vi "GetAdjacentFips.vi"(11 "FipsIn":i32[](array[numeric])) -> (3 "FipsOut":i32[](array[numeric]))   [LabVIEW 2017]
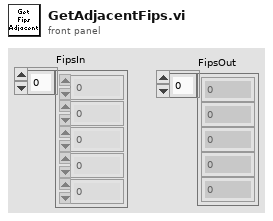
[diagram p1: front panel]
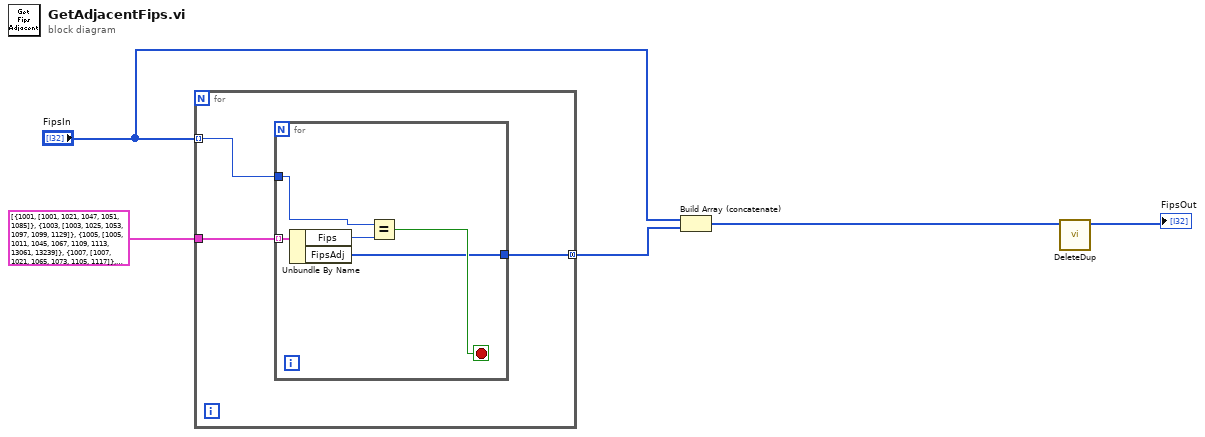
[diagram p0: block diagram]
diagram:
  n1 = for {
    tunnel: cluster{"Fips":i32, "FipsAdj":i32[]}[] [{"Fips"=1001, "FipsAdj"=[1001, 1021, 1047, 1051, 1085]}, {"Fips"=1003, "FipsAdj"=[1003, 1025, 1053, 1097, 1099, 1129]}, {"Fips"=1005, "FipsAdj"=[1005, 1011, 1045, 1067, 1109, 1113, 13061, 13239]}, {"Fips"=1007, "FipsAdj"=[1007, 1021, 1065, 1073, 1105, 1117]}, {"Fips"=1009, "FipsAdj"=[1009, 1043, 1055, 1073, 1095, 1115]}, {"Fips"=1011, "FipsAdj"=[1005, 1011, 1087, 1101, 1109]}, {"Fips"=1013, "FipsAdj"=[1013, 1035, 1039, 1041, 1085, 1099]}, {"Fips"=1015, "FipsAdj"=[1015, 1019, 1029, 1055, 1115]}, {"Fips"=1017, "FipsAdj"=[1017, 1081, 1111, 1123, 13145]}, {"Fips"=1019, "FipsAdj"=[1015, 1019, 1029, 1049, 1055, 13055, 13115]}, {"Fips"=1021, "FipsAdj"=[1001, 1007, 1021, 1037, 1047, 1051, 1105]}, {"Fips"=1023, "FipsAdj"=[1023, 1025, 1091, 1119, 1129, 28023, 28075]}, {"Fips"=1025, "FipsAdj"=[1003, 1023, 1025, 1091, 1099, 1129]}, {"Fips"=1027, "FipsAdj"=[1027, 1029, 1037, 1111, 1121]}, {"Fips"=1029, "FipsAdj"=[1015, 1019, 1027, 1029, 1111, 1121, 13045, 13143]}, {"Fips"=1031, "FipsAdj"=[1031, 1039, 1041, 1045, 1061]}, {"Fips"=1033, "FipsAdj"=[1033, 1059, 1077, 1079]}, {"Fips"=1035, "FipsAdj"=[1013, 1035, 1039, 1053]}, {"Fips"=1037, "FipsAdj"=[1021, 1027, 1037, 1051, 1117, 1121]}, {"Fips"=1039, "FipsAdj"=[1013, 1031, 1035, 1039, 1041, 1053, 1061, 12091]}, {"Fips"=1041, "FipsAdj"=[1013, 1031, 1039, 1041, 1085, 1101]}, {"Fips"=1043, "FipsAdj"=[1009, 1043, 1079, 1095, 1103, 1127]}, {"Fips"=1045, "FipsAdj"=[1005, 1031, 1045, 1061, 1067, 1069]}, {"Fips"=1047, "FipsAdj"=[1001, 1021, 1047, 1085, 1091, 1105]}, {"Fips"=1049, "FipsAdj"=[1019, 1049, 1055, 1071, 1095, 13055, 13083]}, {"Fips"=1051, "FipsAdj"=[1001, 1021, 1037, 1051, 1087, 1101]}, {"Fips"=1053, "FipsAdj"=[1003, 1035, 1039, 1053, 1099, 12033, 12091]}, {"Fips"=1055, "FipsAdj"=[1009, 1015, 1019, 1049, 1055, 1095]}, {"Fips"=1057, "FipsAdj"=[1057, 1075, 1093, 1107, 1125]}, {"Fips"=1059, "FipsAdj"=[1033, 1059, 1079, 1093, 1133, 28057]}, {"Fips"=1061, "FipsAdj"=[1031, 1039, 1045, 1061, 1069, 12059, 12063]}, {"Fips"=1063, "FipsAdj"=[1063, 1065, 1091, 1107, 1119]}, {"Fips"=1065, "FipsAdj"=[1007, 1063, 1065, 1091, 1105]}, {"Fips"=1067, "FipsAdj"=[1005, 1045, 1067, 1069, 13061]}, {"Fips"=1069, "FipsAdj"=[1045, 1061, 1067, 1069, 12063, 13099]}, {"Fips"=1071, "FipsAdj"=[1049, 1071, 1089, 1095, 13083, 47051]}, {"Fips"=1073, "FipsAdj"=[1007, 1009, 1073, 1115, 1117, 1125]}, {"Fips"=1075, "FipsAdj"=[1057, 1075, 1093, 1107, 28087]}, {"Fips"=1077, "FipsAdj"=[1033, 1077, 1079, 1083, 28141, 47055, 47071, 47099]}, {"Fips"=1079, "FipsAdj"=[1033, 1043, 1059, 1077, 1079, 1083, 1103]}, {"Fips"=1081, "FipsAdj"=[1017, 1081, 1087, 1113, 1123, 13145]}, {"Fips"=1083, "FipsAdj"=[1077, 1079, 1083, 1089, 1103, 47055]}, {"Fips"=1085, "FipsAdj"=[1001, 1013, 1041, 1047, 1085, 1101]}, {"Fips"=1087, "FipsAdj"=[1011, 1051, 1081, 1087, 1101, 1113]}, {"Fips"=1089, "FipsAdj"=[1071, 1083, 1089, 1095, 1103, 47051]}, {"Fips"=1091, "FipsAdj"=[1023, 1025, 1047, 1063, 1065, 1091, 1105, 1119]}, {"Fips"=1093, "FipsAdj"=[1057, 1059, 1075, 1093, 1127, 1133, 28057]}, {"Fips"=1095, "FipsAdj"=[1009, 1043, 1049, 1055, 1071, 1089, 1095]}, {"Fips"=1097, "FipsAdj"=[1003, 1097, 1129, 28039, 28041]}, {"Fips"=1099, "FipsAdj"=[1003, 1013, 1025, 1035, 1053, 1099]}, {"Fips"=1101, "FipsAdj"=[1001, 1011, 1041, 1051, 1085, 1087, 1101]}, {"Fips"=1103, "FipsAdj"=[1043, 1079, 1083, 1089, 1095]}, {"Fips"=1105, "FipsAdj"=[1007, 1021, 1047, 1065, 1091]}, {"Fips"=1107, "FipsAdj"=[1057, 1063, 1075, 1107, 1119, 1125, 28087]}, {"Fips"=1109, "FipsAdj"=[1005, 1011, 1031, 1041, 1045, 1101]}, {"Fips"=1111, "FipsAdj"=[1017, 1027, 1029, 1111, 1123, 13045, 13149]}, {"Fips"=1113, "FipsAdj"=[1005, 1011, 1081, 1087, 1113, 13053, 13215]}, {"Fips"=1115, "FipsAdj"=[1009, 1015, 1055, 1073, 1115, 1117]}, {"Fips"=1117, "FipsAdj"=[1007, 1021, 1037, 1073, 1115, 1117]}, {"Fips"=1119, "FipsAdj"=[1023, 1063, 1091, 1107, 1119, 28069, 28075]}, {"Fips"=1121, "FipsAdj"=[1015, 1027, 1029, 1037, 1115, 1117]}, {"Fips"=1123, "FipsAdj"=[1017, 1027, 1037, 1051, 1081, 1087, 1111]}, {"Fips"=1125, "FipsAdj"=[1007, 1057, 1063, 1065, 1073, 1107, 1125]}, {"Fips"=1127, "FipsAdj"=[1009, 1043, 1057, 1073, 1093, 1125, 1127]}, {"Fips"=1129, "FipsAdj"=[1003, 1023, 1025, 1097, 1129, 28041]}, {"Fips"=1131, "FipsAdj"=[1013, 1025, 1047, 1085, 1091, 1099]}, {"Fips"=1133, "FipsAdj"=[1043, 1059, 1079, 1093, 1127]}, {"Fips"=2013, "FipsAdj"=[2013, 2016]}, {"Fips"=2016, "FipsAdj"=[2013]}, {"Fips"=2020, "FipsAdj"=[2020, 2122, 2170]}, {"Fips"=2050, "FipsAdj"=[2050, 2070, 2122, 2164, 2170, 2270]}, {"Fips"=2060, "FipsAdj"=[2060, 2070]}, {"Fips"=2068, "FipsAdj"=[2068, 2090, 2170, 2240]}, {"Fips"=2070, "FipsAdj"=[2050, 2060, 2070]}, {"Fips"=2090, "FipsAdj"=[2068, 2090, 2240]}, {"Fips"=2100, "FipsAdj"=[2100, 2105, 2110]}, {"Fips"=2105, "FipsAdj"=[2100, 2105, 2110, 2195, 2220]}, {"Fips"=2110, "FipsAdj"=[2100, 2105]}, {"Fips"=2122, "FipsAdj"=[2020, 2050, 2122, 2150, 2164, 2170]}, {"Fips"=2130, "FipsAdj"=[2130, 2198]}, {"Fips"=2150, "FipsAdj"=[2122, 2150]}, {"Fips"=2164, "FipsAdj"=[2013, 2050, 2060, 2070, 2122, 2150]}, {"Fips"=2170, "FipsAdj"=[2020, 2050, 2068, 2122, 2170, 2240, 2261]}, {"Fips"=2180, "FipsAdj"=[2180, 2188, 2270]}, {"Fips"=2185, "FipsAdj"=[2185, 2188]}, {"Fips"=2188, "FipsAdj"=[2180, 2185, 2188]}, {"Fips"=2195, "FipsAdj"=[2105, 2195, 2198, 2220]}, {"Fips"=2198, "FipsAdj"=[2130, 2195, 2198]}, {"Fips"=2220, "FipsAdj"=[2105, 2195]}, {"Fips"=2230, "FipsAdj"=[2100]}, {"Fips"=2240, "FipsAdj"=[2068, 2090, 2170, 2240, 2261]}, {"Fips"=2261, "FipsAdj"=[2020, 2122, 2170, 2240, 2261]}, {"Fips"=2270, "FipsAdj"=[2050, 2180, 2270]}, {"Fips"=2275, "FipsAdj"=[2130, 2195, 2198]}, {"Fips"=2282, "FipsAdj"=[2105, 2261]}, {"Fips"=2290, "FipsAdj"=[2050, 2068, 2090, 2170, 2180, 2185, 2188, 2240, 2270]}, {"Fips"=4001, "FipsAdj"=[4001, 4009, 4011, 4017, 8083, 35003, 35006, 35031, 35045]}, {"Fips"=4003, "FipsAdj"=[4003, 4009, 4011, 4019, 4023]}, {"Fips"=4005, "FipsAdj"=[4005, 4007, 4015, 4017, 4025, 49025]}, {"Fips"=4007, "FipsAdj"=[4005, 4007, 4009, 4013, 4017, 4021]}, {"Fips"=4009, "FipsAdj"=[4001, 4003, 4007, 4009, 4011, 4017, 4019]}, {"Fips"=4011, "FipsAdj"=[4001, 4003, 4009, 4011, 35003, 35017]}, {"Fips"=4012, "FipsAdj"=[4012, 4013, 4015, 4025, 4027, 6025, 6065]}, {"Fips"=4013, "FipsAdj"=[4007, 4012, 4013, 4019, 4021, 4025]}, {"Fips"=4015, "FipsAdj"=[4005, 4012, 4015, 4025, 6071, 32003, 32017, 49025]}, {"Fips"=4017, "FipsAdj"=[4001, 4005, 4007, 4009, 4017]}, {"Fips"=4019, "FipsAdj"=[4003, 4009, 4013, 4019, 4021, 4023]}, {"Fips"=4021, "FipsAdj"=[4007, 4009, 4013, 4019]}, {"Fips"=4023, "FipsAdj"=[4003, 4019]}, {"Fips"=4025, "FipsAdj"=[4005, 4007, 4012, 4013, 4015]}, {"Fips"=4027, "FipsAdj"=[4012, 4013, 4019, 4027]}, {"Fips"=5001, "FipsAdj"=[5001, 5041, 5069, 5079, 5085, 5095, 5107]}, {"Fips"=5003, "FipsAdj"=[5003, 5011, 5017, 5043, 5139, 22067]}, {"Fips"=5005, "FipsAdj"=[5005, 5049, 5065, 5089, 5129, 5137]}, {"Fips"=5007, "FipsAdj"=[5007, 5015, 5087, 5143, 29009, 29119, 40001]}, {"Fips"=5009, "FipsAdj"=[5009, 5015, 5089, 5101, 5129]}, {"Fips"=5011, "FipsAdj"=[5003, 5011, 5013, 5025, 5043]}, {"Fips"=5013, "FipsAdj"=[5011, 5013, 5025, 5039, 5103]}, {"Fips"=5015, "FipsAdj"=[5007, 5009, 5015, 5087, 5101, 29009, 29209]}, {"Fips"=5017, "FipsAdj"=[5003, 5017, 5041, 5043, 22035, 22067, 22123, 28011, 28055]}, {"Fips"=5019, "FipsAdj"=[5019, 5039, 5059, 5097, 5099, 5103]}, {"Fips"=5021, "FipsAdj"=[5021, 5055, 5121, 29023, 29069]}, {"Fips"=5023, "FipsAdj"=[5023, 5045, 5063, 5137, 5141]}, {"Fips"=5025, "FipsAdj"=[5011, 5013, 5025, 5039, 5043, 5053, 5069]}, {"Fips"=5027, "FipsAdj"=[5027, 5073, 5099, 5103, 5139, 22027]}, {"Fips"=5029, "FipsAdj"=[5029, 5045, 5105, 5115, 5141]}, {"Fips"=5031, "FipsAdj"=[5031, 5055, 5067, 5075, 5093, 5111]}, {"Fips"=5033, "FipsAdj"=[5033, 5047, 5087, 5131, 5143, 40001]}, {"Fips"=5035, "FipsAdj"=[5035, 5037, 5077, 5093, 5111, 5123, 28033, 28143, 47157]}, {"Fips"=5037, "FipsAdj"=[5035, 5037, 5067, 5111, 5123]}, {"Fips"=5039, "FipsAdj"=[5013, 5019, 5025, 5039, 5053, 5059]}, {"Fips"=5041, "FipsAdj"=[5001, 5017, 5041, 5043, 5079, 5107]}, {"Fips"=5043, "FipsAdj"=[5003, 5011, 5017, 5025, 5041, 5043]}, {"Fips"=5045, "FipsAdj"=[5023, 5029, 5045, 5085, 5105, 5119, 5141]}, {"Fips"=5047, "FipsAdj"=[5033, 5047, 5071, 5083, 5087]}, {"Fips"=5049, "FipsAdj"=[5005, 5049, 5065, 5135, 29091, 29149]}, {"Fips"=5051, "FipsAdj"=[5051, 5059, 5097, 5105, 5125]}, {"Fips"=5053, "FipsAdj"=[5025, 5039, 5053, 5059, 5069, 5119]}, {"Fips"=5055, "FipsAdj"=[5021, 5031, 5055, 5075, 5121]}, {"Fips"=5057, "FipsAdj"=[5057, 5061, 5073, 5081, 5091, 5099]}, {"Fips"=5059, "FipsAdj"=[5019, 5039, 5051, 5053, 5059, 5097]}, {"Fips"=5061, "FipsAdj"=[5057, 5061, 5081, 5097, 5109, 5113]}, {"Fips"=5063, "FipsAdj"=[5023, 5063, 5065, 5067, 5075, 5135, 5137]}, {"Fips"=5065, "FipsAdj"=[5005, 5049, 5063, 5065, 5135]}, {"Fips"=5067, "FipsAdj"=[5031, 5037, 5063, 5067, 5075, 5111, 5145]}, {"Fips"=5069, "FipsAdj"=[5001, 5025, 5053, 5069, 5079, 5085]}, {"Fips"=5071, "FipsAdj"=[5047, 5071, 5083, 5087, 5101]}, {"Fips"=5073, "FipsAdj"=[5027, 5057, 5073, 5091, 5099, 22015]}, {"Fips"=5075, "FipsAdj"=[5031, 5055, 5063, 5067, 5075, 5121]}, {"Fips"=5077, "FipsAdj"=[5035, 5077, 5095, 5107, 5123]}, {"Fips"=5079, "FipsAdj"=[5001, 5025, 5041, 5043, 5069]}, {"Fips"=5081, "FipsAdj"=[5057, 5061, 5081, 5091, 5133, 40089]}, {"Fips"=5083, "FipsAdj"=[5047, 5071, 5083, 5115, 5127, 5131]}, {"Fips"=5085, "FipsAdj"=[5001, 5045, 5069, 5085, 5117, 5119]}, {"Fips"=5087, "FipsAdj"=[5007, 5015, 5033, 5047, 5071, 5087, 5101]}, {"Fips"=5089, "FipsAdj"=[5005, 5009, 5089, 5129, 29153]}, {"Fips"=5091, "FipsAdj"=[5057, 5073, 5081, 5091, 22015, 22017, 48037]}, {"Fips"=5093, "FipsAdj"=[5031, 5035, 5093, 5111, 29069, 29155, 47045, 47097, 47157]}, {"Fips"=5095, "FipsAdj"=[5001, 5077, 5095, 5107, 5117, 5123]}, {"Fips"=5097, "FipsAdj"=[5019, 5051, 5059, 5061, 5097, 5109, 5113, 5127]}, {"Fips"=5099, "FipsAdj"=[5019, 5027, 5057, 5073, 5099, 5103]}, {"Fips"=5101, "FipsAdj"=[5009, 5015, 5071, 5087, 5101, 5115]}, {"Fips"=5103, "FipsAdj"=[5013, 5019, 5027, 5039, 5099, 5103]}, {"Fips"=5105, "FipsAdj"=[5029, 5045, 5051, 5105, 5119, 5125]}, {"Fips"=5107, "FipsAdj"=[5001, 5041, 5077, 5095, 5107, 28011, 28027]}, {"Fips"=5109, "FipsAdj"=[5019, 5057, 5061, 5097, 5099, 5109]}, {"Fips"=5111, "FipsAdj"=[5031, 5035, 5037, 5067, 5093]}, {"Fips"=5113, "FipsAdj"=[5061, 5097, 5109, 5113, 5127, 5133, 40079]}, {"Fips"=5115, "FipsAdj"=[5029, 5071, 5083, 5101, 5115, 5129, 5141]}, {"Fips"=5117, "FipsAdj"=[5001, 5085, 5095, 5117, 5145]}, {"Fips"=5119, "FipsAdj"=[5045, 5053, 5069, 5085, 5105, 5119]}, {"Fips"=5121, "FipsAdj"=[5021, 5055, 5075, 5121, 5135, 29149]}, {"Fips"=5123, "FipsAdj"=[5035, 5037, 5077, 5095, 5123]}, {"Fips"=5125, "FipsAdj"=[5051, 5053, 5059, 5105, 5119]}, {"Fips"=5127, "FipsAdj"=[5083, 5097, 5113, 5127, 5131, 5149]}, {"Fips"=5129, "FipsAdj"=[5005, 5009, 5089, 5101, 5115, 5129, 5137]}, {"Fips"=5131, "FipsAdj"=[5033, 5047, 5083, 5127, 5131, 40079]}, {"Fips"=5133, "FipsAdj"=[5061, 5081, 5113, 5133]}, {"Fips"=5135, "FipsAdj"=[5049, 5063, 5065, 5075, 5121, 5135]}, {"Fips"=5137, "FipsAdj"=[5005, 5023, 5063, 5065, 5129, 5137]}, {"Fips"=5139, "FipsAdj"=[5003, 5011, 5013, 5027, 5103, 5139, 22027, 22067]}, {"Fips"=5141, "FipsAdj"=[5023, 5029, 5045, 5115, 5129, 5137]}, {"Fips"=5143, "FipsAdj"=[5007, 5033, 5087, 5143]}, {"Fips"=5145, "FipsAdj"=[5023, 5045, 5063, 5067, 5085, 5117, 5145]}, {"Fips"=5147, "FipsAdj"=[5037, 5067, 5095, 5117, 5123, 5145]}, {"Fips"=5149, "FipsAdj"=[5029, 5051, 5083, 5097, 5105, 5115, 5127]}, {"Fips"=6001, "FipsAdj"=[6001, 6013, 6075, 6077, 6081, 6085]}, {"Fips"=6003, "FipsAdj"=[6003, 6005, 6009, 6017, 6051, 6109]}, {"Fips"=6005, "FipsAdj"=[6003, 6005, 6009, 6017, 6067]}, {"Fips"=6007, "FipsAdj"=[6007, 6011, 6021, 6063, 6101, 6103]}, {"Fips"=6009, "FipsAdj"=[6003, 6005, 6009, 6077, 6099]}, {"Fips"=6011, "FipsAdj"=[6007, 6011, 6021, 6033, 6101]}, {"Fips"=6013, "FipsAdj"=[6001, 6013, 6041, 6067, 6075, 6077, 6095]}, {"Fips"=6015, "FipsAdj"=[6015, 6023, 6093, 41015]}, {"Fips"=6017, "FipsAdj"=[6003, 6005, 6017, 6061, 6067]}, {"Fips"=6019, "FipsAdj"=[6019, 6027, 6031, 6039, 6047, 6051, 6053, 6069]}, {"Fips"=6021, "FipsAdj"=[6007, 6011, 6021, 6033, 6045]}, {"Fips"=6023, "FipsAdj"=[6015, 6023, 6045, 6093]}, {"Fips"=6025, "FipsAdj"=[4012, 4027, 6025, 6065]}, {"Fips"=6027, "FipsAdj"=[6019, 6027, 6029, 6051, 6071, 6107, 32003, 32009]}, {"Fips"=6029, "FipsAdj"=[6027, 6029, 6031, 6037, 6071, 6079, 6083, 6107]}, {"Fips"=6031, "FipsAdj"=[6019, 6029, 6031, 6053, 6079]}, {"Fips"=6033, "FipsAdj"=[6011, 6021, 6033, 6045, 6055, 6097]}, {"Fips"=6035, "FipsAdj"=[6035, 6049, 6063, 6089, 6091]}, {"Fips"=6037, "FipsAdj"=[6029, 6037, 6059, 6071]}, {"Fips"=6039, "FipsAdj"=[6019, 6039, 6043, 6047, 6051]}, {"Fips"=6041, "FipsAdj"=[6013, 6041, 6075, 6095]}, {"Fips"=6043, "FipsAdj"=[6039, 6043, 6047, 6099]}, {"Fips"=6045, "FipsAdj"=[6021, 6023, 6033, 6045, 6097, 6103]}, {"Fips"=6047, "FipsAdj"=[6019, 6039, 6043, 6047, 6069, 6085]}, {"Fips"=6049, "FipsAdj"=[6035, 6049, 6089, 6093, 32031, 41035]}, {"Fips"=6051, "FipsAdj"=[6003, 6019, 6027, 6039, 6051, 6109, 32005, 32009, 32019]}, {"Fips"=6053, "FipsAdj"=[6019, 6031, 6053, 6069, 6079]}, {"Fips"=6055, "FipsAdj"=[6033, 6055, 6095, 6097]}, {"Fips"=6057, "FipsAdj"=[6057, 6061, 6091, 6115]}, {"Fips"=6059, "FipsAdj"=[6037, 6059, 6065, 6071]}, {"Fips"=6061, "FipsAdj"=[6017, 6057, 6061, 6067, 6101, 6115, 32005, 32031]}, {"Fips"=6063, "FipsAdj"=[6007, 6035, 6063, 6089, 6091, 6103]}, {"Fips"=6065, "FipsAdj"=[4012, 6025, 6059, 6065, 6071]}, {"Fips"=6067, "FipsAdj"=[6005, 6013, 6017, 6061, 6067, 6077, 6095, 6101]}, {"Fips"=6069, "FipsAdj"=[6019, 6047, 6053, 6069, 6085]}, {"Fips"=6071, "FipsAdj"=[4012, 4015, 6027, 6029, 6037, 6059, 6065, 6071]}, {"Fips"=6073, "FipsAdj"=[6025, 6059, 6065]}, {"Fips"=6075, "FipsAdj"=[6001, 6013, 6041, 6075]}, {"Fips"=6077, "FipsAdj"=[6001, 6005, 6009, 6013, 6067, 6077]}, {"Fips"=6079, "FipsAdj"=[6029, 6031, 6053, 6079]}, {"Fips"=6081, "FipsAdj"=[6001, 6075, 6081, 6085]}, {"Fips"=6083, "FipsAdj"=[6029, 6079, 6083]}, {"Fips"=6085, "FipsAdj"=[6001, 6047, 6069, 6081, 6085, 6087]}, {"Fips"=6087, "FipsAdj"=[6053, 6069, 6081, 6085]}, {"Fips"=6089, "FipsAdj"=[6035, 6049, 6063, 6089, 6093, 6103]}, {"Fips"=6091, "FipsAdj"=[6035, 6057, 6063, 6091, 6115]}, {"Fips"=6093, "FipsAdj"=[6015, 6023, 6049, 6089, 6093, 6105, 41029, 41033]}, {"Fips"=6095, "FipsAdj"=[6013, 6041, 6055, 6067, 6095, 6097]}, {"Fips"=6097, "FipsAdj"=[6013, 6033, 6041, 6045, 6055, 6095]}, {"Fips"=6099, "FipsAdj"=[6001, 6009, 6043, 6047, 6077, 6085, 6099]}, {"Fips"=6101, "FipsAdj"=[6007, 6011, 6061, 6067, 6101, 6113]}, {"Fips"=6103, "FipsAdj"=[6007, 6021, 6045, 6063, 6089, 6103]}, {"Fips"=6105, "FipsAdj"=[6023, 6045, 6089, 6093, 6103]}, {"Fips"=6107, "FipsAdj"=[6019, 6027, 6029, 6031]}, {"Fips"=6109, "FipsAdj"=[6003, 6009, 6039, 6043, 6051, 6099]}, {"Fips"=6111, "FipsAdj"=[6029, 6037, 6083]}, {"Fips"=6113, "FipsAdj"=[6011, 6033, 6055, 6067, 6095, 6101]}, {"Fips"=6115, "FipsAdj"=[6007, 6057, 6061, 6063, 6091, 6101]}, {"Fips"=8001, "FipsAdj"=[8001, 8005, 8014, 8031, 8059, 8087, 8121]}, {"Fips"=8003, "FipsAdj"=[8003, 8021, 8023, 8055, 8105]}, {"Fips"=8005, "FipsAdj"=[8001, 8005, 8031, 8035, 8039, 8059, 8073]}, {"Fips"=8007, "FipsAdj"=[8007, 8021, 8053, 8067, 8079, 8105, 35039]}, {"Fips"=8009, "FipsAdj"=[8009, 8011, 8071, 8099, 20129, 20187, 35059]}, {"Fips"=8011, "FipsAdj"=[8009, 8011, 8061, 8071, 8089]}, {"Fips"=8013, "FipsAdj"=[8013, 8014, 8047, 8049, 8059, 8069]}, {"Fips"=8014, "FipsAdj"=[8001, 8013, 8014, 8059]}, {"Fips"=8015, "FipsAdj"=[8015, 8043, 8051, 8065, 8093, 8097]}, {"Fips"=8017, "FipsAdj"=[8017, 8061, 8063, 8073, 20071]}, {"Fips"=8019, "FipsAdj"=[8019, 8047, 8049, 8059, 8093]}, {"Fips"=8021, "FipsAdj"=[8003, 8007, 8021, 8023, 8105, 35039]}, {"Fips"=8023, "FipsAdj"=[8003, 8021, 8023, 8055, 8071, 35007]}, {"Fips"=8025, "FipsAdj"=[8025, 8041, 8061, 8073, 8089]}, {"Fips"=8027, "FipsAdj"=[8027, 8043, 8055, 8101]}, {"Fips"=8029, "FipsAdj"=[8029, 8051, 8077]}, {"Fips"=8031, "FipsAdj"=[8001, 8005, 8031]}, {"Fips"=8033, "FipsAdj"=[8033, 8067, 8083, 8111, 8113]}, {"Fips"=8035, "FipsAdj"=[8005, 8035, 8039, 8041, 8059]}, {"Fips"=8037, "FipsAdj"=[8037, 8045, 8049, 8065, 8097, 8107]}, {"Fips"=8039, "FipsAdj"=[8005, 8035, 8039, 8041]}, {"Fips"=8041, "FipsAdj"=[8025, 8035, 8039, 8041, 8043, 8073, 8101]}, {"Fips"=8043, "FipsAdj"=[8015, 8027, 8041, 8043, 8093, 8101, 8109]}, {"Fips"=8045, "FipsAdj"=[8037, 8045, 8077, 8097, 8103, 8107, 49019]}, {"Fips"=8047, "FipsAdj"=[8013, 8019, 8047, 8049]}, {"Fips"=8049, "FipsAdj"=[8013, 8019, 8037, 8047, 8049, 8057, 8069, 8107]}, {"Fips"=8051, "FipsAdj"=[8015, 8029, 8051, 8053, 8077, 8085, 8091, 8097]}, {"Fips"=8053, "FipsAdj"=[8007, 8051, 8053, 8067, 8079, 8091, 8109]}, {"Fips"=8055, "FipsAdj"=[8003, 8023, 8027, 8055, 8071, 8101]}, {"Fips"=8057, "FipsAdj"=[8049, 8057, 8069, 8107, 56001]}, {"Fips"=8059, "FipsAdj"=[8001, 8005, 8013, 8014, 8019, 8031, 8035, 8047, 8059, 8093]}, {"Fips"=8061, "FipsAdj"=[8011, 8017, 8025, 8061, 8073, 8089, 8099]}, {"Fips"=8063, "FipsAdj"=[8017, 8063, 8073, 8121, 8125, 20023, 20181]}, {"Fips"=8065, "FipsAdj"=[8015, 8037, 8065, 8093, 8097]}, {"Fips"=8067, "FipsAdj"=[8007, 8033, 8053, 8067, 8083, 8111]}, {"Fips"=8069, "FipsAdj"=[8013, 8049, 8057, 8069, 8123, 56001]}, {"Fips"=8071, "FipsAdj"=[8009, 8011, 8023, 8055, 8071, 8089, 8101, 35007]}, {"Fips"=8073, "FipsAdj"=[8005, 8017, 8025, 8039, 8041, 8061, 8063, 8073, 8101]}, {"Fips"=8075, "FipsAdj"=[8075, 8087, 8095, 8115, 8121, 8123, 8125, 31033]}, {"Fips"=8077, "FipsAdj"=[8029, 8045, 8051, 8077, 8085, 8097, 49019]}, {"Fips"=8079, "FipsAdj"=[8007, 8053, 8079, 8105]}, {"Fips"=8081, "FipsAdj"=[8081, 8103, 8107, 49009, 49047, 56007]}, {"Fips"=8083, "FipsAdj"=[4001, 8033, 8067, 8083, 8111, 35045]}, {"Fips"=8085, "FipsAdj"=[8029, 8051, 8077, 8085, 8091, 8113, 49019]}, {"Fips"=8087, "FipsAdj"=[8001, 8075, 8087, 8121]}, {"Fips"=8089, "FipsAdj"=[8011, 8025, 8061, 8071, 8089]}, {"Fips"=8091, "FipsAdj"=[8051, 8053, 8085, 8091, 8111]}, {"Fips"=8093, "FipsAdj"=[8015, 8019, 8043, 8059, 8065, 8093, 8117]}, {"Fips"=8095, "FipsAdj"=[8075, 8095, 8115, 8125, 31029]}, {"Fips"=8097, "FipsAdj"=[8015, 8037, 8045, 8051, 8065, 8077]}, {"Fips"=8099, "FipsAdj"=[8009, 8011, 8061, 8099, 20071, 20075]}, {"Fips"=8101, "FipsAdj"=[8025, 8027, 8041, 8043, 8055, 8071, 8073, 8089]}, {"Fips"=8103, "FipsAdj"=[8045, 8081, 8103, 8107]}, {"Fips"=8105, "FipsAdj"=[8003, 8007, 8021, 8079, 8105]}, {"Fips"=8107, "FipsAdj"=[8037, 8045, 8049, 8057, 8081, 8103, 8107]}, {"Fips"=8109, "FipsAdj"=[8003, 8015, 8027, 8043, 8051, 8053, 8055, 8079, 8105]}, {"Fips"=8111, "FipsAdj"=[8033, 8053, 8067, 8083, 8091, 8111]}, {"Fips"=8113, "FipsAdj"=[8033, 8085, 8091, 8111, 8113]}, {"Fips"=8115, "FipsAdj"=[8075, 8095, 8115, 31033, 31049]}, {"Fips"=8117, "FipsAdj"=[8019, 8037, 8049, 8065, 8093]}, {"Fips"=8119, "FipsAdj"=[8035, 8041, 8043, 8059, 8093]}, {"Fips"=8121, "FipsAdj"=[8001, 8005, 8063, 8073, 8075, 8087, 8121]}, {"Fips"=8123, "FipsAdj"=[8001, 8013, 8014, 8069, 8075, 8087, 8123, 31105]}, {"Fips"=8125, "FipsAdj"=[8063, 8075, 8095, 8121, 8125, 20023, 31029]}, {"Fips"=9001, "FipsAdj"=[9001, 9005, 9009, 36027, 36059, 36079, 36103]}, {"Fips"=9003, "FipsAdj"=[9003, 9005, 9007, 9009, 9011, 9013]}, {"Fips"=9005, "FipsAdj"=[9001, 9003, 9005, 9009, 25003, 25013]}, {"Fips"=9007, "FipsAdj"=[9003, 9007, 9009, 9011]}, {"Fips"=9009, "FipsAdj"=[9001, 9003, 9005, 9007, 9009]}, {"Fips"=9011, "FipsAdj"=[9003, 9007, 9011, 9013, 9015, 36103, 44003]}, {"Fips"=9013, "FipsAdj"=[9003, 9011, 9013, 9015, 25013]}, {"Fips"=9015, "FipsAdj"=[9011, 9013, 9015, 25027, 44003]}, {"Fips"=10001, "FipsAdj"=[10001, 10003, 10005, 24011, 24029, 24035, 34009, 34011]}, {"Fips"=10003, "FipsAdj"=[10001, 10003, 24015, 24029, 34015, 34033, 42029]}, {"Fips"=10005, "FipsAdj"=[10001, 10005, 24011, 24019, 24045, 24047]}, {"Fips"=11001, "FipsAdj"=[11001, 24031, 24033, 51013, 51059]}, {"Fips"=12001, "FipsAdj"=[12001, 12007, 12023, 12041, 12075, 12083, 12107]}, {"Fips"=12003, "FipsAdj"=[12003, 12007, 12019, 12023, 12031, 12089, 12125, 13049, 13065]}, {"Fips"=12005, "FipsAdj"=[12005, 12013, 12045, 12063, 12131]}, {"Fips"=12007, "FipsAdj"=[12001, 12003, 12007, 12019, 12107]}, {"Fips"=12009, "FipsAdj"=[12009, 12061, 12095, 12097, 12117]}, {"Fips"=12011, "FipsAdj"=[12011, 12021, 12051, 12086]}, {"Fips"=12013, "FipsAdj"=[12005, 12013, 12039, 12045, 12063]}, {"Fips"=12015, "FipsAdj"=[12015, 12027, 12043, 12051, 12055, 12071]}, {"Fips"=12017, "FipsAdj"=[12017, 12053, 12075, 12083]}, {"Fips"=12019, "FipsAdj"=[12003, 12007, 12019, 12031, 12107]}, {"Fips"=12021, "FipsAdj"=[12011, 12021, 12051, 12071, 12086]}, {"Fips"=12023, "FipsAdj"=[12001, 12003, 12023, 12041, 12047, 12121, 12125, 13065]}, {"Fips"=12027, "FipsAdj"=[12015, 12027, 12043, 12049, 12055, 12081]}, {"Fips"=12029, "FipsAdj"=[12029, 12041, 12067, 12075]}, {"Fips"=12031, "FipsAdj"=[12003, 12019, 12031, 12089]}, {"Fips"=12033, "FipsAdj"=[1003, 1053, 12033]}, {"Fips"=12035, "FipsAdj"=[12035, 12107, 12109]}, {"Fips"=12037, "FipsAdj"=[12037, 12045, 12077]}, {"Fips"=12039, "FipsAdj"=[12013, 12039, 12063, 12073, 12077, 13087, 13131]}, {"Fips"=12041, "FipsAdj"=[12001, 12023, 12029, 12041, 12067, 12075]}, {"Fips"=12043, "FipsAdj"=[12015, 12027, 12043, 12051, 12055, 12071, 12085, 12093]}, {"Fips"=12045, "FipsAdj"=[12005, 12013, 12037, 12045]}, {"Fips"=12047, "FipsAdj"=[12023, 12047, 12079, 12121, 13027, 13101]}, {"Fips"=12049, "FipsAdj"=[12027, 12049, 12055, 12057, 12081]}, {"Fips"=12051, "FipsAdj"=[12011, 12015, 12021, 12043, 12051, 12071, 12085, 12093]}, {"Fips"=12053, "FipsAdj"=[12017, 12053, 12101]}, {"Fips"=12055, "FipsAdj"=[12015, 12027, 12043, 12049, 12055, 12093, 12097]}, {"Fips"=12057, "FipsAdj"=[12049, 12057, 12081, 12101, 12103]}, {"Fips"=12059, "FipsAdj"=[1061, 12059, 12063, 12131]}, {"Fips"=12061, "FipsAdj"=[12009, 12061, 12093, 12097]}, {"Fips"=12063, "FipsAdj"=[1061, 1069, 12005, 12013, 12039, 12059, 12063, 12077, 12133]}, {"Fips"=12065, "FipsAdj"=[12065, 12073, 12079, 12123, 12129, 13027]}, {"Fips"=12067, "FipsAdj"=[12029, 12041, 12067, 12079, 12121]}, {"Fips"=12069, "FipsAdj"=[12069, 12083, 12095, 12097, 12105, 12117, 12119]}, {"Fips"=12071, "FipsAdj"=[12015, 12021, 12043, 12051]}, {"Fips"=12073, "FipsAdj"=[12039, 12065, 12073, 12077, 12129, 13131]}, {"Fips"=12075, "FipsAdj"=[12001, 12017, 12029, 12041, 12075]}, {"Fips"=12077, "FipsAdj"=[12013, 12037, 12039, 12045, 12063, 12073, 12077]}, {"Fips"=12079, "FipsAdj"=[12047, 12065, 12067, 12079, 12121, 12123, 13027]}, {"Fips"=12081, "FipsAdj"=[12027, 12049, 12057, 12081, 12105]}, {"Fips"=12083, "FipsAdj"=[12001, 12017, 12069, 12075, 12083, 12107, 12119]}, {"Fips"=12085, "FipsAdj"=[12043, 12051, 12085, 12093, 12099]}, {"Fips"=12086, "FipsAdj"=[12011, 12021, 12086]}, {"Fips"=12087, "FipsAdj"=[12021, 12086]}, {"Fips"=12089, "FipsAdj"=[12003, 12031, 12089, 13039]}, {"Fips"=12091, "FipsAdj"=[1039, 1053, 12091, 12113]}, {"Fips"=12093, "FipsAdj"=[12043, 12051, 12055, 12061, 12085, 12093, 12097, 12099, 12105]}, {"Fips"=12095, "FipsAdj"=[12009, 12069, 12095, 12097, 12105, 12117]}, {"Fips"=12097, "FipsAdj"=[12009, 12055, 12061, 12069, 12093, 12095, 12097]}, {"Fips"=12099, "FipsAdj"=[12011, 12043, 12051, 12085, 12093]}, {"Fips"=12101, "FipsAdj"=[12053, 12057, 12101, 12103, 12105]}, {"Fips"=12103, "FipsAdj"=[12057, 12101]}, {"Fips"=12105, "FipsAdj"=[12049, 12055, 12057, 12069, 12081, 12093, 12095, 12097, 12101, 12105]}, {"Fips"=12107, "FipsAdj"=[12001, 12007, 12019, 12035, 12083, 12107, 12109]}, {"Fips"=12109, "FipsAdj"=[12019, 12031, 12035, 12107]}, {"Fips"=12111, "FipsAdj"=[12061, 12085, 12093]}, {"Fips"=12113, "FipsAdj"=[1053, 12033, 12091]}, {"Fips"=12115, "FipsAdj"=[12015, 12027, 12081]}, {"Fips"=12117, "FipsAdj"=[12009, 12069, 12095, 12117]}, {"Fips"=12119, "FipsAdj"=[12017, 12053, 12069, 12083, 12101, 12105]}, {"Fips"=12121, "FipsAdj"=[12023, 12041, 12047, 12067, 12079]}, {"Fips"=12123, "FipsAdj"=[12029, 12065, 12067, 12079]}, {"Fips"=12125, "FipsAdj"=[12001, 12003, 12007, 12023]}, {"Fips"=12127, "FipsAdj"=[12009, 12035, 12069, 12083, 12095, 12107, 12117]}, {"Fips"=12129, "FipsAdj"=[12037, 12065, 12073, 12077]}, {"Fips"=12131, "FipsAdj"=[1039, 1061, 12005, 12059, 12091, 12131]}, {"Fips"=12133, "FipsAdj"=[12005, 12059, 12063, 12131]}, {"Fips"=13001, "FipsAdj"=[13001, 13005, 13161, 13229, 13267, 13279]}, {"Fips"=13003, "FipsAdj"=[13003, 13019, 13065, 13069, 13173]}, {"Fips"=13005, "FipsAdj"=[13001, 13005, 13069, 13161, 13229]}, {"Fips"=13007, "FipsAdj"=[13007, 13037, 13087, 13095, 13099, 13201]}, {"Fips"=13009, "FipsAdj"=[13009, 13141, 13169, 13237, 13303]}, {"Fips"=13011, "FipsAdj"=[13011, 13119, 13137, 13139, 13157, 13195]}, {"Fips"=13013, "FipsAdj"=[13013, 13059, 13135, 13139, 13157, 13219]}, {"Fips"=13015, "FipsAdj"=[13015, 13057, 13067, 13115, 13129, 13223, 13227]}, {"Fips"=13017, "FipsAdj"=[13017, 13069, 13155, 13271, 13287]}, {"Fips"=13019, "FipsAdj"=[13003, 13019, 13069, 13075, 13155, 13173, 13185]}, {"Fips"=13021, "FipsAdj"=[13021, 13079, 13153, 13169, 13207]}, {"Fips"=13023, "FipsAdj"=[13023, 13091, 13153, 13175, 13235, 13289]}, {"Fips"=13025, "FipsAdj"=[13025, 13039, 13049, 13127, 13229, 13299]}, {"Fips"=13027, "FipsAdj"=[12047, 12065, 12079, 13027, 13071, 13075, 13185]}, {"Fips"=13029, "FipsAdj"=[13029, 13031, 13051, 13103, 13109]}, {"Fips"=13031, "FipsAdj"=[13029, 13031, 13043, 13103, 13107, 13109, 13165]}, {"Fips"=13033, "FipsAdj"=[13033, 13107, 13163, 13165, 13245, 13251, 45003, 45005]}, {"Fips"=13035, "FipsAdj"=[13035, 13151, 13159, 13171, 13207, 13217]}, {"Fips"=13037, "FipsAdj"=[13007, 13037, 13061, 13095, 13099, 13243]}, {"Fips"=13039, "FipsAdj"=[12089, 13025, 13039, 13049]}, {"Fips"=13043, "FipsAdj"=[13031, 13043, 13107, 13109, 13267]}, {"Fips"=13045, "FipsAdj"=[1029, 1111, 13045, 13077, 13097, 13121, 13143, 13149]}, {"Fips"=13047, "FipsAdj"=[13047, 13295, 13313]}, {"Fips"=13049, "FipsAdj"=[12003, 12089, 13025, 13039, 13049]}, {"Fips"=13051, "FipsAdj"=[13029, 13051, 13103, 13179]}, {"Fips"=13053, "FipsAdj"=[1113, 13053, 13197, 13215, 13259]}, {"Fips"=13055, "FipsAdj"=[1019, 1049, 13055, 13115]}, {"Fips"=13057, "FipsAdj"=[13015, 13057, 13067, 13085, 13117, 13121, 13129]}, {"Fips"=13059, "FipsAdj"=[13013, 13059, 13157, 13195, 13219]}, {"Fips"=13061, "FipsAdj"=[1005, 1067, 13037, 13061, 13099, 13239]}, {"Fips"=13063, "FipsAdj"=[13063, 13089, 13113, 13121, 13151]}, {"Fips"=13065, "FipsAdj"=[12003, 12023, 13003, 13065, 13101, 13173]}, {"Fips"=13067, "FipsAdj"=[13015, 13057, 13067, 13097, 13121]}, {"Fips"=13069, "FipsAdj"=[13003, 13005, 13017, 13019, 13069, 13155, 13161, 13271]}, {"Fips"=13071, "FipsAdj"=[13027, 13071, 13075, 13205, 13275, 13277]}, {"Fips"=13073, "FipsAdj"=[13073, 13181, 13189, 13245, 45037]}, {"Fips"=13075, "FipsAdj"=[13019, 13027, 13071, 13075, 13185]}, {"Fips"=13077, "FipsAdj"=[13045, 13077, 13113, 13121, 13149, 13199, 13255]}, {"Fips"=13079, "FipsAdj"=[13021, 13079, 13153, 13193, 13207, 13225, 13269]}, {"Fips"=13081, "FipsAdj"=[13081, 13093, 13177, 13261, 13287, 13315]}, {"Fips"=13083, "FipsAdj"=[1049, 1071, 13083, 13295, 47065]}, {"Fips"=13085, "FipsAdj"=[13057, 13085, 13111, 13117, 13123, 13139, 13187]}, {"Fips"=13087, "FipsAdj"=[12039, 13007, 13087, 13131, 13201, 13205]}, {"Fips"=13089, "FipsAdj"=[13063, 13089, 13121, 13135, 13151]}, {"Fips"=13091, "FipsAdj"=[13023, 13091, 13175, 13235, 13271, 13309]}, {"Fips"=13093, "FipsAdj"=[13081, 13093, 13153, 13193, 13235, 13261]}, {"Fips"=13095, "FipsAdj"=[13007, 13037, 13095, 13177, 13205, 13273]}, {"Fips"=13097, "FipsAdj"=[13045, 13067, 13097, 13121]}, {"Fips"=13099, "FipsAdj"=[1067, 1069, 13007, 13037, 13061, 13099, 13201]}, {"Fips"=13101, "FipsAdj"=[12023, 12047, 13065, 13101, 13173]}, {"Fips"=13103, "FipsAdj"=[13029, 13031, 13051, 13103, 13251, 45049]}, {"Fips"=13105, "FipsAdj"=[13105, 13147, 13181, 13195, 13221, 13317, 45001, 45007]}, {"Fips"=13107, "FipsAdj"=[13031, 13033, 13043, 13107, 13163, 13165, 13167, 13175, 13267, 13279]}, {"Fips"=13109, "FipsAdj"=[13029, 13031, 13043, 13109, 13179]}, {"Fips"=13111, "FipsAdj"=[13085, 13111, 13123, 13187, 13213, 13291, 37039]}, {"Fips"=13113, "FipsAdj"=[13063, 13077, 13113, 13121]}, {"Fips"=13115, "FipsAdj"=[1019, 13015, 13055, 13115, 13129, 13233]}, {"Fips"=13117, "FipsAdj"=[13057, 13085, 13117, 13121, 13135]}, {"Fips"=13119, "FipsAdj"=[13011, 13119, 13147, 13195, 13257]}, {"Fips"=13121, "FipsAdj"=[13045, 13057, 13063, 13067, 13077, 13089, 13097, 13113, 13117, 13121]}, {"Fips"=13123, "FipsAdj"=[13085, 13111, 13123, 13129, 13213]}, {"Fips"=13125, "FipsAdj"=[13125, 13141, 13163, 13301]}, {"Fips"=13127, "FipsAdj"=[13025, 13039, 13127, 13191]}, {"Fips"=13129, "FipsAdj"=[13015, 13057, 13115, 13123, 13129, 13213, 13227, 13295]}, {"Fips"=13131, "FipsAdj"=[12039, 12073, 13087, 13131, 13205]}, {"Fips"=13133, "FipsAdj"=[13133, 13141, 13211, 13219, 13221, 13237]}, {"Fips"=13135, "FipsAdj"=[13013, 13089, 13117, 13121, 13135, 13139, 13157, 13247]}, {"Fips"=13137, "FipsAdj"=[13011, 13137, 13139, 13241, 13257, 13281, 13311]}, {"Fips"=13139, "FipsAdj"=[13011, 13013, 13085, 13117, 13135, 13137, 13139, 13157, 13187]}, {"Fips"=13141, "FipsAdj"=[13009, 13125, 13133, 13141, 13237, 13265, 13301]}, {"Fips"=13143, "FipsAdj"=[1029, 13045, 13143, 13223]}, {"Fips"=13145, "FipsAdj"=[1017, 1081, 13145, 13199, 13215, 13263]}, {"Fips"=13147, "FipsAdj"=[13105, 13119, 13147, 13195, 45007]}, {"Fips"=13149, "FipsAdj"=[1111, 13045, 13077, 13149]}, {"Fips"=13151, "FipsAdj"=[13035, 13063, 13089, 13151, 13217, 13247]}, {"Fips"=13153, "FipsAdj"=[13021, 13023, 13079, 13093, 13153, 13193, 13225, 13235]}, {"Fips"=13155, "FipsAdj"=[13017, 13019, 13069, 13155, 13277]}, {"Fips"=13157, "FipsAdj"=[13011, 13013, 13059, 13135, 13139, 13157, 13195]}, {"Fips"=13159, "FipsAdj"=[13035, 13159, 13169, 13207, 13211, 13217]}, {"Fips"=13161, "FipsAdj"=[13001, 13005, 13069, 13161, 13209, 13271, 13279]}, {"Fips"=13163, "FipsAdj"=[13033, 13107, 13125, 13163, 13167, 13189, 13245, 13301]}, {"Fips"=13165, "FipsAdj"=[13031, 13033, 13107, 13165]}, {"Fips"=13167, "FipsAdj"=[13107, 13163, 13167, 13175, 13283, 13303]}, {"Fips"=13169, "FipsAdj"=[13009, 13021, 13159, 13169, 13207, 13237, 13289]}, {"Fips"=13171, "FipsAdj"=[13035, 13171, 13207, 13231, 13255]}, {"Fips"=13173, "FipsAdj"=[13003, 13019, 13065, 13101, 13173]}, {"Fips"=13175, "FipsAdj"=[13023, 13091, 13107, 13167, 13175, 13283, 13289, 13309]}, {"Fips"=13177, "FipsAdj"=[13081, 13095, 13177, 13261, 13273]}, {"Fips"=13179, "FipsAdj"=[13029, 13051, 13109, 13179, 13183, 13191]}, {"Fips"=13181, "FipsAdj"=[13073, 13105, 13181, 13189, 13317]}, {"Fips"=13183, "FipsAdj"=[13179, 13183, 13191, 13267]}, {"Fips"=13185, "FipsAdj"=[12047, 12079, 13019, 13027, 13075, 13101, 13173]}, {"Fips"=13187, "FipsAdj"=[13085, 13111, 13139, 13187, 13291]}, {"Fips"=13189, "FipsAdj"=[13073, 13163, 13181, 13189, 13245, 13301]}, {"Fips"=13191, "FipsAdj"=[13127, 13179, 13183, 13191]}, {"Fips"=13193, "FipsAdj"=[13079, 13093, 13153, 13193, 13225, 13249, 13261]}, {"Fips"=13195, "FipsAdj"=[13011, 13059, 13105, 13119, 13147, 13157, 13195]}, {"Fips"=13197, "FipsAdj"=[13053, 13197, 13249, 13259, 13261, 13263, 13269]}, {"Fips"=13199, "FipsAdj"=[13077, 13145, 13199, 13231, 13255, 13263, 13285]}, {"Fips"=13201, "FipsAdj"=[13007, 13087, 13099, 13201]}, {"Fips"=13205, "FipsAdj"=[13007, 13071, 13087, 13095, 13131, 13205, 13275]}, {"Fips"=13207, "FipsAdj"=[13021, 13035, 13079, 13159, 13169, 13171, 13207]}, {"Fips"=13209, "FipsAdj"=[13161, 13209, 13279, 13283]}, {"Fips"=13211, "FipsAdj"=[13133, 13159, 13211, 13217, 13219, 13237]}, {"Fips"=13213, "FipsAdj"=[13111, 13123, 13129, 13213, 13313, 47011]}, {"Fips"=13215, "FipsAdj"=[1081, 1113, 13053, 13145, 13215]}, {"Fips"=13217, "FipsAdj"=[13035, 13151, 13159, 13211, 13217, 13247]}, {"Fips"=13219, "FipsAdj"=[13013, 13059, 13133, 13157, 13211, 13219, 13221]}, {"Fips"=13221, "FipsAdj"=[13059, 13105, 13133, 13195, 13219, 13221, 13265]}, {"Fips"=13223, "FipsAdj"=[13015, 13045, 13067, 13097, 13143, 13223]}, {"Fips"=13225, "FipsAdj"=[13079, 13153, 13193, 13225]}, {"Fips"=13227, "FipsAdj"=[13015, 13057, 13085, 13123, 13129]}, {"Fips"=13229, "FipsAdj"=[13001, 13005, 13025, 13229, 13299]}, {"Fips"=13231, "FipsAdj"=[13171, 13199, 13231, 13255]}, {"Fips"=13233, "FipsAdj"=[1019, 1029, 13015, 13115, 13143, 13223]}, {"Fips"=13235, "FipsAdj"=[13023, 13091, 13093, 13153, 13235]}, {"Fips"=13237, "FipsAdj"=[13009, 13133, 13141, 13159, 13169, 13211]}, {"Fips"=13239, "FipsAdj"=[1005, 13061, 13239, 13243]}, {"Fips"=13241, "FipsAdj"=[13137, 13241, 13281, 37043, 37099, 37113]}, {"Fips"=13243, "FipsAdj"=[13037, 13061, 13239, 13243, 13259, 13273]}, {"Fips"=13245, "FipsAdj"=[13033, 13073, 13163, 13189, 13245, 45003]}, {"Fips"=13247, "FipsAdj"=[13089, 13135, 13151, 13217, 13247]}, {"Fips"=13249, "FipsAdj"=[13193, 13197, 13249, 13261]}, {"Fips"=13251, "FipsAdj"=[13031, 13033, 13103, 13165, 13251, 45005]}, {"Fips"=13253, "FipsAdj"=[1069, 12039, 12063, 13087, 13099, 13201]}, {"Fips"=13255, "FipsAdj"=[13035, 13063, 13077, 13113, 13151, 13171, 13199, 13231]}, {"Fips"=13257, "FipsAdj"=[13011, 13119, 13137, 13257]}, {"Fips"=13259, "FipsAdj"=[1005, 1113, 13053, 13197, 13239, 13243, 13259]}, {"Fips"=13261, "FipsAdj"=[13081, 13093, 13177, 13193, 13197, 13249, 13261, 13273]}, {"Fips"=13263, "FipsAdj"=[13053, 13145, 13197, 13199, 13215, 13263, 13269]}, {"Fips"=13265, "FipsAdj"=[13133, 13141, 13221, 13265, 13301]}, {"Fips"=13267, "FipsAdj"=[13001, 13043, 13107, 13109, 13179, 13183, 13267, 13279]}, {"Fips"=13269, "FipsAdj"=[13079, 13193, 13197, 13225, 13249, 13263, 13269]}, {"Fips"=13271, "FipsAdj"=[13017, 13069, 13091, 13161, 13271, 13309]}, {"Fips"=13273, "FipsAdj"=[13037, 13095, 13177, 13243, 13261, 13273]}, {"Fips"=13275, "FipsAdj"=[12065, 12073, 13027, 13071, 13131, 13205]}, {"Fips"=13277, "FipsAdj"=[13019, 13071, 13075, 13155, 13277, 13287]}, {"Fips"=13279, "FipsAdj"=[13001, 13043, 13107, 13161, 13209, 13267, 13279]}, {"Fips"=13281, "FipsAdj"=[13137, 13241, 13281, 13291, 13311]}, {"Fips"=13283, "FipsAdj"=[13107, 13167, 13175, 13209, 13279, 13283]}, {"Fips"=13285, "FipsAdj"=[1017, 1111, 13077, 13145, 13149, 13199]}, {"Fips"=13287, "FipsAdj"=[13017, 13081, 13155, 13277, 13287, 13315]}, {"Fips"=13289, "FipsAdj"=[13021, 13023, 13153, 13169, 13175, 13289]}, {"Fips"=13291, "FipsAdj"=[13111, 13187, 13281, 13291, 13311, 37039]}, {"Fips"=13293, "FipsAdj"=[13079, 13171, 13199, 13207, 13231, 13263, 13269]}, {"Fips"=13295, "FipsAdj"=[1049, 13047, 13055, 13083, 13115, 13129, 13295, 13313]}, {"Fips"=13297, "FipsAdj"=[13013, 13135, 13211, 13217, 13219, 13247]}, {"Fips"=13299, "FipsAdj"=[12003, 13003, 13005, 13025, 13049, 13065, 13069, 13229]}, {"Fips"=13301, "FipsAdj"=[13125, 13141, 13163, 13189, 13265, 13301]}, {"Fips"=13303, "FipsAdj"=[13009, 13125, 13141, 13163, 13167, 13303]}, {"Fips"=13305, "FipsAdj"=[13001, 13025, 13127, 13183, 13191, 13229, 13267]}, {"Fips"=13307, "FipsAdj"=[13197, 13243, 13259, 13261, 13273]}, {"Fips"=13309, "FipsAdj"=[13091, 13161, 13175, 13209, 13271, 13283]}, {"Fips"=13311, "FipsAdj"=[13137, 13139, 13187, 13281, 13291]}, {"Fips"=13313, "FipsAdj"=[13047, 13129, 13213, 13295, 13313, 47011]}, {"Fips"=13315, "FipsAdj"=[13017, 13081, 13091, 13093, 13235, 13271, 13287]}, {"Fips"=13317, "FipsAdj"=[13105, 13181, 13189, 13221, 13265, 13301]}, {"Fips"=13319, "FipsAdj"=[13009, 13023, 13167, 13169, 13175, 13289, 13303]}, {"Fips"=13321, "FipsAdj"=[13071, 13081, 13095, 13177, 13205, 13277, 13287]}, {"Fips"=15001, "FipsAdj"=[]}, {"Fips"=15003, "FipsAdj"=[]}, {"Fips"=15005, "FipsAdj"=[15005]}, {"Fips"=15007, "FipsAdj"=[]}, {"Fips"=15009, "FipsAdj"=[15005]}, {"Fips"=16001, "FipsAdj"=[16001, 16015, 16027, 16039, 16045]}, {"Fips"=16003, "FipsAdj"=[16003, 16045, 16049, 16085, 16087, 41001]}, {"Fips"=16005, "FipsAdj"=[16005, 16011, 16029, 16041, 16071]}, {"Fips"=16007, "FipsAdj"=[16007, 16029, 16041, 49005, 49033]}, {"Fips"=16009, "FipsAdj"=[16009, 16055, 16057, 16079, 53063]}, {"Fips"=16011, "FipsAdj"=[16005, 16011, 16013, 16019, 16023, 16029, 16051]}, {"Fips"=16013, "FipsAdj"=[16011, 16013, 16023, 16025, 16031, 16037, 16039, 16063, 16067]}, {"Fips"=16015, "FipsAdj"=[16001, 16015, 16037, 16039, 16045]}, {"Fips"=16017, "FipsAdj"=[16017, 16021, 16055, 16079, 30053, 30089, 53051]}, {"Fips"=16019, "FipsAdj"=[16011, 16019, 16029, 16051, 16065, 16081, 56023]}, {"Fips"=16021, "FipsAdj"=[16017, 16021, 30053]}, {"Fips"=16023, "FipsAdj"=[16011, 16013, 16023, 16033, 16037, 16051]}, {"Fips"=16025, "FipsAdj"=[16013, 16025, 16039, 16047]}, {"Fips"=16027, "FipsAdj"=[16001, 16027, 16045, 16073, 16075]}, {"Fips"=16029, "FipsAdj"=[16005, 16007, 16011, 16019, 16029, 16041]}, {"Fips"=16031, "FipsAdj"=[16013, 16031, 16053, 16067, 16071, 16077, 16083, 32007]}, {"Fips"=16033, "FipsAdj"=[16023, 16033, 16043, 16051, 16059]}, {"Fips"=16035, "FipsAdj"=[16035, 16049, 16057, 16061, 16069, 16079, 30061]}, {"Fips"=16037, "FipsAdj"=[16013, 16015, 16023, 16037, 16039, 16059]}, {"Fips"=16039, "FipsAdj"=[16001, 16013, 16015, 16025, 16037, 16039, 16047, 16073]}, {"Fips"=16041, "FipsAdj"=[16005, 16007, 16029, 16041, 16071, 49005]}, {"Fips"=16043, "FipsAdj"=[16033, 16043, 16051, 16065, 16081, 30001, 30031, 30057]}, {"Fips"=16045, "FipsAdj"=[16001, 16003, 16015, 16027, 16045, 16075, 16085]}, {"Fips"=16047, "FipsAdj"=[16025, 16039, 16047, 16053, 16063]}, {"Fips"=16049, "FipsAdj"=[16003, 16035, 16049, 16059, 16061, 16069, 16085, 30063, 30081]}, {"Fips"=16051, "FipsAdj"=[16011, 16019, 16023, 16033, 16043, 16051]}, {"Fips"=16053, "FipsAdj"=[16031, 16047, 16053, 16063, 16067]}, {"Fips"=16055, "FipsAdj"=[16009, 16017, 16055, 16079]}, {"Fips"=16057, "FipsAdj"=[16009, 16035, 16057, 16069, 16079]}, {"Fips"=16059, "FipsAdj"=[16023, 16033, 16037, 16049, 16059, 16085, 30001]}, {"Fips"=16061, "FipsAdj"=[16035, 16049, 16061]}, {"Fips"=16063, "FipsAdj"=[16013, 16025, 16047, 16053, 16063]}, {"Fips"=16065, "FipsAdj"=[16019, 16043, 16051, 16065]}, {"Fips"=16067, "FipsAdj"=[16013, 16031, 16053, 16063]}, {"Fips"=16069, "FipsAdj"=[16035, 16049, 16057, 16061, 16069, 41063, 53003]}, {"Fips"=16071, "FipsAdj"=[16005, 16031, 16041, 16071, 16077, 49003]}, {"Fips"=16073, "FipsAdj"=[16001, 16027, 16039, 16073, 16083, 32007, 32013]}, {"Fips"=16075, "FipsAdj"=[16027, 16045, 16075, 16087]}, {"Fips"=16077, "FipsAdj"=[16005, 16011, 16013, 16031, 16071]}, {"Fips"=16079, "FipsAdj"=[16009, 16017, 16035, 16055, 16057, 16079, 30061]}, {"Fips"=16081, "FipsAdj"=[16019, 16043, 16065, 16081]}, {"Fips"=16083, "FipsAdj"=[16031, 16039, 16047, 16053, 16073, 16083]}, {"Fips"=16085, "FipsAdj"=[16003, 16015, 16037, 16045, 16049, 16059]}, {"Fips"=16087, "FipsAdj"=[16003, 16045, 16075, 16087, 41001]}, {"Fips"=17001, "FipsAdj"=[17001, 17009, 17067, 17149, 17169, 29111]}, {"Fips"=17003, "FipsAdj"=[17003, 17153, 17181, 21007, 29031, 29133]}, {"Fips"=17005, "FipsAdj"=[17005, 17027, 17051, 17119]}, {"Fips"=17007, "FipsAdj"=[17007, 17037, 17111, 17141, 17201, 55105]}, {"Fips"=17009, "FipsAdj"=[17001, 17009, 17017, 17137, 17149]}, {"Fips"=17011, "FipsAdj"=[17011, 17073, 17099, 17103, 17123, 17155, 17175]}, {"Fips"=17013, "FipsAdj"=[17013, 17061, 17083, 17149, 29113, 29163]}, {"Fips"=17015, "FipsAdj"=[17015, 17085, 17141, 17177, 17195, 19045]}, {"Fips"=17017, "FipsAdj"=[17009, 17017, 17125, 17129, 17137, 17167]}, {"Fips"=17019, "FipsAdj"=[17019, 17041, 17045, 17053, 17113, 17147]}, {"Fips"=17021, "FipsAdj"=[17021, 17115, 17135, 17167]}, {"Fips"=17023, "FipsAdj"=[17023, 17029, 17033, 17035, 17045, 17079, 18153]}, {"Fips"=17025, "FipsAdj"=[17025, 17049, 17051, 17079, 17121, 17159]}, {"Fips"=17027, "FipsAdj"=[17005, 17027, 17051, 17119, 17121, 17163]}, {"Fips"=17029, "FipsAdj"=[17023, 17029, 17035, 17041, 17045, 17139]}, {"Fips"=17031, "FipsAdj"=[17031, 17043, 17089, 17097, 17111, 17197, 18089, 18127]}, {"Fips"=17033, "FipsAdj"=[17023, 17033, 17079, 17101, 17159, 18083]}, {"Fips"=17035, "FipsAdj"=[17023, 17029, 17035, 17049, 17079]}, {"Fips"=17037, "FipsAdj"=[17007, 17037, 17089, 17093, 17099, 17103, 17111, 17141]}, {"Fips"=17039, "FipsAdj"=[17039, 17107, 17113, 17115]}, {"Fips"=17041, "FipsAdj"=[17019, 17029, 17041, 17045, 17139, 17147]}, {"Fips"=17043, "FipsAdj"=[17031, 17043, 17089, 17093]}, {"Fips"=17045, "FipsAdj"=[17019, 17023, 17029, 17041, 17045, 17183, 18165]}, {"Fips"=17047, "FipsAdj"=[17047, 17159, 17185, 17191]}, {"Fips"=17049, "FipsAdj"=[17025, 17035, 17049, 17051, 17079]}, {"Fips"=17051, "FipsAdj"=[17005, 17025, 17027, 17049, 17051, 17121, 17135]}, {"Fips"=17053, "FipsAdj"=[17019, 17053, 17075, 17091, 17105, 17113]}, {"Fips"=17055, "FipsAdj"=[17055, 17065, 17077, 17081, 17145, 17165]}, {"Fips"=17057, "FipsAdj"=[17057, 17095, 17109, 17125, 17143, 17169, 17179]}, {"Fips"=17059, "FipsAdj"=[17059, 17065, 17069, 17165, 17193, 18129]}, {"Fips"=17061, "FipsAdj"=[17013, 17061, 17083, 17117, 17137, 17149]}, {"Fips"=17063, "FipsAdj"=[17063, 17091, 17093, 17099, 17105]}, {"Fips"=17065, "FipsAdj"=[17055, 17059, 17065, 17081, 17165, 17191]}, {"Fips"=17067, "FipsAdj"=[17001, 17067, 17071, 17109, 17169, 19111, 29045]}, {"Fips"=17069, "FipsAdj"=[17059, 17069, 17151, 17165, 21055, 21139]}, {"Fips"=17071, "FipsAdj"=[17067, 17071, 17109, 17131, 17187, 19057]}, {"Fips"=17073, "FipsAdj"=[17011, 17073, 17095, 17131, 17161, 17175]}, {"Fips"=17075, "FipsAdj"=[17053, 17075, 17091, 17183, 18007]}, {"Fips"=17077, "FipsAdj"=[17055, 17077, 17145, 17157, 17181, 17199]}, {"Fips"=17079, "FipsAdj"=[17023, 17025, 17033, 17035, 17049, 17079]}, {"Fips"=17081, "FipsAdj"=[17055, 17065, 17081, 17121, 17145, 17189]}, {"Fips"=17083, "FipsAdj"=[17013, 17061, 17083, 17117, 17119]}, {"Fips"=17085, "FipsAdj"=[17015, 17085, 17177, 19061, 19097, 55043]}, {"Fips"=17087, "FipsAdj"=[17087, 17127, 17151, 17153, 17165, 17181]}, {"Fips"=17089, "FipsAdj"=[17031, 17037, 17043, 17089, 17093]}, {"Fips"=17091, "FipsAdj"=[17053, 17063, 17075, 17091, 17105, 17197, 18089]}, {"Fips"=17093, "FipsAdj"=[17037, 17043, 17063, 17089, 17093, 17099]}, {"Fips"=17095, "FipsAdj"=[17057, 17073, 17095, 17131, 17143, 17175]}, {"Fips"=17097, "FipsAdj"=[17031, 17097, 17111, 26005, 26021, 26159]}, {"Fips"=17099, "FipsAdj"=[17011, 17037, 17063, 17093, 17099, 17103, 17105, 17123, 17155]}, {"Fips"=17101, "FipsAdj"=[17033, 17101, 17159, 17185]}, {"Fips"=17103, "FipsAdj"=[17011, 17037, 17099, 17103, 17141]}, {"Fips"=17105, "FipsAdj"=[17053, 17063, 17091, 17099, 17105, 17113]}, {"Fips"=17107, "FipsAdj"=[17039, 17107, 17113, 17115, 17125, 17129, 17167]}, {"Fips"=17109, "FipsAdj"=[17057, 17067, 17071, 17109, 17169]}, {"Fips"=17111, "FipsAdj"=[17007, 17031, 17037, 17089, 17097, 17111, 55059]}, {"Fips"=17113, "FipsAdj"=[17019, 17039, 17053, 17105, 17107, 17113, 17147, 17179]}, {"Fips"=17115, "FipsAdj"=[17021, 17039, 17107, 17115, 17139, 17147, 17167]}, {"Fips"=17117, "FipsAdj"=[17061, 17083, 17117, 17119, 17135, 17137]}, {"Fips"=17119, "FipsAdj"=[17005, 17027, 17083, 17117, 17119, 17135, 17163, 29183, 29189]}, {"Fips"=17121, "FipsAdj"=[17025, 17027, 17051, 17081, 17121, 17189]}, {"Fips"=17123, "FipsAdj"=[17011, 17099, 17123, 17143, 17155, 17175]}, {"Fips"=17125, "FipsAdj"=[17017, 17057, 17107, 17125, 17129, 17169]}, {"Fips"=17127, "FipsAdj"=[17087, 17127, 17151, 17153, 21139]}, {"Fips"=17129, "FipsAdj"=[17017, 17107, 17125, 17129]}, {"Fips"=17131, "FipsAdj"=[17071, 17073, 17095, 17131, 17161, 17187, 19057]}, {"Fips"=17133, "FipsAdj"=[17133, 17157, 17163, 29099, 29186]}, {"Fips"=17135, "FipsAdj"=[17005, 17021, 17051, 17117, 17119, 17135, 17167]}, {"Fips"=17137, "FipsAdj"=[17009, 17017, 17061, 17117, 17137, 17149, 17167]}, {"Fips"=17139, "FipsAdj"=[17029, 17041, 17115, 17139, 17147]}, {"Fips"=17141, "FipsAdj"=[17007, 17015, 17037, 17103, 17141, 17177, 17195]}, {"Fips"=17143, "FipsAdj"=[17057, 17095, 17123, 17143, 17175, 17179]}, {"Fips"=17145, "FipsAdj"=[17055, 17077, 17081, 17145, 17157]}, {"Fips"=17147, "FipsAdj"=[17019, 17039, 17041, 17113, 17115, 17139]}, {"Fips"=17149, "FipsAdj"=[17001, 17009, 17013, 17061, 17137, 17149, 17171, 29127, 29163]}, {"Fips"=17151, "FipsAdj"=[17069, 17087, 17127, 17151, 17165, 17199]}, {"Fips"=17153, "FipsAdj"=[17003, 17087, 17127, 17153, 17181, 21007]}, {"Fips"=17155, "FipsAdj"=[17011, 17099, 17123]}, {"Fips"=17157, "FipsAdj"=[17077, 17133, 17145, 17157, 17163, 17189, 29157]}, {"Fips"=17159, "FipsAdj"=[17025, 17033, 17047, 17079, 17101, 17159, 17185]}, {"Fips"=17161, "FipsAdj"=[17073, 17131, 17161, 17195, 19045, 19115, 19139]}, {"Fips"=17163, "FipsAdj"=[17027, 17119, 17133, 17157, 17163, 17189, 29189]}, {"Fips"=17165, "FipsAdj"=[17055, 17059, 17065, 17069, 17087, 17151, 17165]}, {"Fips"=17167, "FipsAdj"=[17017, 17021, 17107, 17115, 17117, 17129, 17135, 17137]}, {"Fips"=17169, "FipsAdj"=[17001, 17009, 17017, 17057, 17067, 17109, 17125]}, {"Fips"=17171, "FipsAdj"=[17061, 17137, 17149]}, {"Fips"=17173, "FipsAdj"=[17021, 17029, 17035, 17049, 17051, 17115, 17135, 17139]}, {"Fips"=17175, "FipsAdj"=[17011, 17073, 17095, 17123, 17143]}, {"Fips"=17177, "FipsAdj"=[17015, 17085, 17141, 17177, 17201, 55045]}, {"Fips"=17179, "FipsAdj"=[17057, 17107, 17113, 17125, 17143, 17179]}, {"Fips"=17181, "FipsAdj"=[17003, 17077, 17087, 17153, 17181, 17199, 29031]}, {"Fips"=17183, "FipsAdj"=[17019, 17041, 17045, 17053, 17075, 17183, 18007, 18165]}, {"Fips"=17185, "FipsAdj"=[17047, 17101, 17159, 17185, 17193, 18051]}, {"Fips"=17187, "FipsAdj"=[17057, 17071, 17095, 17109, 17131]}, {"Fips"=17189, "FipsAdj"=[17027, 17081, 17121, 17145, 17157, 17163]}, {"Fips"=17191, "FipsAdj"=[17025, 17047, 17065, 17081, 17121, 17159, 17191]}, {"Fips"=17193, "FipsAdj"=[17047, 17059, 17065, 17185, 17191, 17193, 18051]}, {"Fips"=17195, "FipsAdj"=[17011, 17015, 17073, 17103, 17141, 17161, 17195]}, {"Fips"=17197, "FipsAdj"=[17031, 17043, 17063, 17091, 17093, 17197]}, {"Fips"=17199, "FipsAdj"=[17055, 17077, 17087, 17151, 17165, 17181]}, {"Fips"=17201, "FipsAdj"=[17007, 17037, 17141, 17177, 17201, 55045]}, {"Fips"=17203, "FipsAdj"=[17099, 17105, 17113, 17123, 17143, 17179]}, {"Fips"=18001, "FipsAdj"=[18001, 18003, 18075, 18179, 39107]}, {"Fips"=18003, "FipsAdj"=[18001, 18003, 18033, 18069, 18113, 18179, 18183, 39039, 39125]}, {"Fips"=18005, "FipsAdj"=[18005, 18013, 18031, 18071, 18079, 18081]}, {"Fips"=18007, "FipsAdj"=[17075, 17183, 18007, 18073, 18111, 18157, 18171]}, {"Fips"=18009, "FipsAdj"=[18009, 18035, 18053, 18075]}, {"Fips"=18011, "FipsAdj"=[18011, 18023, 18057, 18063, 18097]}, {"Fips"=18013, "FipsAdj"=[18005, 18013, 18071, 18081, 18105]}, {"Fips"=18015, "FipsAdj"=[18015, 18017, 18023, 18067, 18157]}, {"Fips"=18017, "FipsAdj"=[18015, 18017, 18049, 18067, 18103, 18131]}, {"Fips"=18019, "FipsAdj"=[18019, 18043, 18077, 18143, 18175, 21111, 21185]}, {"Fips"=18021, "FipsAdj"=[18021, 18055, 18119, 18121, 18133, 18153]}, {"Fips"=18023, "FipsAdj"=[18011, 18015, 18023, 18057, 18067, 18107, 18157]}, {"Fips"=18025, "FipsAdj"=[18025, 18037, 18061, 18117, 18123, 18175]}, {"Fips"=18027, "FipsAdj"=[18027, 18037, 18055, 18083, 18101]}, {"Fips"=18029, "FipsAdj"=[18029, 18047, 18115, 18137, 21015, 39017]}, {"Fips"=18031, "FipsAdj"=[18005, 18031, 18047, 18079, 18137, 18139]}, {"Fips"=18033, "FipsAdj"=[18003, 18033, 18087, 18113, 18151, 39039]}, {"Fips"=18035, "FipsAdj"=[18009, 18035, 18053, 18065, 18075, 18095]}, {"Fips"=18037, "FipsAdj"=[18025, 18027, 18037, 18101, 18117, 18123, 18125, 18147]}, {"Fips"=18039, "FipsAdj"=[18039, 18085, 18087, 18099, 18113, 18141, 26027]}, {"Fips"=18041, "FipsAdj"=[18041, 18047, 18065, 18139, 18161]}, {"Fips"=18043, "FipsAdj"=[18019, 18043, 18061, 18175]}, {"Fips"=18045, "FipsAdj"=[18045, 18107, 18121, 18157, 18165]}, {"Fips"=18047, "FipsAdj"=[18029, 18031, 18041, 18047, 18137, 18139, 18161, 39017]}, {"Fips"=18049, "FipsAdj"=[18017, 18049, 18085, 18099, 18103, 18131, 18149]}, {"Fips"=18051, "FipsAdj"=[17185, 17193, 18051, 18083, 18125, 18129, 18163]}, {"Fips"=18053, "FipsAdj"=[18009, 18035, 18053, 18067, 18069, 18095, 18103, 18159, 18169]}, {"Fips"=18055, "FipsAdj"=[18021, 18027, 18055, 18083, 18093, 18101, 18105, 18119]}, {"Fips"=18057, "FipsAdj"=[18011, 18023, 18057, 18059, 18095, 18097]}, {"Fips"=18059, "FipsAdj"=[18057, 18059, 18065, 18095, 18097, 18139]}, {"Fips"=18061, "FipsAdj"=[18025, 18043, 18061, 18175, 21093, 21111]}, {"Fips"=18063, "FipsAdj"=[18011, 18063, 18097, 18107, 18109]}, {"Fips"=18065, "FipsAdj"=[18035, 18041, 18059, 18065, 18095, 18135, 18139]}, {"Fips"=18067, "FipsAdj"=[18015, 18017, 18023, 18053, 18067, 18103]}, {"Fips"=18069, "FipsAdj"=[18003, 18053, 18069, 18169, 18179]}, {"Fips"=18071, "FipsAdj"=[18005, 18013, 18071, 18079, 18093, 18105, 18143]}, {"Fips"=18073, "FipsAdj"=[18007, 18073, 18089, 18091, 18111, 18127, 18131, 18149]}, {"Fips"=18075, "FipsAdj"=[18001, 18009, 18035, 18075, 18135, 18179, 39037]}, {"Fips"=18077, "FipsAdj"=[18019, 18077, 18079, 18137, 18143, 18155, 21041]}, {"Fips"=18079, "FipsAdj"=[18005, 18031, 18071, 18077, 18079, 18137]}, {"Fips"=18081, "FipsAdj"=[18005, 18013, 18081, 18097, 18109]}, {"Fips"=18083, "FipsAdj"=[17033, 17101, 17185, 18027, 18051, 18055, 18083, 18125]}, {"Fips"=18085, "FipsAdj"=[18039, 18049, 18085, 18099, 18113, 18169]}, {"Fips"=18087, "FipsAdj"=[18033, 18039, 18087, 18113, 18151, 26023]}, {"Fips"=18089, "FipsAdj"=[17031, 17091, 17197, 18073, 18089, 18111]}, {"Fips"=18091, "FipsAdj"=[18073, 18091, 18127, 18141, 18149]}, {"Fips"=18093, "FipsAdj"=[18055, 18071, 18093, 18101, 18105, 18117]}, {"Fips"=18095, "FipsAdj"=[18035, 18053, 18057, 18059, 18065, 18095]}, {"Fips"=18097, "FipsAdj"=[18011, 18057, 18059, 18063, 18081, 18097, 18109]}, {"Fips"=18099, "FipsAdj"=[18039, 18049, 18085, 18099, 18131, 18141]}, {"Fips"=18101, "FipsAdj"=[18027, 18037, 18055, 18093, 18101]}, {"Fips"=18103, "FipsAdj"=[18017, 18049, 18053, 18067, 18103]}, {"Fips"=18105, "FipsAdj"=[18013, 18055, 18071, 18093, 18105, 18109]}, {"Fips"=18107, "FipsAdj"=[18011, 18023, 18045, 18063, 18107, 18121, 18133]}, {"Fips"=18109, "FipsAdj"=[18013, 18063, 18081, 18097, 18105, 18109, 18119]}, {"Fips"=18111, "FipsAdj"=[17075, 17091, 18007, 18073, 18089]}, {"Fips"=18113, "FipsAdj"=[18003, 18033, 18039, 18085, 18087, 18113, 18151]}, {"Fips"=18115, "FipsAdj"=[18029, 18115, 18137, 18155]}, {"Fips"=18117, "FipsAdj"=[18025, 18037, 18093, 18101, 18117]}, {"Fips"=18119, "FipsAdj"=[18021, 18055, 18105, 18109, 18119]}, {"Fips"=18121, "FipsAdj"=[18021, 18045, 18107, 18121, 18133, 18165]}, {"Fips"=18123, "FipsAdj"=[18025, 18037, 18123, 18147, 21027, 21091]}, {"Fips"=18125, "FipsAdj"=[18027, 18037, 18051, 18083, 18125]}, {"Fips"=18127, "FipsAdj"=[17031, 18073, 18089, 18091, 18127, 18149]}, {"Fips"=18129, "FipsAdj"=[17059, 17193, 18051, 18129, 18163, 21101]}, {"Fips"=18131, "FipsAdj"=[18017, 18049, 18073, 18099, 18131, 18149]}, {"Fips"=18133, "FipsAdj"=[18021, 18063, 18107, 18109, 18119, 18121]}, {"Fips"=18135, "FipsAdj"=[18035, 18065, 18075, 18135, 18177]}, {"Fips"=18137, "FipsAdj"=[18029, 18031, 18047, 18077, 18079, 18115, 18137]}, {"Fips"=18139, "FipsAdj"=[18031, 18041, 18047, 18059, 18065, 18139]}, {"Fips"=18141, "FipsAdj"=[18039, 18091, 18099, 18141, 18149, 26021]}, {"Fips"=18143, "FipsAdj"=[18019, 18071, 18077, 18079, 18143]}, {"Fips"=18145, "FipsAdj"=[18005, 18031, 18059, 18081, 18097, 18139]}, {"Fips"=18147, "FipsAdj"=[18037, 18123, 18147, 18173, 21059]}, {"Fips"=18149, "FipsAdj"=[18049, 18073, 18091, 18099, 18127, 18131, 18141]}, {"Fips"=18151, "FipsAdj"=[18033, 18087, 18113, 18151, 26023, 26059]}, {"Fips"=18153, "FipsAdj"=[17023, 17033, 18021, 18055, 18083, 18153]}, {"Fips"=18155, "FipsAdj"=[18077, 18115, 18137, 18155, 21015, 21041]}, {"Fips"=18157, "FipsAdj"=[18007, 18015, 18023, 18045, 18107, 18157, 18171]}, {"Fips"=18159, "FipsAdj"=[18023, 18053, 18057, 18067, 18095]}, {"Fips"=18161, "FipsAdj"=[18041, 18047, 18161, 18177, 39017]}, {"Fips"=18163, "FipsAdj"=[18051, 18129, 18163, 18173]}, {"Fips"=18165, "FipsAdj"=[17045, 17183, 18045, 18121, 18165, 18167]}, {"Fips"=18167, "FipsAdj"=[17023, 17045, 18021, 18121, 18153, 18165]}, {"Fips"=18169, "FipsAdj"=[18049, 18053, 18069, 18085, 18103, 18169]}, {"Fips"=18171, "FipsAdj"=[17183, 18007, 18045, 18157, 18165]}, {"Fips"=18173, "FipsAdj"=[18037, 18051, 18125, 18147, 18163, 18173, 21059]}, {"Fips"=18175, "FipsAdj"=[18019, 18025, 18043, 18061, 18071, 18093, 18117, 18143]}, {"Fips"=18177, "FipsAdj"=[18041, 18065, 18135, 18161, 18177, 39037]}, {"Fips"=18179, "FipsAdj"=[18001, 18003, 18009, 18053, 18069, 18075]}, {"Fips"=18181, "FipsAdj"=[18007, 18015, 18017, 18073, 18131, 18157]}, {"Fips"=18183, "FipsAdj"=[18003, 18069, 18085, 18113, 18169]}, {"Fips"=19001, "FipsAdj"=[19001, 19003, 19009, 19029, 19049, 19077, 19121]}, {"Fips"=19003, "FipsAdj"=[19001, 19003, 19029, 19137, 19145, 19159, 19173]}, {"Fips"=19005, "FipsAdj"=[19005, 19043, 19065, 19191, 27055, 55023]}, {"Fips"=19007, "FipsAdj"=[19007, 19051, 19117, 19135, 19179, 19185, 29171]}, {"Fips"=19009, "FipsAdj"=[19001, 19009, 19027, 19029, 19047, 19077]}, {"Fips"=19011, "FipsAdj"=[19011, 19013, 19019, 19095, 19103, 19113, 19157]}, {"Fips"=19013, "FipsAdj"=[19011, 19013, 19017, 19019, 19023, 19065, 19075]}, {"Fips"=19015, "FipsAdj"=[19015, 19049, 19073, 19079, 19153, 19169]}, {"Fips"=19017, "FipsAdj"=[19013, 19017, 19019, 19023, 19037, 19065]}, {"Fips"=19019, "FipsAdj"=[19011, 19013, 19017, 19019, 19043, 19055, 19065]}, {"Fips"=19021, "FipsAdj"=[19021, 19025, 19035, 19041, 19093, 19141, 19147, 19151]}, {"Fips"=19023, "FipsAdj"=[19013, 19017, 19023, 19033, 19037, 19067, 19069, 19075]}, {"Fips"=19025, "FipsAdj"=[19021, 19025, 19027, 19073, 19151, 19161]}, {"Fips"=19027, "FipsAdj"=[19009, 19025, 19027, 19047, 19073, 19077, 19161]}, {"Fips"=19029, "FipsAdj"=[19001, 19003, 19009, 19029, 19077, 19137, 19155]}, {"Fips"=19031, "FipsAdj"=[19031, 19045, 19103, 19105, 19113, 19139]}, {"Fips"=19033, "FipsAdj"=[19023, 19033, 19067, 19069, 19081, 19131, 19189, 19195]}, {"Fips"=19035, "FipsAdj"=[19021, 19035, 19041, 19093, 19141, 19149, 19161, 19167]}, {"Fips"=19037, "FipsAdj"=[19017, 19023, 19037, 19065, 19067, 19089, 19131]}, {"Fips"=19039, "FipsAdj"=[19039, 19053, 19117, 19121, 19159, 19175, 19181]}, {"Fips"=19041, "FipsAdj"=[19021, 19035, 19041, 19059, 19063, 19141, 19143, 19147]}, {"Fips"=19043, "FipsAdj"=[19005, 19019, 19043, 19055, 19061, 19065, 19191, 55023]}, {"Fips"=19045, "FipsAdj"=[17015, 17161, 17195, 19031, 19045, 19097, 19105]}, {"Fips"=19047, "FipsAdj"=[19009, 19027, 19047, 19085, 19093, 19133, 19161, 19165]}, {"Fips"=19049, "FipsAdj"=[19001, 19015, 19049, 19073, 19077, 19121, 19153]}, {"Fips"=19051, "FipsAdj"=[19007, 19051, 19101, 19135, 19177, 19179, 29197]}, {"Fips"=19053, "FipsAdj"=[19039, 19053, 19117, 19159, 19175, 19185, 29081]}, {"Fips"=19055, "FipsAdj"=[19019, 19043, 19055, 19061, 19065, 19105]}, {"Fips"=19057, "FipsAdj"=[17071, 17131, 19057, 19087, 19111]}, {"Fips"=19059, "FipsAdj"=[19041, 19059, 19063, 19141, 19143, 19147]}, {"Fips"=19061, "FipsAdj"=[17085, 19043, 19055, 19061, 19097, 19105]}, {"Fips"=19063, "FipsAdj"=[19041, 19059, 19063, 19109, 19147, 27063]}, {"Fips"=19065, "FipsAdj"=[19005, 19013, 19017, 19019, 19037, 19043, 19055, 19065]}, {"Fips"=19067, "FipsAdj"=[19017, 19023, 19033, 19037, 19067, 19069, 19089]}, {"Fips"=19069, "FipsAdj"=[19023, 19033, 19067, 19069, 19075, 19079, 19081, 19083]}, {"Fips"=19071, "FipsAdj"=[19071, 19129, 19137, 19145, 29005, 31025]}, {"Fips"=19073, "FipsAdj"=[19015, 19025, 19027, 19049, 19073, 19077]}, {"Fips"=19075, "FipsAdj"=[19013, 19023, 19069, 19075, 19083, 19127]}, {"Fips"=19077, "FipsAdj"=[19001, 19009, 19027, 19029, 19049, 19073, 19077]}, {"Fips"=19079, "FipsAdj"=[19015, 19069, 19079, 19083, 19169, 19187]}, {"Fips"=19081, "FipsAdj"=[19033, 19069, 19081, 19091, 19109, 19189, 19195]}, {"Fips"=19083, "FipsAdj"=[19023, 19069, 19075, 19079, 19083, 19127, 19169]}, {"Fips"=19085, "FipsAdj"=[19047, 19085, 19133, 19155, 19165, 31021]}, {"Fips"=19087, "FipsAdj"=[19057, 19087, 19101, 19111, 19115, 19177]}, {"Fips"=19089, "FipsAdj"=[19037, 19067, 19089, 19131, 19191, 27045]}, {"Fips"=19091, "FipsAdj"=[19081, 19091, 19109, 19147, 19151, 19187]}, {"Fips"=19093, "FipsAdj"=[19021, 19035, 19047, 19093, 19133, 19161]}, {"Fips"=19095, "FipsAdj"=[19011, 19095, 19103, 19107, 19113, 19157, 19171]}, {"Fips"=19097, "FipsAdj"=[17015, 17085, 19045, 19061, 19097]}, {"Fips"=19099, "FipsAdj"=[19099, 19123, 19125, 19127, 19153, 19157, 19169]}, {"Fips"=19101, "FipsAdj"=[19051, 19087, 19101, 19107, 19177, 19179]}, {"Fips"=19103, "FipsAdj"=[19011, 19031, 19095, 19103, 19113, 19115, 19139]}, {"Fips"=19105, "FipsAdj"=[19031, 19045, 19055, 19061, 19097, 19105]}, {"Fips"=19107, "FipsAdj"=[19095, 19101, 19107, 19123, 19157, 19179]}, {"Fips"=19109, "FipsAdj"=[19063, 19081, 19091, 19109, 19147, 19151, 19189, 19197, 27043]}, {"Fips"=19111, "FipsAdj"=[17067, 17071, 19057, 19087, 19111, 19177]}, {"Fips"=19113, "FipsAdj"=[19011, 19019, 19031, 19055, 19095, 19103, 19105]}, {"Fips"=19115, "FipsAdj"=[17131, 17161, 19057, 19087, 19103, 19115, 19139]}, {"Fips"=19117, "FipsAdj"=[19007, 19039, 19053, 19117, 19125, 19135, 19181]}, {"Fips"=19119, "FipsAdj"=[19119, 19141, 19143, 19167, 27105, 27133, 46083]}, {"Fips"=19121, "FipsAdj"=[19001, 19039, 19049, 19077, 19121, 19153, 19175]}, {"Fips"=19123, "FipsAdj"=[19099, 19107, 19123, 19125, 19135, 19157]}, {"Fips"=19125, "FipsAdj"=[19099, 19117, 19123, 19125, 19135, 19153]}, {"Fips"=19127, "FipsAdj"=[19075, 19083, 19099, 19127, 19157, 19169]}, {"Fips"=19129, "FipsAdj"=[19071, 19129, 19137, 19145, 19155, 31025]}, {"Fips"=19131, "FipsAdj"=[19033, 19037, 19067, 19089, 19131, 19195]}, {"Fips"=19133, "FipsAdj"=[19047, 19085, 19093, 19133, 19193, 31021]}, {"Fips"=19135, "FipsAdj"=[19007, 19051, 19117, 19123, 19125, 19135, 19179]}, {"Fips"=19137, "FipsAdj"=[19003, 19029, 19071, 19129, 19137, 19145, 19155]}, {"Fips"=19139, "FipsAdj"=[17161, 19031, 19103, 19115, 19139]}, {"Fips"=19141, "FipsAdj"=[19021, 19035, 19041, 19059, 19119, 19141, 19143, 19149]}, {"Fips"=19143, "FipsAdj"=[19041, 19059, 19119, 19141, 19143, 19167, 27063]}, {"Fips"=19145, "FipsAdj"=[19003, 19071, 19129, 19137, 19145, 19173, 29005]}, {"Fips"=19147, "FipsAdj"=[19021, 19041, 19059, 19063, 19091, 19109, 19147]}, {"Fips"=19149, "FipsAdj"=[19035, 19141, 19149, 19167, 19193]}, {"Fips"=19151, "FipsAdj"=[19021, 19025, 19041, 19091, 19109, 19147, 19151, 19161]}, {"Fips"=19153, "FipsAdj"=[19015, 19049, 19099, 19121, 19125, 19153, 19169]}, {"Fips"=19155, "FipsAdj"=[19029, 19085, 19129, 19137, 19155, 19165, 31055, 31153]}, {"Fips"=19157, "FipsAdj"=[19011, 19095, 19099, 19107, 19123, 19127, 19157]}, {"Fips"=19159, "FipsAdj"=[19003, 19039, 19053, 19159, 19173, 19175, 29081]}, {"Fips"=19161, "FipsAdj"=[19021, 19025, 19027, 19035, 19047, 19093, 19151]}, {"Fips"=19163, "FipsAdj"=[17161, 19031, 19045, 19139]}, {"Fips"=19165, "FipsAdj"=[19009, 19027, 19029, 19047, 19085, 19155]}, {"Fips"=19167, "FipsAdj"=[19035, 19119, 19141, 19143, 19149, 19167, 46083]}, {"Fips"=19169, "FipsAdj"=[19015, 19079, 19083, 19099, 19127, 19153]}, {"Fips"=19171, "FipsAdj"=[19011, 19013, 19075, 19095, 19099, 19127, 19157]}, {"Fips"=19173, "FipsAdj"=[19003, 19137, 19145, 19159, 19173, 19175, 29147]}, {"Fips"=19175, "FipsAdj"=[19001, 19003, 19039, 19053, 19121, 19159, 19173]}, {"Fips"=19177, "FipsAdj"=[19051, 19087, 19101, 19111, 19177, 19179, 29045]}, {"Fips"=19179, "FipsAdj"=[19007, 19051, 19101, 19107, 19123, 19135, 19177]}, {"Fips"=19181, "FipsAdj"=[19039, 19049, 19117, 19121, 19125, 19153]}, {"Fips"=19183, "FipsAdj"=[19087, 19095, 19101, 19103, 19107, 19115]}, {"Fips"=19185, "FipsAdj"=[19007, 19039, 19053, 19117, 19135, 19185, 29129]}, {"Fips"=19187, "FipsAdj"=[19015, 19025, 19073, 19079, 19091, 19151, 19187]}, {"Fips"=19189, "FipsAdj"=[19033, 19081, 19109, 19189, 19195, 27043]}, {"Fips"=19191, "FipsAdj"=[19005, 19037, 19043, 19065, 19089, 19191, 27045]}, {"Fips"=19193, "FipsAdj"=[19035, 19047, 19093, 19133, 19149, 19193, 31043, 31173]}, {"Fips"=19195, "FipsAdj"=[19033, 19081, 19131, 19189, 19195, 27047]}, {"Fips"=19197, "FipsAdj"=[19033, 19069, 19079, 19081, 19083, 19091, 19109, 19187]}, {"Fips"=20001, "FipsAdj"=[20001, 20003, 20011, 20031, 20107, 20133, 20205]}, {"Fips"=20003, "FipsAdj"=[20001, 20003, 20011, 20031, 20059, 20107, 20121]}, {"Fips"=20005, "FipsAdj"=[20005, 20013, 20043, 20085, 20087, 20103, 29021]}, {"Fips"=20007, "FipsAdj"=[20007, 20033, 20077, 20095, 20097, 20151, 40003]}, {"Fips"=20009, "FipsAdj"=[20009, 20053, 20145, 20159, 20165, 20167]}, {"Fips"=20011, "FipsAdj"=[20001, 20003, 20011, 20037, 20107, 20133]}, {"Fips"=20013, "FipsAdj"=[20005, 20013, 20043, 20085, 20131]}, {"Fips"=20015, "FipsAdj"=[20015, 20017, 20035, 20049, 20073, 20079, 20115, 20173]}, {"Fips"=20017, "FipsAdj"=[20015, 20017, 20073, 20111, 20115]}, {"Fips"=20019, "FipsAdj"=[20019, 20035, 20049, 20125, 40113]}, {"Fips"=20021, "FipsAdj"=[20021, 20037, 20099, 29097, 29145, 40035]}, {"Fips"=20023, "FipsAdj"=[8063, 8125, 20023, 20153, 20181]}, {"Fips"=20025, "FipsAdj"=[20025, 20033, 20057, 20097, 20119, 40007]}, {"Fips"=20027, "FipsAdj"=[20027, 20029, 20041, 20061, 20143, 20161]}, {"Fips"=20029, "FipsAdj"=[20027, 20029, 20089, 20123, 20143, 20157]}, {"Fips"=20031, "FipsAdj"=[20001, 20003, 20031, 20059, 20073, 20111, 20139]}, {"Fips"=20033, "FipsAdj"=[20007, 20025, 20033, 20097, 40059]}, {"Fips"=20035, "FipsAdj"=[20015, 20019, 20035, 20049, 20173, 20191, 40071]}, {"Fips"=20037, "FipsAdj"=[20011, 20021, 20037, 20099, 20133, 29011, 29097]}, {"Fips"=20039, "FipsAdj"=[20039, 20137, 20153, 20179, 20193, 31065]}, {"Fips"=20041, "FipsAdj"=[20027, 20041, 20061, 20113, 20115, 20127, 20143]}, {"Fips"=20043, "FipsAdj"=[20005, 20013, 20043, 29003, 29021, 29087]}, {"Fips"=20045, "FipsAdj"=[20045, 20059, 20087, 20091, 20103, 20121, 20139]}, {"Fips"=20047, "FipsAdj"=[20047, 20057, 20083, 20097, 20145, 20151]}, {"Fips"=20049, "FipsAdj"=[20015, 20019, 20035, 20049, 20073, 20125]}, {"Fips"=20051, "FipsAdj"=[20051, 20135, 20141, 20163, 20165, 20167]}, {"Fips"=20053, "FipsAdj"=[20009, 20053, 20105, 20113, 20159, 20167]}, {"Fips"=20055, "FipsAdj"=[20055, 20067, 20069, 20081, 20083, 20093, 20101, 20135]}, {"Fips"=20057, "FipsAdj"=[20025, 20047, 20057, 20069, 20083, 20097]}, {"Fips"=20059, "FipsAdj"=[20003, 20031, 20045, 20059, 20091, 20107, 20121]}, {"Fips"=20061, "FipsAdj"=[20027, 20041, 20061, 20127, 20161]}, {"Fips"=20063, "FipsAdj"=[20063, 20065, 20101, 20109, 20135, 20171, 20179, 20193]}, {"Fips"=20065, "FipsAdj"=[20063, 20065, 20137, 20147, 20163, 20179]}, {"Fips"=20067, "FipsAdj"=[20055, 20067, 20075, 20081, 20093, 20187]}, {"Fips"=20069, "FipsAdj"=[20055, 20057, 20069, 20081, 20083]}, {"Fips"=20071, "FipsAdj"=[8017, 8061, 8099, 20071, 20075, 20199]}, {"Fips"=20073, "FipsAdj"=[20015, 20017, 20031, 20049, 20073, 20111, 20205]}, {"Fips"=20075, "FipsAdj"=[8099, 20067, 20071, 20075, 20093, 20187]}, {"Fips"=20077, "FipsAdj"=[20007, 20077, 20095, 20191, 40003]}, {"Fips"=20079, "FipsAdj"=[20015, 20079, 20113, 20115, 20155]}, {"Fips"=20081, "FipsAdj"=[20055, 20067, 20069, 20081, 20093, 20119, 20175]}, {"Fips"=20083, "FipsAdj"=[20047, 20055, 20057, 20069, 20083, 20135]}, {"Fips"=20085, "FipsAdj"=[20005, 20013, 20085, 20087, 20131, 20149]}, {"Fips"=20087, "FipsAdj"=[20005, 20045, 20085, 20087, 20103]}, {"Fips"=20089, "FipsAdj"=[20029, 20089, 20123, 20141, 20157, 20183, 31129]}, {"Fips"=20091, "FipsAdj"=[20045, 20059, 20091, 20103, 20121, 20209, 29037]}, {"Fips"=20093, "FipsAdj"=[20055, 20067, 20075, 20081, 20093, 20171, 20187]}, {"Fips"=20095, "FipsAdj"=[20007, 20077, 20095, 20151, 20155, 20173]}, {"Fips"=20097, "FipsAdj"=[20007, 20025, 20033, 20047, 20057, 20097]}, {"Fips"=20099, "FipsAdj"=[20021, 20037, 20099, 20125, 20133, 40035]}, {"Fips"=20101, "FipsAdj"=[20055, 20063, 20101, 20135]}, {"Fips"=20103, "FipsAdj"=[20005, 20045, 20087, 20091, 20103, 20209]}, {"Fips"=20105, "FipsAdj"=[20053, 20105, 20123, 20141, 20143, 20167]}, {"Fips"=20107, "FipsAdj"=[20001, 20003, 20011, 20059, 20107, 20121, 29013]}, {"Fips"=20109, "FipsAdj"=[20063, 20109, 20171, 20181, 20193, 20199]}, {"Fips"=20111, "FipsAdj"=[20017, 20031, 20073, 20111, 20127, 20139]}, {"Fips"=20113, "FipsAdj"=[20041, 20053, 20079, 20113, 20115, 20155, 20159]}, {"Fips"=20115, "FipsAdj"=[20015, 20017, 20041, 20079, 20113, 20115, 20127]}, {"Fips"=20117, "FipsAdj"=[20117, 20131, 20149, 20161, 20201, 31067]}, {"Fips"=20119, "FipsAdj"=[20025, 20057, 20069, 20081, 20119, 20175]}, {"Fips"=20121, "FipsAdj"=[20003, 20045, 20059, 20091, 20107, 20121, 29013]}, {"Fips"=20123, "FipsAdj"=[20029, 20089, 20105, 20123, 20141]}, {"Fips"=20125, "FipsAdj"=[20019, 20049, 20099, 20125, 20133, 20205, 40105]}, {"Fips"=20127, "FipsAdj"=[20017, 20041, 20061, 20111, 20115, 20127]}, {"Fips"=20129, "FipsAdj"=[8009, 20129, 20187, 20189, 40025]}, {"Fips"=20131, "FipsAdj"=[20013, 20085, 20117, 20131, 20149, 31133]}, {"Fips"=20133, "FipsAdj"=[20001, 20011, 20037, 20099, 20125, 20133, 20205]}, {"Fips"=20135, "FipsAdj"=[20051, 20055, 20063, 20083, 20101, 20135, 20145, 20165]}, {"Fips"=20137, "FipsAdj"=[20039, 20065, 20137, 20147, 20179, 31065]}, {"Fips"=20139, "FipsAdj"=[20031, 20045, 20059, 20111, 20139, 20177]}, {"Fips"=20141, "FipsAdj"=[20051, 20089, 20105, 20123, 20141, 20163, 20167]}, {"Fips"=20143, "FipsAdj"=[20027, 20029, 20041, 20105, 20123, 20143]}, {"Fips"=20145, "FipsAdj"=[20009, 20047, 20083, 20135, 20145, 20165]}, {"Fips"=20147, "FipsAdj"=[20065, 20137, 20147, 20163, 20183, 31061]}, {"Fips"=20149, "FipsAdj"=[20085, 20117, 20131, 20149, 20161, 20177]}, {"Fips"=20151, "FipsAdj"=[20007, 20047, 20095, 20097, 20151, 20155]}, {"Fips"=20153, "FipsAdj"=[20023, 20039, 20153, 20181, 20193, 31057, 31087]}, {"Fips"=20155, "FipsAdj"=[20079, 20095, 20113, 20151, 20155, 20159, 20173]}, {"Fips"=20157, "FipsAdj"=[20029, 20089, 20157, 20201, 31095, 31129]}, {"Fips"=20159, "FipsAdj"=[20009, 20053, 20113, 20155, 20159]}, {"Fips"=20161, "FipsAdj"=[20027, 20061, 20117, 20149, 20161, 20197]}, {"Fips"=20163, "FipsAdj"=[20051, 20065, 20141, 20147, 20163, 20183]}, {"Fips"=20165, "FipsAdj"=[20009, 20051, 20135, 20145, 20165]}, {"Fips"=20167, "FipsAdj"=[20009, 20051, 20053, 20105, 20141, 20165]}, {"Fips"=20169, "FipsAdj"=[20041, 20053, 20105, 20113, 20115, 20143]}, {"Fips"=20171, "FipsAdj"=[20055, 20063, 20093, 20101, 20109, 20171]}, {"Fips"=20173, "FipsAdj"=[20015, 20035, 20079, 20095, 20155, 20173]}, {"Fips"=20175, "FipsAdj"=[20081, 20119, 20175, 20189, 40007]}, {"Fips"=20177, "FipsAdj"=[20045, 20085, 20087, 20139, 20149, 20177]}, {"Fips"=20179, "FipsAdj"=[20039, 20063, 20065, 20137, 20179]}, {"Fips"=20181, "FipsAdj"=[8063, 20023, 20109, 20153, 20181, 20193]}, {"Fips"=20183, "FipsAdj"=[20089, 20141, 20147, 20163, 20183, 31061]}, {"Fips"=20185, "FipsAdj"=[20009, 20047, 20145, 20151, 20155, 20159]}, {"Fips"=20187, "FipsAdj"=[8009, 8099, 20067, 20075, 20093, 20129, 20187]}, {"Fips"=20189, "FipsAdj"=[20067, 20081, 20129, 20175, 20187, 20189]}, {"Fips"=20191, "FipsAdj"=[20015, 20035, 20077, 20095, 20173, 20191, 40053]}, {"Fips"=20193, "FipsAdj"=[20039, 20063, 20109, 20153, 20179, 20181]}, {"Fips"=20195, "FipsAdj"=[20051, 20063, 20065, 20135, 20163]}, {"Fips"=20197, "FipsAdj"=[20061, 20111, 20127, 20139, 20149, 20161, 20177]}, {"Fips"=20199, "FipsAdj"=[8017, 8063, 20071, 20109, 20181, 20199]}, {"Fips"=20201, "FipsAdj"=[20027, 20029, 20117, 20157, 20161, 20201, 31067, 31095]}, {"Fips"=20203, "FipsAdj"=[20071, 20075, 20093, 20109, 20171, 20199]}, {"Fips"=20205, "FipsAdj"=[20001, 20049, 20073, 20125, 20133, 20205]}, {"Fips"=20207, "FipsAdj"=[20001, 20003, 20031, 20073, 20133, 20205]}, {"Fips"=20209, "FipsAdj"=[20091, 20103, 20209, 29047, 29095]}, {"Fips"=21001, "FipsAdj"=[21001, 21045, 21057, 21087, 21169, 21207]}, {"Fips"=21003, "FipsAdj"=[21003, 21009, 21171, 21213, 21227, 47111]}, {"Fips"=21005, "FipsAdj"=[21005, 21073, 21167, 21179, 21211, 21215, 21229]}, {"Fips"=21007, "FipsAdj"=[17003, 17153, 21007, 21039, 21145]}, {"Fips"=21009, "FipsAdj"=[21003, 21009, 21061, 21099, 21169, 21171]}, {"Fips"=21011, "FipsAdj"=[21011, 21017, 21069, 21165, 21173, 21181]}, {"Fips"=21013, "FipsAdj"=[21013, 21051, 21095, 21121, 21131, 21235, 47025]}, {"Fips"=21015, "FipsAdj"=[18029, 18115, 18155, 21015, 21077, 21081, 21117]}, {"Fips"=21017, "FipsAdj"=[21011, 21017, 21049, 21067, 21097, 21173, 21181]}, {"Fips"=21019, "FipsAdj"=[21019, 21043, 21089, 21127, 39087]}, {"Fips"=21021, "FipsAdj"=[21021, 21045, 21079, 21137, 21155, 21167]}, {"Fips"=21023, "FipsAdj"=[21023, 21097, 21161, 21191, 21201, 39015]}, {"Fips"=21025, "FipsAdj"=[21025, 21119, 21129, 21153, 21189, 21193]}, {"Fips"=21027, "FipsAdj"=[18123, 21027, 21085, 21091, 21093, 21163]}, {"Fips"=21029, "FipsAdj"=[21029, 21093, 21111, 21179]}, {"Fips"=21031, "FipsAdj"=[21031, 21061, 21085, 21141, 21177, 21183]}, {"Fips"=21033, "FipsAdj"=[21033, 21047, 21055, 21107, 21143, 21221]}, {"Fips"=21035, "FipsAdj"=[21035, 21083, 21157, 21221, 47079]}, {"Fips"=21037, "FipsAdj"=[21037, 21117, 21191, 39025]}, {"Fips"=21039, "FipsAdj"=[21007, 21039, 21083, 21105, 21145]}, {"Fips"=21041, "FipsAdj"=[18077, 18155, 21041, 21077, 21103, 21187]}, {"Fips"=21043, "FipsAdj"=[21019, 21043, 21063, 21089, 21127, 21135]}, {"Fips"=21045, "FipsAdj"=[21001, 21021, 21045, 21137, 21155, 21199, 21207]}, {"Fips"=21047, "FipsAdj"=[21033, 21047, 21107, 21177, 21219, 21221, 47125]}, {"Fips"=21049, "FipsAdj"=[21017, 21049, 21065, 21067, 21151, 21173]}, {"Fips"=21051, "FipsAdj"=[21013, 21051, 21109, 21121, 21125, 21131, 21189]}, {"Fips"=21053, "FipsAdj"=[21053, 21057, 21207, 21231, 47027]}, {"Fips"=21055, "FipsAdj"=[17069, 21033, 21055, 21139, 21143, 21225]}, {"Fips"=21057, "FipsAdj"=[21001, 21053, 21057, 21169, 21171, 21207]}, {"Fips"=21059, "FipsAdj"=[18147, 18173, 21059, 21091, 21101, 21149]}, {"Fips"=21061, "FipsAdj"=[21009, 21031, 21061, 21085, 21099]}, {"Fips"=21063, "FipsAdj"=[21043, 21063, 21127, 21175]}, {"Fips"=21065, "FipsAdj"=[21049, 21065, 21109, 21129, 21151]}, {"Fips"=21067, "FipsAdj"=[21017, 21049, 21067, 21113, 21151, 21209]}, {"Fips"=21069, "FipsAdj"=[21011, 21069, 21135, 21161, 21181, 21201]}, {"Fips"=21071, "FipsAdj"=[21071, 21115, 21119, 21153, 21159]}, {"Fips"=21073, "FipsAdj"=[21005, 21073, 21103, 21187, 21209, 21211]}, {"Fips"=21075, "FipsAdj"=[21075, 21105, 29133, 29143, 47095]}, {"Fips"=21077, "FipsAdj"=[18155, 21015, 21041, 21077, 21081]}, {"Fips"=21079, "FipsAdj"=[21021, 21079, 21113, 21137, 21151, 21167]}, {"Fips"=21081, "FipsAdj"=[21015, 21077, 21081, 21097, 21117, 21187, 21191]}, {"Fips"=21083, "FipsAdj"=[21035, 21039, 21083, 21105, 21145, 21157, 47079]}, {"Fips"=21085, "FipsAdj"=[21027, 21031, 21061, 21085, 21093, 21099]}, {"Fips"=21087, "FipsAdj"=[21001, 21087, 21099, 21123, 21169]}, {"Fips"=21089, "FipsAdj"=[21019, 21043, 21089, 21135, 39087]}, {"Fips"=21091, "FipsAdj"=[18123, 18147, 21027, 21059, 21091]}, {"Fips"=21093, "FipsAdj"=[18061, 21027, 21029, 21085, 21093, 21099, 21111, 21123, 21163]}, {"Fips"=21095, "FipsAdj"=[21013, 21095, 21131, 21133, 21193, 51105]}, {"Fips"=21097, "FipsAdj"=[21017, 21023, 21081, 21097, 21181, 21191, 21201]}, {"Fips"=21099, "FipsAdj"=[21009, 21061, 21085, 21087, 21093, 21099, 21123]}, {"Fips"=21101, "FipsAdj"=[18129, 18163, 18173, 21059, 21101, 21149, 21225]}, {"Fips"=21103, "FipsAdj"=[21041, 21073, 21103, 21185, 21187, 21211]}, {"Fips"=21105, "FipsAdj"=[21039, 21075, 21083, 21105, 29133, 47131]}, {"Fips"=21107, "FipsAdj"=[21033, 21047, 21107, 21149, 21177]}, {"Fips"=21109, "FipsAdj"=[21051, 21065, 21109, 21125, 21129, 21151, 21189]}, {"Fips"=21111, "FipsAdj"=[18019, 18043, 18061, 21029, 21093, 21111, 21185, 21211]}, {"Fips"=21113, "FipsAdj"=[21067, 21079, 21113, 21151, 21167]}, {"Fips"=21115, "FipsAdj"=[21071, 21115, 21127, 21153, 21159]}, {"Fips"=21117, "FipsAdj"=[21015, 21037, 21081, 21117, 21191]}, {"Fips"=21119, "FipsAdj"=[21025, 21071, 21119, 21133, 21153, 21193]}, {"Fips"=21121, "FipsAdj"=[21013, 21051, 21121, 21125]}, {"Fips"=21123, "FipsAdj"=[21087, 21093, 21099, 21123, 21155, 21179]}, {"Fips"=21125, "FipsAdj"=[21051, 21109, 21121, 21125, 21147, 21199, 21203]}, {"Fips"=21127, "FipsAdj"=[21019, 21043, 21063, 21115, 21127, 21159, 21175]}, {"Fips"=21129, "FipsAdj"=[21025, 21065, 21109, 21129, 21189, 21197]}, {"Fips"=21131, "FipsAdj"=[21013, 21051, 21095, 21131]}, {"Fips"=21133, "FipsAdj"=[21095, 21119, 21133, 21193, 21195]}, {"Fips"=21135, "FipsAdj"=[21043, 21069, 21089, 21135, 21161, 21205, 39001]}, {"Fips"=21137, "FipsAdj"=[21021, 21045, 21079, 21137, 21199]}, {"Fips"=21139, "FipsAdj"=[17069, 17127, 17151, 21055, 21139, 21143, 21145]}, {"Fips"=21141, "FipsAdj"=[21031, 21141, 21177, 21213, 21219, 21227]}, {"Fips"=21143, "FipsAdj"=[21033, 21055, 21139, 21143, 21157]}, {"Fips"=21145, "FipsAdj"=[17127, 17153, 21007, 21039, 21083, 21139, 21145]}, {"Fips"=21147, "FipsAdj"=[21125, 21147, 21199, 21231, 21235, 47013]}, {"Fips"=21149, "FipsAdj"=[21059, 21101, 21107, 21149, 21177, 21183]}, {"Fips"=21151, "FipsAdj"=[21049, 21065, 21067, 21079, 21109, 21113, 21151]}, {"Fips"=21153, "FipsAdj"=[21025, 21071, 21115, 21119, 21153, 21175]}, {"Fips"=21155, "FipsAdj"=[21021, 21045, 21123, 21155, 21179, 21217]}, {"Fips"=21157, "FipsAdj"=[21035, 21083, 21139, 21143, 21145, 21157]}, {"Fips"=21159, "FipsAdj"=[21071, 21115, 21127, 21159, 21195, 54059]}, {"Fips"=21161, "FipsAdj"=[21023, 21069, 21135, 21161, 21201, 39001]}, {"Fips"=21163, "FipsAdj"=[18025, 18061, 18123, 21027, 21093]}, {"Fips"=21165, "FipsAdj"=[21011, 21165, 21173, 21175, 21197, 21205]}, {"Fips"=21167, "FipsAdj"=[21005, 21021, 21079, 21113, 21167, 21229]}, {"Fips"=21169, "FipsAdj"=[21001, 21009, 21057, 21087, 21099, 21169]}, {"Fips"=21171, "FipsAdj"=[21003, 21009, 21057, 21169, 21171, 47027]}, {"Fips"=21173, "FipsAdj"=[21011, 21017, 21049, 21165, 21173, 21181]}, {"Fips"=21175, "FipsAdj"=[21063, 21115, 21127, 21153, 21165, 21175, 21205]}, {"Fips"=21177, "FipsAdj"=[21031, 21047, 21107, 21141, 21149, 21177, 21183]}, {"Fips"=21179, "FipsAdj"=[21005, 21029, 21093, 21123, 21155, 21179, 21215]}, {"Fips"=21181, "FipsAdj"=[21011, 21017, 21069, 21097, 21173, 21181]}, {"Fips"=21183, "FipsAdj"=[21027, 21031, 21059, 21085, 21091, 21149, 21177]}, {"Fips"=21185, "FipsAdj"=[18019, 21103, 21111, 21185, 21211]}, {"Fips"=21187, "FipsAdj"=[21041, 21073, 21077, 21081, 21103, 21187]}, {"Fips"=21189, "FipsAdj"=[21025, 21051, 21109, 21129, 21189]}, {"Fips"=21191, "FipsAdj"=[21023, 21037, 21081, 21097, 21117, 21191]}, {"Fips"=21193, "FipsAdj"=[21025, 21051, 21095, 21119, 21131, 21133, 21189]}, {"Fips"=21195, "FipsAdj"=[21071, 21119, 21133, 21159, 21195, 51027, 51051, 51195]}, {"Fips"=21197, "FipsAdj"=[21049, 21065, 21129, 21165, 21173, 21197]}, {"Fips"=21199, "FipsAdj"=[21045, 21125, 21137, 21147, 21199, 21203, 21207]}, {"Fips"=21201, "FipsAdj"=[21023, 21069, 21097, 21161, 21181]}, {"Fips"=21203, "FipsAdj"=[21079, 21109, 21125, 21137, 21151, 21199]}, {"Fips"=21205, "FipsAdj"=[21011, 21043, 21063, 21069, 21135, 21165, 21175]}, {"Fips"=21207, "FipsAdj"=[21001, 21045, 21053, 21057, 21199, 21207]}, {"Fips"=21209, "FipsAdj"=[21017, 21067, 21073, 21081, 21097, 21187, 21209]}, {"Fips"=21211, "FipsAdj"=[21005, 21073, 21103, 21111, 21185, 21211]}, {"Fips"=21213, "FipsAdj"=[21003, 21141, 21213, 21227, 47147]}, {"Fips"=21215, "FipsAdj"=[21005, 21029, 21111, 21179, 21211]}, {"Fips"=21217, "FipsAdj"=[21001, 21045, 21087, 21123, 21155]}, {"Fips"=21219, "FipsAdj"=[21047, 21141, 21177, 21219, 47125]}, {"Fips"=21221, "FipsAdj"=[21033, 21035, 21047, 21143, 21157, 21221]}, {"Fips"=21223, "FipsAdj"=[18019, 18077, 21041, 21103, 21185]}, {"Fips"=21225, "FipsAdj"=[17059, 17069, 18129, 21055, 21101, 21225]}, {"Fips"=21227, "FipsAdj"=[21003, 21009, 21031, 21061, 21141, 21213]}, {"Fips"=21229, "FipsAdj"=[21005, 21021, 21155, 21167, 21179]}, {"Fips"=21231, "FipsAdj"=[21053, 21147, 21199, 21207, 21231, 47137]}, {"Fips"=21233, "FipsAdj"=[21033, 21055, 21101, 21107, 21149, 21225]}, {"Fips"=21235, "FipsAdj"=[21013, 21121, 21125, 21147, 21235, 47013]}, {"Fips"=21237, "FipsAdj"=[21025, 21129, 21153, 21165, 21175, 21197]}, {"Fips"=21239, "FipsAdj"=[21005, 21067, 21073, 21113, 21167, 21209]}, {"Fips"=22001, "FipsAdj"=[22001, 22039, 22053, 22055, 22097]}, {"Fips"=22003, "FipsAdj"=[22003, 22011, 22039, 22053, 22079]}, {"Fips"=22005, "FipsAdj"=[22005, 22007, 22033, 22047, 22063, 22093]}, {"Fips"=22007, "FipsAdj"=[22005, 22007, 22045, 22047, 22057, 22093, 22099, 22101]}, {"Fips"=22009, "FipsAdj"=[22009, 22025, 22029, 22039, 22059, 22077, 22079, 22097]}, {"Fips"=22011, "FipsAdj"=[22003, 22011, 22019, 22053, 22115]}, {"Fips"=22013, "FipsAdj"=[22013, 22015, 22027, 22049, 22061, 22069, 22081, 22119]}, {"Fips"=22015, "FipsAdj"=[5073, 5091, 22013, 22015, 22017, 22081]}, {"Fips"=22017, "FipsAdj"=[5091, 22015, 22017, 22031, 22081, 48067, 48203, 48315]}, {"Fips"=22019, "FipsAdj"=[22011, 22019, 22023, 22053, 48351]}, {"Fips"=22021, "FipsAdj"=[22021, 22025, 22041, 22049, 22059, 22073, 22083]}, {"Fips"=22023, "FipsAdj"=[22019, 22023, 22053, 22113, 48245]}, {"Fips"=22025, "FipsAdj"=[22009, 22021, 22025, 22029, 22041, 22059]}, {"Fips"=22027, "FipsAdj"=[5027, 5139, 22013, 22027, 22061, 22111]}, {"Fips"=22029, "FipsAdj"=[22009, 22025, 22029, 22077, 22107, 22125, 28001]}, {"Fips"=22031, "FipsAdj"=[22017, 22031, 22069, 22081, 22085, 48365]}, {"Fips"=22033, "FipsAdj"=[22005, 22033, 22037, 22047, 22063, 22091]}, {"Fips"=22035, "FipsAdj"=[5017, 22035, 22065, 22083, 22123, 28055]}, {"Fips"=22037, "FipsAdj"=[22033, 22037, 22091, 22121, 22125, 28005]}, {"Fips"=22039, "FipsAdj"=[22001, 22003, 22009, 22039, 22053, 22079]}, {"Fips"=22041, "FipsAdj"=[22021, 22025, 22041, 22065, 22083]}, {"Fips"=22043, "FipsAdj"=[22043, 22059, 22069, 22079]}, {"Fips"=22045, "FipsAdj"=[22007, 22045, 22047, 22055, 22099, 22101]}, {"Fips"=22047, "FipsAdj"=[22005, 22007, 22033, 22045, 22047, 22077, 22099]}, {"Fips"=22049, "FipsAdj"=[22013, 22021, 22049, 22061, 22073]}, {"Fips"=22051, "FipsAdj"=[22051, 22057, 22071, 22075, 22089, 22095, 22103]}, {"Fips"=22053, "FipsAdj"=[22001, 22003, 22011, 22019, 22023, 22039, 22053]}, {"Fips"=22055, "FipsAdj"=[22001, 22045, 22055, 22097, 22099]}, {"Fips"=22057, "FipsAdj"=[22007, 22051, 22057, 22089, 22093, 22095]}, {"Fips"=22059, "FipsAdj"=[22009, 22021, 22025, 22043, 22059, 22079]}, {"Fips"=22061, "FipsAdj"=[22013, 22027, 22049, 22061, 22073]}, {"Fips"=22063, "FipsAdj"=[22005, 22033, 22063, 22091, 22095]}, {"Fips"=22065, "FipsAdj"=[22035, 22041, 22065, 22083, 22107]}, {"Fips"=22067, "FipsAdj"=[5003, 5017, 5139, 22067, 22073, 22083, 22111]}, {"Fips"=22069, "FipsAdj"=[22013, 22031, 22043, 22069, 22079, 22081, 22085, 22115]}, {"Fips"=22071, "FipsAdj"=[22051, 22071, 22075, 22087]}, {"Fips"=22073, "FipsAdj"=[22021, 22049, 22061, 22067, 22073, 22083]}, {"Fips"=22075, "FipsAdj"=[22051, 22071, 22075]}, {"Fips"=22077, "FipsAdj"=[22009, 22029, 22047, 22077, 22097, 22099, 22121]}, {"Fips"=22079, "FipsAdj"=[22003, 22009, 22039, 22043, 22059, 22069, 22079]}, {"Fips"=22081, "FipsAdj"=[22013, 22015, 22017, 22031, 22069]}, {"Fips"=22083, "FipsAdj"=[22021, 22035, 22041, 22065, 22067, 22073, 22083]}, {"Fips"=22085, "FipsAdj"=[22031, 22069, 22085, 22115, 48351, 48403]}, {"Fips"=22087, "FipsAdj"=[22071, 22075, 22087, 22103, 28045]}, {"Fips"=22089, "FipsAdj"=[22051, 22057, 22089, 22095]}, {"Fips"=22091, "FipsAdj"=[22033, 22037, 22063, 22091, 22105]}, {"Fips"=22093, "FipsAdj"=[22005, 22007, 22057, 22093]}, {"Fips"=22095, "FipsAdj"=[22005, 22051, 22057, 22063, 22089, 22093, 22095]}, {"Fips"=22097, "FipsAdj"=[22001, 22009, 22039, 22055, 22077, 22097]}, {"Fips"=22099, "FipsAdj"=[22007, 22045, 22047, 22055, 22077, 22097, 22099]}, {"Fips"=22101, "FipsAdj"=[22007, 22045, 22099, 22101]}, {"Fips"=22103, "FipsAdj"=[22051, 22071, 22087, 22103, 22105, 22117, 28045]}, {"Fips"=22105, "FipsAdj"=[22051, 22063, 22089, 22091, 22095, 22103, 22105, 22117, 28005]}, {"Fips"=22107, "FipsAdj"=[22025, 22029, 22041, 22065, 22107, 28001, 28021, 28063]}, {"Fips"=22109, "FipsAdj"=[22007, 22057, 22101]}, {"Fips"=22111, "FipsAdj"=[5003, 5139, 22027, 22061, 22067, 22073]}, {"Fips"=22113, "FipsAdj"=[22001, 22023, 22045, 22053, 22055]}, {"Fips"=22115, "FipsAdj"=[22003, 22011, 22069, 22079, 22085, 22115]}, {"Fips"=22117, "FipsAdj"=[22103, 22105, 22117, 28091, 28109, 28113]}, {"Fips"=22119, "FipsAdj"=[5027, 5073, 22013, 22015, 22027]}, {"Fips"=22121, "FipsAdj"=[22033, 22037, 22047, 22077, 22121]}, {"Fips"=22123, "FipsAdj"=[5017, 22035, 22067, 22083]}, {"Fips"=22125, "FipsAdj"=[22009, 22029, 22037, 22077, 22121, 22125]}, {"Fips"=22127, "FipsAdj"=[22013, 22021, 22043, 22049, 22059, 22069]}, {"Fips"=23001, "FipsAdj"=[23001, 23005, 23007, 23011, 23017]}, {"Fips"=23003, "FipsAdj"=[23003, 23019, 23021, 23025]}, {"Fips"=23005, "FipsAdj"=[23001, 23005, 23017, 23023]}, {"Fips"=23007, "FipsAdj"=[23001, 23007, 23011, 23017]}, {"Fips"=23009, "FipsAdj"=[23009, 23013, 23019, 23027]}, {"Fips"=23011, "FipsAdj"=[23001, 23007, 23011, 23015, 23023, 23025]}, {"Fips"=23013, "FipsAdj"=[23009, 23013, 23015]}, {"Fips"=23015, "FipsAdj"=[23011, 23013, 23015, 23023]}, {"Fips"=23017, "FipsAdj"=[23001, 23005, 23007, 23017, 23031, 33003]}, {"Fips"=23019, "FipsAdj"=[23003, 23009, 23019, 23021, 23025, 23027]}, {"Fips"=23021, "FipsAdj"=[23003, 23019, 23021]}, {"Fips"=23023, "FipsAdj"=[23001, 23005, 23011, 23015]}, {"Fips"=23025, "FipsAdj"=[23003, 23007, 23011, 23019, 23021, 23025]}, {"Fips"=23027, "FipsAdj"=[23009, 23011, 23013, 23015, 23019, 23025]}, {"Fips"=23029, "FipsAdj"=[23003, 23009, 23019]}, {"Fips"=23031, "FipsAdj"=[23005, 23017, 23031, 33003, 33015]}, {"Fips"=24001, "FipsAdj"=[24001, 24023, 24043, 42009, 42057, 42111, 54027, 54057]}, {"Fips"=24003, "FipsAdj"=[24003, 24005, 24009, 24027, 24029, 24033, 24035, 24041]}, {"Fips"=24005, "FipsAdj"=[24003, 24005, 24013, 24025, 24027, 24029, 24510]}, {"Fips"=24009, "FipsAdj"=[24003, 24009, 24017, 24019, 24033, 24037]}, {"Fips"=24011, "FipsAdj"=[10001, 10005, 24011, 24019, 24035]}, {"Fips"=24013, "FipsAdj"=[24005, 24013, 24021, 24027, 42001]}, {"Fips"=24015, "FipsAdj"=[10003, 24015, 24025, 24029, 42029]}, {"Fips"=24017, "FipsAdj"=[24009, 24017, 24033, 24037, 51059, 51099, 51153, 51179]}, {"Fips"=24019, "FipsAdj"=[10005, 24009, 24011, 24019, 24037, 24039, 24041]}, {"Fips"=24021, "FipsAdj"=[24013, 24021, 24027, 24031, 24043, 42001, 42055]}, {"Fips"=24023, "FipsAdj"=[24001, 24023, 42051, 42111, 54023, 54057]}, {"Fips"=24025, "FipsAdj"=[24005, 24015, 24025, 24029, 42071]}, {"Fips"=24027, "FipsAdj"=[24003, 24005, 24013, 24021, 24027, 24031]}, {"Fips"=24029, "FipsAdj"=[10001, 10003, 24003, 24005, 24015, 24025, 24029]}, {"Fips"=24031, "FipsAdj"=[11001, 24021, 24027, 24031, 24033, 51013, 51059]}, {"Fips"=24033, "FipsAdj"=[11001, 24003, 24009, 24017, 24027, 24031, 24033, 51059]}, {"Fips"=24035, "FipsAdj"=[10001, 24003, 24011, 24029, 24035]}, {"Fips"=24037, "FipsAdj"=[24009, 24017, 24019, 24037, 24039, 51133]}, {"Fips"=24039, "FipsAdj"=[24019, 24037, 24039, 24045, 24047, 51001]}, {"Fips"=24041, "FipsAdj"=[24003, 24009, 24011, 24019, 24035]}, {"Fips"=24043, "FipsAdj"=[24001, 24021, 24043, 42055, 42057, 51107, 54003, 54037]}, {"Fips"=24045, "FipsAdj"=[10005, 24019, 24039, 24045]}, {"Fips"=24047, "FipsAdj"=[10005, 24039, 24045, 24047]}, {"Fips"=24510, "FipsAdj"=[24003, 24005]}, {"Fips"=25001, "FipsAdj"=[25001, 25005, 25007]}, {"Fips"=25003, "FipsAdj"=[9005, 25003, 25011, 25013, 25015, 36021, 36027, 36083]}, {"Fips"=25005, "FipsAdj"=[25001, 25005, 25007, 25021, 25023, 44001, 44005]}, {"Fips"=25007, "FipsAdj"=[25001, 25005, 25007]}, {"Fips"=25009, "FipsAdj"=[25009, 25017, 25025, 33011]}, {"Fips"=25011, "FipsAdj"=[25003, 25011, 25015, 25027, 33005, 50003]}, {"Fips"=25013, "FipsAdj"=[9003, 9005, 9013, 25003, 25013, 25015]}, {"Fips"=25015, "FipsAdj"=[25003, 25011, 25013, 25015]}, {"Fips"=25017, "FipsAdj"=[25009, 25017, 25021, 25025, 25027]}, {"Fips"=25019, "FipsAdj"=[25007]}, {"Fips"=25021, "FipsAdj"=[25005, 25017, 25021, 25023, 25025, 25027]}, {"Fips"=25023, "FipsAdj"=[25001, 25005, 25021, 25023]}, {"Fips"=25025, "FipsAdj"=[25009, 25017, 25021, 25023]}, {"Fips"=25027, "FipsAdj"=[9013, 9015, 25011, 25013, 25015, 25017, 25021, 25027, 33005, 33011]}, {"Fips"=26001, "FipsAdj"=[26001, 26007, 26069, 26119, 26129]}, {"Fips"=26003, "FipsAdj"=[26003, 26041, 26083, 26095, 26103]}, {"Fips"=26005, "FipsAdj"=[17097, 26005, 26015, 26077, 26081, 26139, 26159, 55059]}, {"Fips"=26007, "FipsAdj"=[26001, 26007, 26119, 26135]}, {"Fips"=26009, "FipsAdj"=[26009, 26029, 26039, 26055, 26079, 26089]}, {"Fips"=26011, "FipsAdj"=[26011, 26017, 26051, 26063, 26069]}, {"Fips"=26013, "FipsAdj"=[26013, 26061, 26071]}, {"Fips"=26015, "FipsAdj"=[26005, 26015, 26025, 26045, 26067, 26077]}, {"Fips"=26017, "FipsAdj"=[26011, 26017, 26051, 26063, 26111, 26145]}, {"Fips"=26019, "FipsAdj"=[26019, 26055, 26089, 26101, 26165, 55029]}, {"Fips"=26021, "FipsAdj"=[17031, 17097, 18091, 18127, 18141, 26021, 26027]}, {"Fips"=26023, "FipsAdj"=[18087, 18151, 26023, 26025, 26059, 26077]}, {"Fips"=26025, "FipsAdj"=[26015, 26023, 26025, 26045, 26059, 26075, 26077]}, {"Fips"=26027, "FipsAdj"=[18039, 18141, 26021, 26027, 26077, 26149]}, {"Fips"=26029, "FipsAdj"=[26009, 26029, 26031, 26047, 26089, 26097, 26137]}, {"Fips"=26031, "FipsAdj"=[26029, 26031, 26047, 26097, 26119, 26137]}, {"Fips"=26033, "FipsAdj"=[26033, 26095, 26097]}, {"Fips"=26035, "FipsAdj"=[26035, 26051, 26073, 26107, 26111, 26113, 26133]}, {"Fips"=26037, "FipsAdj"=[26037, 26045, 26057, 26065, 26067, 26117]}, {"Fips"=26039, "FipsAdj"=[26009, 26039, 26079, 26113, 26119, 26129, 26135, 26137]}, {"Fips"=26041, "FipsAdj"=[26003, 26041, 26089, 26103, 26109, 26153]}, {"Fips"=26043, "FipsAdj"=[26043, 26071, 26103, 26109, 55037]}, {"Fips"=26045, "FipsAdj"=[26015, 26025, 26037, 26045, 26065, 26067]}, {"Fips"=26047, "FipsAdj"=[26029, 26031, 26047]}, {"Fips"=26049, "FipsAdj"=[26049, 26087, 26093, 26125, 26145, 26155]}, {"Fips"=26051, "FipsAdj"=[26011, 26017, 26035, 26051, 26073, 26111, 26129]}, {"Fips"=26053, "FipsAdj"=[26053, 26071, 26131, 55003, 55051]}, {"Fips"=26055, "FipsAdj"=[26009, 26019, 26055, 26079, 26089, 26101, 26113]}, {"Fips"=26057, "FipsAdj"=[26037, 26057, 26067, 26073, 26111, 26117, 26145]}, {"Fips"=26059, "FipsAdj"=[18151, 26023, 26025, 26059, 26075, 26091, 39051]}, {"Fips"=26061, "FipsAdj"=[26013, 26061, 26071, 26083, 26103]}, {"Fips"=26063, "FipsAdj"=[26011, 26017, 26063, 26069, 26151]}, {"Fips"=26065, "FipsAdj"=[26037, 26045, 26065, 26075, 26093]}, {"Fips"=26067, "FipsAdj"=[26015, 26037, 26045, 26057, 26067, 26081]}, {"Fips"=26069, "FipsAdj"=[26001, 26011, 26063, 26069, 26129]}, {"Fips"=26071, "FipsAdj"=[26013, 26043, 26053, 26061, 26071, 26103, 26131, 55037, 55041]}, {"Fips"=26073, "FipsAdj"=[26035, 26051, 26057, 26073, 26107, 26111, 26117]}, {"Fips"=26075, "FipsAdj"=[26025, 26045, 26059, 26065, 26075, 26091, 26093]}, {"Fips"=26077, "FipsAdj"=[26005, 26015, 26023, 26025, 26027, 26077, 26149]}, {"Fips"=26079, "FipsAdj"=[26009, 26039, 26055, 26079, 26113, 26137, 26143]}, {"Fips"=26081, "FipsAdj"=[26005, 26015, 26067, 26081, 26117, 26121, 26123]}, {"Fips"=26083, "FipsAdj"=[26003, 26061, 26083, 26103, 26131]}, {"Fips"=26085, "FipsAdj"=[26085, 26101, 26105, 26107, 26123, 26127, 26133]}, {"Fips"=26087, "FipsAdj"=[26049, 26087, 26099, 26125, 26147, 26151]}, {"Fips"=26089, "FipsAdj"=[26009, 26019, 26029, 26041, 26055, 26089, 26153]}, {"Fips"=26091, "FipsAdj"=[26059, 26075, 26091, 26115, 26161, 39051]}, {"Fips"=26093, "FipsAdj"=[26049, 26065, 26075, 26093, 26125, 26155]}, {"Fips"=26095, "FipsAdj"=[26003, 26033, 26095, 26097]}, {"Fips"=26097, "FipsAdj"=[26029, 26031, 26033, 26047, 26095, 26097, 26141]}, {"Fips"=26099, "FipsAdj"=[26087, 26099, 26125, 26147]}, {"Fips"=26101, "FipsAdj"=[26019, 26055, 26085, 26101, 26105, 26165, 55061]}, {"Fips"=26103, "FipsAdj"=[26003, 26013, 26041, 26043, 26061, 26071, 26083, 26103]}, {"Fips"=26105, "FipsAdj"=[26085, 26101, 26105, 26123, 26127, 55071]}, {"Fips"=26107, "FipsAdj"=[26035, 26073, 26085, 26107, 26117, 26123]}, {"Fips"=26109, "FipsAdj"=[26041, 26043, 26103, 26109, 55029]}, {"Fips"=26111, "FipsAdj"=[26017, 26035, 26051, 26057, 26073, 26111]}, {"Fips"=26113, "FipsAdj"=[26035, 26039, 26055, 26079, 26113, 26133, 26143]}, {"Fips"=26115, "FipsAdj"=[26091, 26115, 26161, 26163]}, {"Fips"=26117, "FipsAdj"=[26037, 26057, 26067, 26073, 26081, 26107, 26117]}, {"Fips"=26119, "FipsAdj"=[26001, 26007, 26031, 26039, 26119, 26135, 26137]}, {"Fips"=26121, "FipsAdj"=[26081, 26121, 26123, 26127, 26139, 55079]}, {"Fips"=26123, "FipsAdj"=[26081, 26085, 26105, 26107, 26117, 26121, 26123, 26127]}, {"Fips"=26125, "FipsAdj"=[26049, 26087, 26093, 26099, 26125, 26161]}, {"Fips"=26127, "FipsAdj"=[26085, 26105, 26121, 26123, 26127, 55089]}, {"Fips"=26129, "FipsAdj"=[26001, 26011, 26039, 26051, 26069, 26129, 26135]}, {"Fips"=26131, "FipsAdj"=[26053, 26061, 26071, 26083, 26131, 27031]}, {"Fips"=26133, "FipsAdj"=[26035, 26073, 26085, 26107, 26113, 26123, 26133]}, {"Fips"=26135, "FipsAdj"=[26001, 26007, 26039, 26069, 26119, 26129, 26135, 26137]}, {"Fips"=26137, "FipsAdj"=[26009, 26029, 26031, 26039, 26079, 26119, 26135]}, {"Fips"=26139, "FipsAdj"=[26005, 26081, 26121, 26139, 55079]}, {"Fips"=26141, "FipsAdj"=[26007, 26031, 26033, 26097, 26119]}, {"Fips"=26143, "FipsAdj"=[26035, 26039, 26051, 26079, 26113, 26129, 26135]}, {"Fips"=26145, "FipsAdj"=[26017, 26049, 26057, 26111, 26145, 26155]}, {"Fips"=26147, "FipsAdj"=[26087, 26099, 26147]}, {"Fips"=26149, "FipsAdj"=[18039, 18087, 26023, 26025, 26027, 26077, 26149]}, {"Fips"=26151, "FipsAdj"=[26063, 26087, 26147, 26151]}, {"Fips"=26153, "FipsAdj"=[26003, 26029, 26041, 26089, 26095, 26097]}, {"Fips"=26155, "FipsAdj"=[26037, 26049, 26057, 26065, 26093, 26145]}, {"Fips"=26157, "FipsAdj"=[26017, 26049, 26063, 26087, 26145, 26151]}, {"Fips"=26159, "FipsAdj"=[17097, 26005, 26021, 26027, 26077, 26149]}, {"Fips"=26161, "FipsAdj"=[26075, 26091, 26093, 26115, 26125, 26161]}, {"Fips"=26163, "FipsAdj"=[26099, 26115, 26125, 26161]}, {"Fips"=26165, "FipsAdj"=[26019, 26055, 26079, 26085, 26101, 26113, 26133]}, {"Fips"=27001, "FipsAdj"=[27001, 27017, 27021, 27035, 27061, 27065, 27095, 27115]}, {"Fips"=27003, "FipsAdj"=[27003, 27025, 27053, 27059, 27123, 27141]}, {"Fips"=27005, "FipsAdj"=[27005, 27027, 27029, 27057, 27087, 27107, 27111]}, {"Fips"=27007, "FipsAdj"=[27007, 27021, 27029, 27057, 27061, 27071, 27077, 27089, 27113]}, {"Fips"=27009, "FipsAdj"=[27009, 27095, 27097, 27141]}, {"Fips"=27011, "FipsAdj"=[27011, 27073, 27149, 27151, 27155, 46051]}, {"Fips"=27013, "FipsAdj"=[27013, 27015, 27043, 27079, 27091, 27103, 27161]}, {"Fips"=27015, "FipsAdj"=[27013, 27015, 27033, 27103, 27127, 27129]}, {"Fips"=27017, "FipsAdj"=[27001, 27017, 27115, 27137]}, {"Fips"=27019, "FipsAdj"=[27019, 27053, 27085, 27139, 27143]}, {"Fips"=27021, "FipsAdj"=[27001, 27007, 27021, 27035, 27057, 27061, 27097, 27153]}, {"Fips"=27023, "FipsAdj"=[27023, 27067, 27073, 27129, 27151]}, {"Fips"=27025, "FipsAdj"=[27003, 27025, 27059, 27065, 27115, 27163, 55013]}, {"Fips"=27027, "FipsAdj"=[27005, 27027, 27107, 27111, 27167, 38017]}, {"Fips"=27029, "FipsAdj"=[27005, 27007, 27029, 27057, 27087, 27113]}, {"Fips"=27031, "FipsAdj"=[26083, 26131, 27031, 27075]}, {"Fips"=27033, "FipsAdj"=[27015, 27033, 27063, 27101, 27105, 27127]}, {"Fips"=27035, "FipsAdj"=[27001, 27021, 27035, 27095]}, {"Fips"=27037, "FipsAdj"=[27037, 27049, 27053, 27123, 27131, 27139, 27163]}, {"Fips"=27039, "FipsAdj"=[27039, 27049, 27099, 27109, 27131]}, {"Fips"=27041, "FipsAdj"=[27041, 27051, 27111, 27121, 27145, 27149]}, {"Fips"=27043, "FipsAdj"=[19109, 19189, 27013, 27043, 27047, 27091]}, {"Fips"=27045, "FipsAdj"=[19089, 19191, 27045, 27055, 27099, 27109]}, {"Fips"=27047, "FipsAdj"=[19189, 19195, 27043, 27047, 27099, 27147]}, {"Fips"=27049, "FipsAdj"=[27037, 27039, 27049, 27109, 27131, 27157, 55091]}, {"Fips"=27051, "FipsAdj"=[27041, 27051, 27111, 27121, 27149, 27155]}, {"Fips"=27053, "FipsAdj"=[27003, 27019, 27037, 27053, 27123, 27139, 27141]}, {"Fips"=27055, "FipsAdj"=[19005, 19191, 27045, 27055, 27169, 55063]}, {"Fips"=27057, "FipsAdj"=[27005, 27007, 27021, 27029, 27057]}, {"Fips"=27059, "FipsAdj"=[27003, 27025, 27059, 27065, 27095, 27115]}, {"Fips"=27061, "FipsAdj"=[27001, 27007, 27021, 27061, 27071]}, {"Fips"=27063, "FipsAdj"=[19059, 19063, 19143, 27033, 27063, 27091, 27105]}, {"Fips"=27065, "FipsAdj"=[27001, 27025, 27059, 27065, 27095]}, {"Fips"=27067, "FipsAdj"=[27023, 27067, 27093, 27121, 27129, 27145]}, {"Fips"=27069, "FipsAdj"=[27069, 27089, 27135]}, {"Fips"=27071, "FipsAdj"=[27007, 27061, 27071, 27077]}, {"Fips"=27073, "FipsAdj"=[27011, 27023, 27073, 27151, 27173, 46039]}, {"Fips"=27075, "FipsAdj"=[27031, 27075, 27137, 55003, 55007]}, {"Fips"=27077, "FipsAdj"=[27007, 27071, 27077]}, {"Fips"=27079, "FipsAdj"=[27013, 27079, 27103, 27131, 27139, 27143]}, {"Fips"=27081, "FipsAdj"=[27081, 27083, 27117, 27173, 46011, 46039]}, {"Fips"=27083, "FipsAdj"=[27081, 27083, 27101, 27117, 27127]}, {"Fips"=27085, "FipsAdj"=[27019, 27085, 27093, 27129, 27143]}, {"Fips"=27087, "FipsAdj"=[27005, 27029, 27087, 27107]}, {"Fips"=27089, "FipsAdj"=[27007, 27069, 27089, 27113, 27119, 27135, 38035, 38067]}, {"Fips"=27091, "FipsAdj"=[19063, 19109, 27013, 27043, 27063, 27091]}, {"Fips"=27093, "FipsAdj"=[27067, 27085, 27093, 27129, 27145]}, {"Fips"=27095, "FipsAdj"=[27001, 27009, 27035, 27059, 27065, 27095, 27097]}, {"Fips"=27097, "FipsAdj"=[27009, 27021, 27035, 27095, 27097, 27145]}, {"Fips"=27099, "FipsAdj"=[19089, 19131, 19195, 27039, 27045, 27047, 27099, 27109]}, {"Fips"=27101, "FipsAdj"=[27033, 27083, 27101, 27105, 27117, 27127]}, {"Fips"=27103, "FipsAdj"=[27013, 27015, 27079, 27103, 27129]}, {"Fips"=27105, "FipsAdj"=[19119, 19143, 27033, 27063, 27101, 27105]}, {"Fips"=27107, "FipsAdj"=[27005, 27027, 27087, 27107, 27119, 38017]}, {"Fips"=27109, "FipsAdj"=[27039, 27045, 27049, 27099, 27109, 27157]}, {"Fips"=27111, "FipsAdj"=[27005, 27027, 27041, 27051, 27111, 27153, 27159]}, {"Fips"=27113, "FipsAdj"=[27007, 27029, 27089, 27113, 27119]}, {"Fips"=27115, "FipsAdj"=[27001, 27017, 27025, 27059, 27065, 27115, 55013]}, {"Fips"=27117, "FipsAdj"=[27081, 27083, 27101, 27117, 27133, 46011, 46099]}, {"Fips"=27119, "FipsAdj"=[27029, 27087, 27089, 27107, 27113, 27119, 27125, 38035]}, {"Fips"=27121, "FipsAdj"=[27041, 27051, 27067, 27121, 27145, 27149]}, {"Fips"=27123, "FipsAdj"=[27003, 27037, 27053, 27123]}, {"Fips"=27125, "FipsAdj"=[27113, 27119]}, {"Fips"=27127, "FipsAdj"=[27015, 27033, 27083, 27101, 27127, 27129]}, {"Fips"=27129, "FipsAdj"=[27015, 27023, 27067, 27085, 27093, 27103, 27127, 27129, 27143]}, {"Fips"=27131, "FipsAdj"=[27037, 27039, 27049, 27079, 27131, 27139, 27147]}, {"Fips"=27133, "FipsAdj"=[19119, 27101, 27105, 27117, 27133, 46099]}, {"Fips"=27135, "FipsAdj"=[27007, 27069, 27077, 27089]}, {"Fips"=27137, "FipsAdj"=[27001, 27017, 27061, 27071, 27075, 27137]}, {"Fips"=27139, "FipsAdj"=[27019, 27037, 27053, 27079, 27131, 27139]}, {"Fips"=27141, "FipsAdj"=[27003, 27009, 27053, 27059, 27095, 27141, 27145]}, {"Fips"=27143, "FipsAdj"=[27019, 27079, 27085, 27103, 27129, 27139]}, {"Fips"=27145, "FipsAdj"=[27009, 27041, 27067, 27093, 27097, 27121, 27141, 27145, 27153]}, {"Fips"=27147, "FipsAdj"=[27039, 27047, 27099, 27131, 27147]}, {"Fips"=27149, "FipsAdj"=[27011, 27041, 27051, 27121, 27149, 27151]}, {"Fips"=27151, "FipsAdj"=[27011, 27023, 27067, 27073, 27121, 27149]}, {"Fips"=27153, "FipsAdj"=[27021, 27041, 27097, 27111, 27145, 27153]}, {"Fips"=27155, "FipsAdj"=[27011, 27051, 27149, 27155, 27167, 38077]}, {"Fips"=27157, "FipsAdj"=[27049, 27109, 27157, 27169, 55011]}, {"Fips"=27159, "FipsAdj"=[27005, 27021, 27057, 27111, 27153]}, {"Fips"=27161, "FipsAdj"=[27013, 27043, 27047, 27079, 27131, 27147]}, {"Fips"=27163, "FipsAdj"=[27003, 27025, 27037, 27123, 27163, 55093, 55095]}, {"Fips"=27165, "FipsAdj"=[]}, {"Fips"=27163, "FipsAdj"=[27015, 27033, 27063, 27091]}, {"Fips"=27167, "FipsAdj"=[27027, 27051, 27111, 27155, 27167]}, {"Fips"=27169, "FipsAdj"=[27045, 27055, 27109, 27157, 27169, 55011, 55063]}, {"Fips"=27171, "FipsAdj"=[27019, 27053, 27085, 27093, 27141, 27145]}, {"Fips"=27173, "FipsAdj"=[27023, 27073, 27081, 27083, 27127, 27129, 27173]}, {"Fips"=28001, "FipsAdj"=[22029, 22107, 28001, 28037, 28063]}, {"Fips"=28003, "FipsAdj"=[28003, 28117, 28139, 28141, 47069, 47071]}, {"Fips"=28005, "FipsAdj"=[22037, 22091, 22105, 28005, 28037, 28085, 28113]}, {"Fips"=28007, "FipsAdj"=[28007, 28015, 28019, 28051, 28079, 28089, 28097, 28099, 28159]}, {"Fips"=28009, "FipsAdj"=[28009, 28093, 28139, 28145, 47047]}, {"Fips"=28011, "FipsAdj"=[5017, 5041, 5107, 28011, 28027, 28133]}, {"Fips"=28013, "FipsAdj"=[28013, 28017, 28043, 28071, 28115, 28155]}, {"Fips"=28015, "FipsAdj"=[28007, 28015, 28043, 28051, 28083]}, {"Fips"=28017, "FipsAdj"=[28013, 28017, 28025, 28081, 28095, 28115]}, {"Fips"=28019, "FipsAdj"=[28007, 28019, 28097, 28105, 28155]}, {"Fips"=28021, "FipsAdj"=[22107, 28021, 28029, 28049, 28063]}, {"Fips"=28023, "FipsAdj"=[1023, 28023, 28061, 28075, 28101]}, {"Fips"=28025, "FipsAdj"=[28017, 28025, 28087, 28095, 28105]}, {"Fips"=28027, "FipsAdj"=[5107, 28011, 28027, 28119, 28133, 28135]}, {"Fips"=28029, "FipsAdj"=[28021, 28029, 28049, 28063, 28077, 28085, 28121]}, {"Fips"=28031, "FipsAdj"=[28031, 28035, 28065, 28067, 28073, 28127]}, {"Fips"=28033, "FipsAdj"=[5035, 28033, 28093, 28137, 28143]}, {"Fips"=28035, "FipsAdj"=[28031, 28035, 28067, 28073, 28109, 28111]}, {"Fips"=28037, "FipsAdj"=[28001, 28005, 28037, 28063, 28085]}, {"Fips"=28039, "FipsAdj"=[1097, 28039, 28041, 28059, 28111]}, {"Fips"=28041, "FipsAdj"=[1097, 1129, 28039, 28041, 28111]}, {"Fips"=28043, "FipsAdj"=[28013, 28015, 28043, 28083, 28097, 28135, 28155]}, {"Fips"=28045, "FipsAdj"=[22087, 22103, 28045, 28047, 28109]}, {"Fips"=28047, "FipsAdj"=[22087, 28045, 28047, 28059, 28109]}, {"Fips"=28049, "FipsAdj"=[28021, 28029, 28049, 28089, 28121, 28127, 28149]}, {"Fips"=28051, "FipsAdj"=[28007, 28015, 28051, 28053, 28083, 28089]}, {"Fips"=28053, "FipsAdj"=[28051, 28053, 28083, 28125, 28133, 28151]}, {"Fips"=28055, "FipsAdj"=[5017, 22035, 28055, 28125, 28149, 28151]}, {"Fips"=28057, "FipsAdj"=[1059, 1093, 28057, 28081, 28095, 28117]}, {"Fips"=28059, "FipsAdj"=[1097, 28039, 28047, 28059]}, {"Fips"=28061, "FipsAdj"=[28023, 28061, 28067, 28075, 28101, 28123, 28129]}, {"Fips"=28063, "FipsAdj"=[22107, 28001, 28021, 28029, 28037, 28063]}, {"Fips"=28065, "FipsAdj"=[28031, 28065, 28073, 28077, 28091]}, {"Fips"=28067, "FipsAdj"=[28031, 28035, 28061, 28067, 28111, 28129]}, {"Fips"=28069, "FipsAdj"=[1119, 28069, 28075, 28099, 28101, 28103]}, {"Fips"=28071, "FipsAdj"=[28013, 28071, 28093, 28107, 28115, 28137, 28145]}, {"Fips"=28073, "FipsAdj"=[28031, 28035, 28065, 28073, 28091]}, {"Fips"=28075, "FipsAdj"=[1023, 1119, 28023, 28061, 28069, 28075, 28099]}, {"Fips"=28077, "FipsAdj"=[28029, 28065, 28077, 28085, 28091, 28127]}, {"Fips"=28079, "FipsAdj"=[28007, 28079, 28089, 28099, 28101, 28123]}, {"Fips"=28081, "FipsAdj"=[28017, 28057, 28081, 28095, 28115, 28117]}, {"Fips"=28083, "FipsAdj"=[28015, 28043, 28051, 28053, 28083, 28133]}, {"Fips"=28085, "FipsAdj"=[28005, 28029, 28037, 28063, 28077, 28085, 28113]}, {"Fips"=28087, "FipsAdj"=[1075, 1107, 28025, 28087, 28095, 28103]}, {"Fips"=28089, "FipsAdj"=[28007, 28049, 28051, 28079, 28089, 28121, 28123]}, {"Fips"=28091, "FipsAdj"=[22117, 28065, 28073, 28077, 28091, 28109]}, {"Fips"=28093, "FipsAdj"=[28009, 28033, 28071, 28093, 28137, 28145, 47047]}, {"Fips"=28095, "FipsAdj"=[1075, 1093, 28017, 28025, 28057, 28081, 28087]}, {"Fips"=28097, "FipsAdj"=[28007, 28015, 28019, 28043, 28097]}, {"Fips"=28099, "FipsAdj"=[28007, 28069, 28075, 28079, 28099, 28101]}, {"Fips"=28101, "FipsAdj"=[28023, 28061, 28069, 28075, 28079, 28099, 28101, 28123]}, {"Fips"=28103, "FipsAdj"=[1107, 1119, 28069, 28087, 28103, 28105]}, {"Fips"=28105, "FipsAdj"=[28019, 28025, 28087, 28103, 28105, 28155]}, {"Fips"=28107, "FipsAdj"=[28071, 28107, 28119, 28135, 28137, 28143]}, {"Fips"=28109, "FipsAdj"=[22103, 22117, 28035, 28045, 28047, 28073, 28091, 28109]}, {"Fips"=28111, "FipsAdj"=[28035, 28039, 28041, 28067, 28111, 28131]}, {"Fips"=28113, "FipsAdj"=[22105, 22117, 28005, 28085, 28113]}, {"Fips"=28115, "FipsAdj"=[28013, 28017, 28071, 28081, 28115]}, {"Fips"=28117, "FipsAdj"=[28003, 28057, 28081, 28117, 28139, 28141]}, {"Fips"=28119, "FipsAdj"=[28027, 28107, 28119, 28135]}, {"Fips"=28121, "FipsAdj"=[28029, 28049, 28089, 28121, 28123, 28127]}, {"Fips"=28123, "FipsAdj"=[28061, 28079, 28089, 28101, 28121, 28123]}, {"Fips"=28125, "FipsAdj"=[28053, 28055, 28125, 28151]}, {"Fips"=28127, "FipsAdj"=[28029, 28031, 28049, 28065, 28077, 28121, 28127]}, {"Fips"=28129, "FipsAdj"=[28031, 28061, 28067, 28101, 28121, 28123, 28127]}, {"Fips"=28131, "FipsAdj"=[28035, 28039, 28045, 28047, 28059, 28109, 28111]}, {"Fips"=28133, "FipsAdj"=[28011, 28027, 28053, 28083, 28133, 28135]}, {"Fips"=28135, "FipsAdj"=[28027, 28043, 28083, 28107, 28119, 28133, 28135]}, {"Fips"=28137, "FipsAdj"=[28033, 28071, 28093, 28107, 28137]}, {"Fips"=28139, "FipsAdj"=[28003, 28009, 28117, 28139, 28145]}, {"Fips"=28141, "FipsAdj"=[1033, 1059, 1077, 28003, 28057, 28117, 28141]}, {"Fips"=28143, "FipsAdj"=[5035, 5077, 5107, 28027, 28033, 28107, 28119, 28137]}, {"Fips"=28145, "FipsAdj"=[28009, 28071, 28081, 28093, 28115, 28117, 28139]}, {"Fips"=28147, "FipsAdj"=[22117, 28077, 28085, 28091, 28113]}, {"Fips"=28149, "FipsAdj"=[22035, 22065, 22107, 28021, 28049, 28055, 28149]}, {"Fips"=28151, "FipsAdj"=[5017, 28011, 28053, 28055, 28125, 28133]}, {"Fips"=28153, "FipsAdj"=[1023, 1129, 28023, 28041, 28061, 28067, 28111]}, {"Fips"=28155, "FipsAdj"=[28013, 28017, 28019, 28025, 28043, 28097, 28105]}, {"Fips"=28157, "FipsAdj"=[22029, 22037, 22125, 28001, 28005, 28037]}, {"Fips"=28159, "FipsAdj"=[28007, 28019, 28069, 28079, 28099, 28103, 28105]}, {"Fips"=28161, "FipsAdj"=[28013, 28043, 28071, 28107, 28135]}, {"Fips"=28163, "FipsAdj"=[28007, 28049, 28051, 28053, 28055, 28089, 28125, 28149]}, {"Fips"=29001, "FipsAdj"=[29001, 29103, 29115, 29121, 29171, 29197, 29199]}, {"Fips"=29003, "FipsAdj"=[20043, 29003, 29021, 29063, 29075, 29087]}, {"Fips"=29005, "FipsAdj"=[19071, 19145, 29005, 29087, 29147, 31127]}, {"Fips"=29007, "FipsAdj"=[29007, 29019, 29027, 29137, 29139, 29163, 29173]}, {"Fips"=29009, "FipsAdj"=[5007, 5015, 29009, 29109, 29119, 29145]}, {"Fips"=29011, "FipsAdj"=[20037, 29011, 29039, 29057, 29097]}, {"Fips"=29013, "FipsAdj"=[20107, 20121, 29013, 29037, 29083, 29185]}, {"Fips"=29015, "FipsAdj"=[29015, 29029, 29083, 29085, 29141, 29159]}, {"Fips"=29017, "FipsAdj"=[29017, 29031, 29123, 29157, 29207]}, {"Fips"=29019, "FipsAdj"=[29007, 29019, 29027, 29051, 29053, 29089, 29135]}, {"Fips"=29021, "FipsAdj"=[20005, 20043, 29003, 29021, 29049, 29063]}, {"Fips"=29023, "FipsAdj"=[5021, 29023, 29035, 29069, 29181, 29207]}, {"Fips"=29025, "FipsAdj"=[29025, 29033, 29049, 29061, 29063, 29117]}, {"Fips"=29027, "FipsAdj"=[29007, 29019, 29027, 29051, 29139]}, {"Fips"=29029, "FipsAdj"=[29015, 29029, 29059, 29085, 29105, 29131, 29141]}, {"Fips"=29031, "FipsAdj"=[17003, 17181, 29017, 29031, 29157, 29201]}, {"Fips"=29033, "FipsAdj"=[29025, 29033, 29041, 29107, 29117, 29177]}, {"Fips"=29035, "FipsAdj"=[29023, 29035, 29149, 29179, 29181, 29203]}, {"Fips"=29037, "FipsAdj"=[20091, 20121, 29013, 29037, 29083, 29095]}, {"Fips"=29039, "FipsAdj"=[29011, 29039, 29057, 29167, 29185]}, {"Fips"=29041, "FipsAdj"=[29033, 29041, 29089, 29115, 29117, 29121, 29175]}, {"Fips"=29043, "FipsAdj"=[29043, 29067, 29077, 29109, 29209, 29213]}, {"Fips"=29045, "FipsAdj"=[17067, 19111, 19177, 29045, 29103, 29111]}, {"Fips"=29047, "FipsAdj"=[20209, 29047, 29049, 29095, 29165]}, {"Fips"=29049, "FipsAdj"=[29021, 29025, 29047, 29049, 29063, 29165]}, {"Fips"=29051, "FipsAdj"=[29019, 29027, 29051, 29131, 29135]}, {"Fips"=29053, "FipsAdj"=[29019, 29053, 29089, 29135, 29141, 29159]}, {"Fips"=29055, "FipsAdj"=[29055, 29065, 29071, 29073, 29093, 29161]}, {"Fips"=29057, "FipsAdj"=[29011, 29039, 29057, 29077, 29097, 29109]}, {"Fips"=29059, "FipsAdj"=[29029, 29059, 29077, 29085, 29105, 29167]}, {"Fips"=29061, "FipsAdj"=[29025, 29061, 29063, 29075, 29079, 29081]}, {"Fips"=29063, "FipsAdj"=[29003, 29021, 29025, 29049, 29061, 29063]}, {"Fips"=29065, "FipsAdj"=[29055, 29065, 29093, 29161, 29179, 29203]}, {"Fips"=29067, "FipsAdj"=[29043, 29067, 29091, 29153, 29213, 29215, 29225]}, {"Fips"=29069, "FipsAdj"=[5021, 5031, 5055, 5093, 29023, 29069, 29143, 29155]}, {"Fips"=29071, "FipsAdj"=[29055, 29071, 29073, 29099, 29183, 29189, 29219]}, {"Fips"=29073, "FipsAdj"=[29055, 29071, 29073, 29125, 29139, 29151, 29161]}, {"Fips"=29075, "FipsAdj"=[29003, 29061, 29063, 29075, 29081, 29147]}, {"Fips"=29077, "FipsAdj"=[29043, 29057, 29059, 29077, 29109, 29167]}, {"Fips"=29079, "FipsAdj"=[29061, 29079, 29081, 29115, 29117, 29129]}, {"Fips"=29081, "FipsAdj"=[19053, 19159, 29061, 29075, 29079, 29081, 29129]}, {"Fips"=29083, "FipsAdj"=[29013, 29015, 29037, 29083, 29101, 29159]}, {"Fips"=29085, "FipsAdj"=[29015, 29029, 29059, 29085, 29167]}, {"Fips"=29087, "FipsAdj"=[20043, 29003, 29005, 29087, 29147, 31127]}, {"Fips"=29089, "FipsAdj"=[29019, 29041, 29053, 29089, 29175]}, {"Fips"=29091, "FipsAdj"=[5049, 29067, 29091, 29149, 29153, 29203]}, {"Fips"=29093, "FipsAdj"=[29055, 29065, 29093, 29123, 29179, 29187, 29221]}, {"Fips"=29095, "FipsAdj"=[20091, 20209, 29037, 29047, 29095, 29101, 29107]}, {"Fips"=29097, "FipsAdj"=[20021, 20037, 29011, 29057, 29097, 29109]}, {"Fips"=29099, "FipsAdj"=[17133, 29071, 29099, 29186, 29187, 29189]}, {"Fips"=29101, "FipsAdj"=[29037, 29083, 29095, 29101, 29107]}, {"Fips"=29103, "FipsAdj"=[29001, 29045, 29103, 29111, 29121, 29199]}, {"Fips"=29105, "FipsAdj"=[29029, 29059, 29105, 29169, 29215, 29225]}, {"Fips"=29107, "FipsAdj"=[29033, 29095, 29101, 29107, 29159, 29177]}, {"Fips"=29109, "FipsAdj"=[29009, 29043, 29057, 29077, 29097, 29109, 29145]}, {"Fips"=29111, "FipsAdj"=[17001, 17067, 29045, 29103, 29111, 29127]}, {"Fips"=29113, "FipsAdj"=[17013, 29113, 29139, 29163, 29183]}, {"Fips"=29115, "FipsAdj"=[29001, 29041, 29079, 29115, 29117, 29121]}, {"Fips"=29117, "FipsAdj"=[29025, 29033, 29041, 29061, 29079, 29115]}, {"Fips"=29119, "FipsAdj"=[5007, 29009, 29119, 29145, 40041]}, {"Fips"=29121, "FipsAdj"=[29001, 29041, 29103, 29115, 29121, 29137, 29175]}, {"Fips"=29123, "FipsAdj"=[29017, 29093, 29123, 29157, 29187]}, {"Fips"=29125, "FipsAdj"=[29073, 29125, 29131, 29151, 29161]}, {"Fips"=29127, "FipsAdj"=[17001, 17149, 29111, 29127, 29137, 29173]}, {"Fips"=29129, "FipsAdj"=[19053, 19185, 29079, 29081, 29129, 29171]}, {"Fips"=29131, "FipsAdj"=[29029, 29051, 29125, 29131, 29135, 29141, 29151]}, {"Fips"=29133, "FipsAdj"=[17003, 21007, 21039, 21075, 21105, 29133, 29143]}, {"Fips"=29135, "FipsAdj"=[29019, 29051, 29053, 29131, 29135]}, {"Fips"=29137, "FipsAdj"=[29007, 29121, 29127, 29137, 29173, 29175]}, {"Fips"=29139, "FipsAdj"=[29007, 29027, 29073, 29113, 29139, 29151, 29163]}, {"Fips"=29141, "FipsAdj"=[29015, 29029, 29053, 29131, 29135, 29141]}, {"Fips"=29143, "FipsAdj"=[21075, 29069, 29133, 29143, 29155, 29201, 29207]}, {"Fips"=29145, "FipsAdj"=[20021, 29009, 29097, 29109, 29119, 29145]}, {"Fips"=29147, "FipsAdj"=[19145, 19173, 29003, 29005, 29075, 29087, 29147]}, {"Fips"=29149, "FipsAdj"=[5049, 5121, 5135, 29035, 29091, 29149, 29181]}, {"Fips"=29151, "FipsAdj"=[29027, 29051, 29073, 29125, 29131, 29139]}, {"Fips"=29153, "FipsAdj"=[5005, 5049, 5089, 29067, 29091, 29153]}, {"Fips"=29155, "FipsAdj"=[5093, 29069, 29143, 29155, 47045]}, {"Fips"=29157, "FipsAdj"=[17077, 17157, 17181, 29017, 29031, 29123, 29157, 29186]}, {"Fips"=29159, "FipsAdj"=[29015, 29053, 29083, 29101, 29107, 29141, 29159]}, {"Fips"=29161, "FipsAdj"=[29055, 29065, 29073, 29125, 29161, 29169]}, {"Fips"=29163, "FipsAdj"=[17013, 17149, 29007, 29113, 29139, 29163]}, {"Fips"=29165, "FipsAdj"=[20005, 20103, 20209, 29021, 29047, 29049]}, {"Fips"=29167, "FipsAdj"=[29039, 29057, 29059, 29077, 29085, 29167]}, {"Fips"=29169, "FipsAdj"=[29029, 29105, 29125, 29131, 29161, 29169]}, {"Fips"=29171, "FipsAdj"=[19007, 19185, 29001, 29129, 29171, 29197]}, {"Fips"=29173, "FipsAdj"=[17149, 29007, 29127, 29137, 29163]}, {"Fips"=29175, "FipsAdj"=[29007, 29019, 29041, 29089, 29121, 29137]}, {"Fips"=29177, "FipsAdj"=[29025, 29033, 29047, 29049, 29095, 29107]}, {"Fips"=29179, "FipsAdj"=[29035, 29065, 29093, 29179, 29203]}, {"Fips"=29181, "FipsAdj"=[5021, 5121, 29023, 29035, 29149]}, {"Fips"=29183, "FipsAdj"=[17013, 17083, 17119, 29071, 29113, 29183, 29189]}, {"Fips"=29185, "FipsAdj"=[29013, 29015, 29039, 29083, 29085, 29167, 29185]}, {"Fips"=29186, "FipsAdj"=[17133, 17157, 29099, 29157, 29186]}, {"Fips"=29187, "FipsAdj"=[29093, 29099, 29123, 29157, 29186, 29187]}, {"Fips"=29189, "FipsAdj"=[17119, 17133, 17163, 29071, 29099, 29183, 29189]}, {"Fips"=29195, "FipsAdj"=[29033, 29041, 29053, 29089, 29107, 29159]}, {"Fips"=29197, "FipsAdj"=[19007, 19051, 29001, 29171, 29197]}, {"Fips"=29199, "FipsAdj"=[19051, 19177, 29001, 29045, 29103, 29197]}, {"Fips"=29201, "FipsAdj"=[17003, 29031, 29133, 29143, 29201]}, {"Fips"=29203, "FipsAdj"=[29035, 29065, 29091, 29149, 29179, 29203]}, {"Fips"=29205, "FipsAdj"=[29103, 29111, 29121, 29127, 29137]}, {"Fips"=29207, "FipsAdj"=[29017, 29023, 29031, 29069, 29143, 29201, 29207]}, {"Fips"=29209, "FipsAdj"=[5015, 29009, 29043, 29109, 29209]}, {"Fips"=29211, "FipsAdj"=[29001, 29079, 29115, 29129, 29171]}, {"Fips"=29213, "FipsAdj"=[5009, 5015, 5089, 29043, 29067, 29153, 29209]}, {"Fips"=29215, "FipsAdj"=[29065, 29067, 29091, 29105, 29161, 29169, 29203, 29215]}, {"Fips"=29217, "FipsAdj"=[20011, 20037, 20107, 29011, 29013, 29039, 29185]}, {"Fips"=29219, "FipsAdj"=[29071, 29073, 29113, 29139, 29183]}, {"Fips"=29221, "FipsAdj"=[29055, 29071, 29093, 29099, 29187]}, {"Fips"=29223, "FipsAdj"=[29017, 29023, 29035, 29093, 29123, 29179, 29207]}, {"Fips"=29225, "FipsAdj"=[29043, 29059, 29067, 29077, 29105, 29225]}, {"Fips"=29227, "FipsAdj"=[19159, 19173, 29075, 29081, 29147]}, {"Fips"=29229, "FipsAdj"=[29067, 29105, 29215, 29225]}, {"Fips"=29510, "FipsAdj"=[17119, 17163, 29189]}, {"Fips"=30001, "FipsAdj"=[16033, 16043, 16059, 30001, 30023, 30057, 30081]}, {"Fips"=30003, "FipsAdj"=[30003, 30009, 30075, 30087, 30103, 30111, 56003]}, {"Fips"=30005, "FipsAdj"=[30005, 30015, 30027, 30041]}, {"Fips"=30007, "FipsAdj"=[30007, 30031, 30043, 30049]}, {"Fips"=30009, "FipsAdj"=[30003, 30009, 30067, 30095, 30111, 56003]}, {"Fips"=30011, "FipsAdj"=[30011, 30017, 30025, 30075, 46019, 46063]}, {"Fips"=30013, "FipsAdj"=[30013, 30015, 30045, 30049, 30059]}, {"Fips"=30015, "FipsAdj"=[30005, 30013, 30015, 30027, 30041, 30045, 30051, 30073]}, {"Fips"=30017, "FipsAdj"=[30011, 30017, 30025, 30033, 30075, 30079]}, {"Fips"=30019, "FipsAdj"=[30019, 30085, 30091]}, {"Fips"=30021, "FipsAdj"=[30021, 30055, 30079, 30083]}, {"Fips"=30023, "FipsAdj"=[30001, 30023, 30039, 30043, 30077, 30081]}, {"Fips"=30025, "FipsAdj"=[30011, 30017, 30025, 30079, 30109, 38011, 38033, 38087]}, {"Fips"=30027, "FipsAdj"=[30005, 30015, 30027, 30037, 30045, 30065, 30069, 30071]}, {"Fips"=30029, "FipsAdj"=[30029, 30035, 30047, 30049, 30053, 30063, 30073, 30077, 30089]}, {"Fips"=30031, "FipsAdj"=[16043, 30007, 30031, 30043, 30057, 30059, 30067, 56029]}, {"Fips"=30033, "FipsAdj"=[30017, 30033, 30055, 30069, 30071, 30079, 30087]}, {"Fips"=30035, "FipsAdj"=[30029, 30035, 30073]}, {"Fips"=30037, "FipsAdj"=[30027, 30037, 30065, 30095, 30097, 30107]}, {"Fips"=30039, "FipsAdj"=[30023, 30039, 30063, 30077]}, {"Fips"=30041, "FipsAdj"=[30005, 30015, 30041]}, {"Fips"=30043, "FipsAdj"=[30007, 30023, 30031, 30043, 30049, 30057, 30077]}, {"Fips"=30045, "FipsAdj"=[30013, 30015, 30027, 30045, 30059]}, {"Fips"=30047, "FipsAdj"=[30029, 30047, 30063]}, {"Fips"=30049, "FipsAdj"=[30007, 30013, 30029, 30043, 30049, 30059, 30077]}, {"Fips"=30051, "FipsAdj"=[30015, 30041, 30051, 30073]}, {"Fips"=30053, "FipsAdj"=[16017, 16021, 30029, 30053]}, {"Fips"=30055, "FipsAdj"=[30021, 30033, 30055, 30079, 30083, 30085]}, {"Fips"=30057, "FipsAdj"=[16043, 30001, 30031, 30043, 30057]}, {"Fips"=30059, "FipsAdj"=[30007, 30013, 30031, 30045, 30049, 30059, 30067, 30097]}, {"Fips"=30061, "FipsAdj"=[16035, 16079, 30061, 30063]}, {"Fips"=30063, "FipsAdj"=[16035, 16049, 30029, 30039, 30047, 30061, 30063, 30077, 30081]}, {"Fips"=30065, "FipsAdj"=[30027, 30037, 30065, 30069, 30087]}, {"Fips"=30067, "FipsAdj"=[30009, 30031, 30059, 30067, 30095, 30097]}, {"Fips"=30069, "FipsAdj"=[30027, 30033, 30065, 30069, 30071]}, {"Fips"=30071, "FipsAdj"=[30005, 30027, 30033, 30069, 30071]}, {"Fips"=30073, "FipsAdj"=[30015, 30029, 30035, 30051, 30073, 30099]}, {"Fips"=30075, "FipsAdj"=[30003, 30011, 30017, 30075, 30087, 56005, 56011]}, {"Fips"=30077, "FipsAdj"=[30023, 30029, 30039, 30043, 30049, 30063]}, {"Fips"=30079, "FipsAdj"=[30017, 30021, 30025, 30033, 30055, 30079]}, {"Fips"=30081, "FipsAdj"=[16049, 16059, 30001, 30023, 30039, 30063]}, {"Fips"=30083, "FipsAdj"=[30021, 30055, 30083, 30085, 30109, 38053]}, {"Fips"=30085, "FipsAdj"=[30019, 30055, 30083, 30085, 30091, 30105, 38053]}, {"Fips"=30087, "FipsAdj"=[30003, 30017, 30033, 30065, 30069, 30075, 30087, 30103]}, {"Fips"=30089, "FipsAdj"=[16017, 16079, 30029, 30047, 30053, 30061, 30063]}, {"Fips"=30091, "FipsAdj"=[30019, 30085, 30091, 38023]}, {"Fips"=30093, "FipsAdj"=[30001, 30023, 30043, 30057]}, {"Fips"=30095, "FipsAdj"=[30009, 30037, 30067, 30095, 30097]}, {"Fips"=30097, "FipsAdj"=[30037, 30059, 30067, 30095, 30097]}, {"Fips"=30099, "FipsAdj"=[30013, 30015, 30029, 30049, 30073]}, {"Fips"=30101, "FipsAdj"=[30035, 30051, 30073]}, {"Fips"=30103, "FipsAdj"=[30003, 30087, 30103]}, {"Fips"=30105, "FipsAdj"=[30019, 30033, 30055, 30071, 30085]}, {"Fips"=30107, "FipsAdj"=[30027, 30037, 30045, 30059, 30097]}, {"Fips"=30109, "FipsAdj"=[30021, 30025, 30079, 30083, 30109, 38033]}, {"Fips"=30111, "FipsAdj"=[30003, 30009, 30037, 30065, 30087, 30095, 30103]}, {"Fips"=31001, "FipsAdj"=[31001, 31019, 31035, 31079, 31081, 31099]}, {"Fips"=31003, "FipsAdj"=[31003, 31011, 31089, 31107, 31119, 31139]}, {"Fips"=31005, "FipsAdj"=[31005, 31069, 31075, 31091, 31101]}, {"Fips"=31007, "FipsAdj"=[31007, 31033, 31105, 31123, 31157, 56015]}, {"Fips"=31009, "FipsAdj"=[31009, 31017, 31031, 31041, 31113, 31115]}, {"Fips"=31011, "FipsAdj"=[31003, 31011, 31077, 31119, 31125, 31141]}, {"Fips"=31013, "FipsAdj"=[31013, 31045, 31123, 31157, 31161]}, {"Fips"=31015, "FipsAdj"=[31015, 31089, 31103, 31107, 31149, 46023]}, {"Fips"=31017, "FipsAdj"=[31009, 31017, 31031, 31103, 31115]}, {"Fips"=31019, "FipsAdj"=[31001, 31019, 31041, 31047, 31079, 31093, 31099, 31137]}, {"Fips"=31021, "FipsAdj"=[19085, 19133, 31021, 31039, 31053, 31173]}, {"Fips"=31023, "FipsAdj"=[31023, 31037, 31053, 31109, 31141, 31143, 31155, 31159]}, {"Fips"=31025, "FipsAdj"=[19071, 19129, 31025, 31109, 31131, 31153]}, {"Fips"=31027, "FipsAdj"=[31027, 31051, 31107, 31139, 31179, 46027]}, {"Fips"=31029, "FipsAdj"=[8095, 8125, 31029, 31057, 31085]}, {"Fips"=31031, "FipsAdj"=[31009, 31017, 31031, 31075, 31091, 31103, 31161, 31171, 46007, 46113, 46121]}, {"Fips"=31033, "FipsAdj"=[8075, 8115, 31007, 31033, 31049, 31069, 31105]}, {"Fips"=31035, "FipsAdj"=[31001, 31035, 31059, 31081, 31129, 31181]}, {"Fips"=31037, "FipsAdj"=[31023, 31037, 31039, 31053, 31141]}, {"Fips"=31039, "FipsAdj"=[31021, 31037, 31039, 31053, 31167, 31173]}, {"Fips"=31041, "FipsAdj"=[31009, 31019, 31041, 31047, 31071, 31111, 31113, 31115, 31163]}, {"Fips"=31043, "FipsAdj"=[19193, 31043, 31051, 31173]}, {"Fips"=31045, "FipsAdj"=[31013, 31045, 31161, 31165, 46047]}, {"Fips"=31047, "FipsAdj"=[31019, 31041, 31047, 31063, 31073, 31111]}, {"Fips"=31049, "FipsAdj"=[8115, 31033, 31049, 31069, 31101]}, {"Fips"=31051, "FipsAdj"=[31027, 31043, 31051, 31173, 31179, 46027]}, {"Fips"=31053, "FipsAdj"=[31021, 31023, 31037, 31039, 31053, 31055, 31155]}, {"Fips"=31055, "FipsAdj"=[19155, 31053, 31055, 31153, 31155]}, {"Fips"=31057, "FipsAdj"=[8125, 20023, 20153, 31029, 31057, 31085]}, {"Fips"=31059, "FipsAdj"=[31035, 31059, 31095, 31129, 31151, 31159, 31169]}, {"Fips"=31061, "FipsAdj"=[20147, 20183, 31061, 31083, 31099, 31137]}, {"Fips"=31063, "FipsAdj"=[31047, 31063, 31065, 31073, 31085, 31087, 31111]}, {"Fips"=31065, "FipsAdj"=[20039, 20137, 31063, 31065, 31073, 31083, 31137]}, {"Fips"=31067, "FipsAdj"=[20117, 20201, 31067, 31095, 31097, 31109, 31131, 31133]}, {"Fips"=31069, "FipsAdj"=[31005, 31033, 31049, 31069, 31075, 31101, 31123]}, {"Fips"=31071, "FipsAdj"=[31041, 31071, 31089, 31115, 31175]}, {"Fips"=31073, "FipsAdj"=[31047, 31063, 31065, 31073]}, {"Fips"=31075, "FipsAdj"=[31005, 31031, 31069, 31075, 31091]}, {"Fips"=31077, "FipsAdj"=[31011, 31077, 31093, 31125, 31163, 31175]}, {"Fips"=31079, "FipsAdj"=[31001, 31019, 31079, 31081, 31093]}, {"Fips"=31081, "FipsAdj"=[31001, 31035, 31079, 31081, 31121, 31143]}, {"Fips"=31083, "FipsAdj"=[20137, 20147, 31061, 31065, 31083, 31099]}, {"Fips"=31085, "FipsAdj"=[31029, 31057, 31063, 31085, 31087, 31111]}, {"Fips"=31087, "FipsAdj"=[20153, 31057, 31063, 31085, 31087]}, {"Fips"=31089, "FipsAdj"=[31003, 31015, 31071, 31089, 31103, 31107, 31115, 31149]}, {"Fips"=31091, "FipsAdj"=[31005, 31031, 31075, 31091, 31117]}, {"Fips"=31093, "FipsAdj"=[31019, 31077, 31079, 31093, 31121, 31125]}, {"Fips"=31095, "FipsAdj"=[20157, 20201, 31059, 31067, 31095, 31151]}, {"Fips"=31097, "FipsAdj"=[31067, 31097, 31109, 31127, 31131]}, {"Fips"=31099, "FipsAdj"=[31001, 31019, 31061, 31083, 31099, 31137]}, {"Fips"=31101, "FipsAdj"=[31005, 31049, 31069, 31101, 31111, 31117]}, {"Fips"=31103, "FipsAdj"=[31015, 31017, 31031, 31089, 31103, 31149, 46053, 46121]}, {"Fips"=31105, "FipsAdj"=[8075, 8123, 31007, 31033, 31105]}, {"Fips"=31107, "FipsAdj"=[31003, 31015, 31027, 31089, 31107, 31139, 46009, 46023]}, {"Fips"=31109, "FipsAdj"=[31023, 31025, 31067, 31097, 31109, 31131, 31151, 31155]}, {"Fips"=31111, "FipsAdj"=[31041, 31047, 31063, 31085, 31101, 31111, 31113, 31117]}, {"Fips"=31113, "FipsAdj"=[31009, 31041, 31111, 31113, 31117]}, {"Fips"=31115, "FipsAdj"=[31009, 31017, 31041, 31071, 31089, 31115]}, {"Fips"=31117, "FipsAdj"=[31005, 31091, 31101, 31111, 31113, 31117]}, {"Fips"=31119, "FipsAdj"=[31003, 31011, 31119, 31139, 31141, 31167]}, {"Fips"=31121, "FipsAdj"=[31079, 31081, 31093, 31121, 31125, 31141]}, {"Fips"=31123, "FipsAdj"=[31007, 31013, 31033, 31069, 31123, 31157]}, {"Fips"=31125, "FipsAdj"=[31011, 31077, 31093, 31121, 31125]}, {"Fips"=31127, "FipsAdj"=[29005, 29087, 31097, 31127, 31131, 31133]}, {"Fips"=31129, "FipsAdj"=[20089, 20157, 31035, 31059, 31129, 31169]}, {"Fips"=31131, "FipsAdj"=[19071, 29005, 31025, 31067, 31097, 31109, 31127]}, {"Fips"=31133, "FipsAdj"=[20117, 20131, 31067, 31097, 31127, 31133]}, {"Fips"=31135, "FipsAdj"=[8095, 8115, 31029, 31049, 31085, 31101, 31111]}, {"Fips"=31137, "FipsAdj"=[31019, 31047, 31061, 31065, 31073, 31083, 31099]}, {"Fips"=31139, "FipsAdj"=[31003, 31027, 31107, 31119, 31139, 31167]}, {"Fips"=31141, "FipsAdj"=[31011, 31023, 31037, 31119, 31121, 31125, 31141, 31143]}, {"Fips"=31143, "FipsAdj"=[31023, 31081, 31121, 31141, 31143, 31159]}, {"Fips"=31145, "FipsAdj"=[20039, 20153, 31063, 31065, 31087]}, {"Fips"=31147, "FipsAdj"=[20013, 20043, 20131, 29087, 31127, 31133]}, {"Fips"=31149, "FipsAdj"=[31015, 31017, 31089, 31103, 31115]}, {"Fips"=31151, "FipsAdj"=[31059, 31067, 31095, 31109, 31151, 31159, 31169]}, {"Fips"=31153, "FipsAdj"=[19129, 19155, 31025, 31055, 31153]}, {"Fips"=31155, "FipsAdj"=[31023, 31025, 31053, 31055, 31109, 31153]}, {"Fips"=31157, "FipsAdj"=[31007, 31013, 31123, 31157, 31165]}, {"Fips"=31159, "FipsAdj"=[31023, 31059, 31109, 31143, 31151, 31159]}, {"Fips"=31161, "FipsAdj"=[31013, 31031, 31045, 31069, 31075, 31123, 31161]}, {"Fips"=31163, "FipsAdj"=[31019, 31041, 31077, 31093, 31163]}, {"Fips"=31165, "FipsAdj"=[31013, 31045, 31157, 31165, 46047, 56015]}, {"Fips"=31167, "FipsAdj"=[31037, 31039, 31119, 31139, 31141, 31167]}, {"Fips"=31169, "FipsAdj"=[20157, 20201, 31059, 31095, 31129, 31151]}, {"Fips"=31171, "FipsAdj"=[31009, 31031, 31091, 31113, 31117]}, {"Fips"=31173, "FipsAdj"=[19133, 19193, 31021, 31039, 31043, 31051, 31173]}, {"Fips"=31175, "FipsAdj"=[31041, 31071, 31077, 31163, 31175]}, {"Fips"=31177, "FipsAdj"=[19085, 19155, 31021, 31053, 31055]}, {"Fips"=31179, "FipsAdj"=[31027, 31039, 31051, 31119, 31139, 31167, 31173]}, {"Fips"=31181, "FipsAdj"=[20089, 20183, 31001, 31035, 31061, 31099, 31129]}, {"Fips"=31183, "FipsAdj"=[31003, 31011, 31071, 31077, 31089, 31175]}, {"Fips"=31185, "FipsAdj"=[31023, 31035, 31059, 31081, 31143, 31151, 31159]}, {"Fips"=32001, "FipsAdj"=[32001, 32015, 32019, 32021, 32023, 32027]}, {"Fips"=32003, "FipsAdj"=[4015, 6027, 6071, 32003, 32017]}, {"Fips"=32005, "FipsAdj"=[6003, 6017, 6051, 6061, 32005, 32019]}, {"Fips"=32007, "FipsAdj"=[16031, 16073, 16083, 32007, 32011, 32013, 32015, 32033, 49003]}, {"Fips"=32009, "FipsAdj"=[6027, 6051, 32009, 32021]}, {"Fips"=32011, "FipsAdj"=[32007, 32011, 32015, 32023]}, {"Fips"=32013, "FipsAdj"=[16073, 32007, 32013, 32015, 32027, 32031, 41025]}, {"Fips"=32015, "FipsAdj"=[32001, 32007, 32011, 32013, 32015, 32023]}, {"Fips"=32017, "FipsAdj"=[4015, 32003, 32017, 32023, 32033, 49001, 49021, 49027]}, {"Fips"=32019, "FipsAdj"=[6051, 32001, 32005, 32019, 32021, 32029, 32031]}, {"Fips"=32021, "FipsAdj"=[6051, 32001, 32009, 32019, 32021]}, {"Fips"=32023, "FipsAdj"=[6027, 32001, 32003, 32009, 32011, 32015, 32017, 32021, 32023]}, {"Fips"=32027, "FipsAdj"=[32001, 32013, 32015, 32027]}, {"Fips"=32029, "FipsAdj"=[32019, 32029, 32031]}, {"Fips"=32031, "FipsAdj"=[6035, 6049, 6057, 6061, 6091, 32001, 32013, 32019, 32027, 32029, 32031, 32510, 41025]}, {"Fips"=32033, "FipsAdj"=[32007, 32011, 32017, 32023, 32033, 49023, 49027]}, {"Fips"=32510, "FipsAdj"=[6061, 32005, 32019, 32029, 32031]}, {"Fips"=33001, "FipsAdj"=[33001, 33003, 33009, 33013]}, {"Fips"=33003, "FipsAdj"=[23017, 23031, 33001, 33003, 33007, 33009]}, {"Fips"=33005, "FipsAdj"=[25011, 25027, 33005, 33011, 33019]}, {"Fips"=33007, "FipsAdj"=[23017, 33003, 33007, 33009]}, {"Fips"=33009, "FipsAdj"=[33001, 33003, 33007, 33009, 33013, 33019, 50005, 50009, 50017]}, {"Fips"=33011, "FipsAdj"=[25009, 25017, 25027, 33005, 33011, 33013, 33015]}, {"Fips"=33013, "FipsAdj"=[33001, 33009, 33011, 33013, 33015, 33017]}, {"Fips"=33015, "FipsAdj"=[23031, 25009, 33011, 33013, 33015]}, {"Fips"=33017, "FipsAdj"=[23031, 33001, 33003, 33013, 33015]}, {"Fips"=33019, "FipsAdj"=[33005, 33009, 33011, 33013, 33019, 50025]}, {"Fips"=34001, "FipsAdj"=[34001, 34005, 34007, 34009, 34011, 34015]}, {"Fips"=34003, "FipsAdj"=[34003, 34013, 34017, 34031, 36005, 36061, 36087]}, {"Fips"=34005, "FipsAdj"=[34001, 34005, 34007, 34021, 34025, 34029, 42017]}, {"Fips"=34007, "FipsAdj"=[34001, 34005, 34007, 34015]}, {"Fips"=34009, "FipsAdj"=[10001, 10005, 34001, 34009]}, {"Fips"=34011, "FipsAdj"=[10001, 34001, 34009, 34011, 34015]}, {"Fips"=34013, "FipsAdj"=[34003, 34013, 34017, 34027, 34031]}, {"Fips"=34015, "FipsAdj"=[10003, 34001, 34007, 34011, 34015, 34033, 42045]}, {"Fips"=34017, "FipsAdj"=[34003, 34013, 34017, 34039, 36047, 36061]}, {"Fips"=34019, "FipsAdj"=[34019, 34021, 34027, 34035, 34041]}, {"Fips"=34021, "FipsAdj"=[34005, 34019, 34021, 34023, 34025, 34035]}, {"Fips"=34023, "FipsAdj"=[34021, 34023, 34025, 34035, 34039]}, {"Fips"=34025, "FipsAdj"=[34005, 34021, 34023, 34025, 34029, 36081]}, {"Fips"=34027, "FipsAdj"=[34013, 34019, 34027, 34031, 34035, 34037, 34039]}, {"Fips"=34029, "FipsAdj"=[34001, 34005, 34025]}, {"Fips"=34031, "FipsAdj"=[34003, 34013, 34027, 34031, 34037, 36071]}, {"Fips"=34033, "FipsAdj"=[10001, 10003, 34011, 34015]}, {"Fips"=34035, "FipsAdj"=[34019, 34021, 34023, 34027, 34035]}, {"Fips"=34037, "FipsAdj"=[34027, 34031, 34037, 34041, 36071, 42089]}, {"Fips"=34039, "FipsAdj"=[34013, 34017, 34023, 34027, 34035, 34039]}, {"Fips"=34041, "FipsAdj"=[34019, 34027, 34037, 34041, 42017, 42089]}, {"Fips"=35001, "FipsAdj"=[35001, 35006, 35043, 35049, 35057]}, {"Fips"=35003, "FipsAdj"=[4001, 4011, 35003, 35006, 35017, 35051]}, {"Fips"=35005, "FipsAdj"=[35005, 35011, 35015, 35025, 35027, 35035]}, {"Fips"=35006, "FipsAdj"=[4001, 35001, 35003, 35006, 35031, 35043, 35053]}, {"Fips"=35007, "FipsAdj"=[8023, 8071, 35007, 35021, 35033, 35055]}, {"Fips"=35009, "FipsAdj"=[35009, 35037, 35041, 48017, 48117]}, {"Fips"=35011, "FipsAdj"=[35005, 35011, 35019, 35027, 35037]}, {"Fips"=35013, "FipsAdj"=[35013, 35029, 35035, 35051]}, {"Fips"=35015, "FipsAdj"=[35005, 35015, 35025, 35035, 48109, 48301]}, {"Fips"=35017, "FipsAdj"=[4011, 35003, 35017, 35023, 35029]}, {"Fips"=35019, "FipsAdj"=[35011, 35019, 35027, 35037, 35047]}, {"Fips"=35021, "FipsAdj"=[35007, 35021, 35033, 35037, 35047]}, {"Fips"=35023, "FipsAdj"=[4003, 4011, 35017, 35023]}, {"Fips"=35025, "FipsAdj"=[35005, 35015, 35025, 35041, 48003, 48079, 48165, 48301, 48495]}, {"Fips"=35027, "FipsAdj"=[35005, 35011, 35019, 35027, 35035, 35051, 35053]}, {"Fips"=35028, "FipsAdj"=[35028, 35039, 35043]}, {"Fips"=35029, "FipsAdj"=[35013, 35017, 35023, 35029]}, {"Fips"=35031, "FipsAdj"=[4001, 35006, 35031, 35043]}, {"Fips"=35033, "FipsAdj"=[35007, 35021, 35033, 35039, 35047, 35049]}, {"Fips"=35035, "FipsAdj"=[35005, 35013, 35015, 35027, 35035, 35051, 48109, 48141]}, {"Fips"=35037, "FipsAdj"=[35009, 35011, 35019, 35021, 35037, 35041, 35047, 35059, 48117, 48205]}, {"Fips"=35039, "FipsAdj"=[8007, 8021, 35028, 35033, 35039, 35043, 35045, 35049]}, {"Fips"=35041, "FipsAdj"=[35005, 35009, 35011, 35025, 35037, 35041, 48017]}, {"Fips"=35043, "FipsAdj"=[35001, 35006, 35028, 35031, 35039, 35043, 35045]}, {"Fips"=35045, "FipsAdj"=[4001, 8007, 8067, 8083, 35031, 35039, 35043, 35045]}, {"Fips"=35047, "FipsAdj"=[35019, 35021, 35033, 35037, 35047, 35049]}, {"Fips"=35049, "FipsAdj"=[35001, 35028, 35033, 35039, 35043, 35047, 35049]}, {"Fips"=35051, "FipsAdj"=[35003, 35013, 35017, 35027, 35029, 35035, 35051]}, {"Fips"=35053, "FipsAdj"=[35003, 35006, 35027, 35051, 35053, 35057]}, {"Fips"=35055, "FipsAdj"=[8021, 8023, 35007, 35033, 35039]}, {"Fips"=35057, "FipsAdj"=[35001, 35019, 35027, 35047, 35049, 35053, 35057]}, {"Fips"=35059, "FipsAdj"=[8009, 8071, 35007, 35021, 35037, 35059, 40025, 48111]}, {"Fips"=35061, "FipsAdj"=[35001, 35006, 35053, 35057]}, {"Fips"=36001, "FipsAdj"=[36001, 36021, 36039, 36083, 36091, 36093]}, {"Fips"=36003, "FipsAdj"=[36003, 36009, 36051, 36101, 36121, 42083]}, {"Fips"=36005, "FipsAdj"=[34003, 36005, 36059, 36061, 36081]}, {"Fips"=36007, "FipsAdj"=[36007, 36017, 36023, 36025, 36107, 42115]}, {"Fips"=36009, "FipsAdj"=[36003, 36009, 36013, 36029, 36121, 42083]}, {"Fips"=36011, "FipsAdj"=[36011, 36023, 36045, 36067, 36075, 36099, 36109]}, {"Fips"=36013, "FipsAdj"=[36009, 36013, 36029, 42049]}, {"Fips"=36015, "FipsAdj"=[36015, 36097, 36101, 36107, 36109, 42015]}, {"Fips"=36017, "FipsAdj"=[36007, 36017, 36023, 36025, 36053]}, {"Fips"=36019, "FipsAdj"=[36019, 36031, 36033, 50007]}, {"Fips"=36021, "FipsAdj"=[25003, 36001, 36021, 36027, 36039, 36083]}, {"Fips"=36023, "FipsAdj"=[36007, 36011, 36017, 36023, 36053, 36067, 36107]}, {"Fips"=36025, "FipsAdj"=[36007, 36017, 36025, 36039, 36077, 36095, 36105, 36111]}, {"Fips"=36027, "FipsAdj"=[9001, 9005, 25003, 36021, 36027, 36071, 36079]}, {"Fips"=36029, "FipsAdj"=[36009, 36013, 36029, 36037, 36063]}, {"Fips"=36031, "FipsAdj"=[36019, 36031, 36033, 36041, 36113, 36115, 50001]}, {"Fips"=36033, "FipsAdj"=[36019, 36031, 36033, 36041]}, {"Fips"=36035, "FipsAdj"=[36035, 36041, 36043, 36057]}, {"Fips"=36037, "FipsAdj"=[36029, 36037, 36051, 36055, 36063, 36073]}, {"Fips"=36039, "FipsAdj"=[36001, 36021, 36025, 36039, 36083, 36095]}, {"Fips"=36041, "FipsAdj"=[36031, 36033, 36035, 36041, 36043, 36089, 36091]}, {"Fips"=36043, "FipsAdj"=[36035, 36041, 36043, 36049, 36057, 36065, 36077]}, {"Fips"=36045, "FipsAdj"=[36011, 36045, 36049, 36075]}, {"Fips"=36047, "FipsAdj"=[34017, 36047, 36061, 36081]}, {"Fips"=36049, "FipsAdj"=[36043, 36045, 36049, 36065, 36075]}, {"Fips"=36051, "FipsAdj"=[36003, 36037, 36051, 36055, 36069, 36101]}, {"Fips"=36053, "FipsAdj"=[36017, 36023, 36053, 36065, 36067, 36075]}, {"Fips"=36055, "FipsAdj"=[36037, 36051, 36055, 36069, 36073]}, {"Fips"=36057, "FipsAdj"=[36035, 36043, 36057, 36077, 36091, 36093]}, {"Fips"=36059, "FipsAdj"=[9001, 36005, 36059, 36081, 36103]}, {"Fips"=36061, "FipsAdj"=[34003, 34017, 36005, 36047, 36061]}, {"Fips"=36063, "FipsAdj"=[36029, 36037, 36063]}, {"Fips"=36065, "FipsAdj"=[36043, 36049, 36053, 36065, 36075]}, {"Fips"=36067, "FipsAdj"=[36011, 36023, 36053, 36067]}, {"Fips"=36069, "FipsAdj"=[36051, 36055, 36069, 36099, 36101, 36117]}, {"Fips"=36071, "FipsAdj"=[34031, 34037, 36027, 36071, 36079, 36087, 36105, 36111]}, {"Fips"=36073, "FipsAdj"=[36037, 36055, 36063]}, {"Fips"=36075, "FipsAdj"=[36011, 36045, 36049, 36053, 36065, 36067]}, {"Fips"=36077, "FipsAdj"=[36017, 36025, 36043, 36053, 36057, 36065, 36077]}, {"Fips"=36079, "FipsAdj"=[9001, 36027, 36071, 36079, 36087]}, {"Fips"=36081, "FipsAdj"=[34025, 36005, 36047, 36059, 36061, 36081]}, {"Fips"=36083, "FipsAdj"=[25003, 36001, 36021, 36039, 36083, 36091, 36115]}, {"Fips"=36085, "FipsAdj"=[34017, 34023, 34025, 34039, 36047, 36081]}, {"Fips"=36087, "FipsAdj"=[34003, 34031, 36071, 36079, 36087]}, {"Fips"=36089, "FipsAdj"=[36033, 36041, 36043, 36045, 36049]}, {"Fips"=36091, "FipsAdj"=[36001, 36035, 36041, 36057, 36083, 36091, 36093, 36113]}, {"Fips"=36093, "FipsAdj"=[36001, 36057, 36091, 36093]}, {"Fips"=36095, "FipsAdj"=[36001, 36025, 36039, 36057, 36077, 36093]}, {"Fips"=36097, "FipsAdj"=[36015, 36097, 36099, 36101, 36109]}, {"Fips"=36099, "FipsAdj"=[36011, 36069, 36097, 36099, 36109, 36117]}, {"Fips"=36101, "FipsAdj"=[36003, 36015, 36051, 36069, 36097, 36101, 36123, 42105]}, {"Fips"=36103, "FipsAdj"=[9001, 9007, 9009, 9011, 36059, 36103]}, {"Fips"=36105, "FipsAdj"=[36025, 36071, 36105, 36111, 42103]}, {"Fips"=36107, "FipsAdj"=[36007, 36015, 36023, 36107, 36109, 42015]}, {"Fips"=36109, "FipsAdj"=[36011, 36015, 36023, 36097, 36099, 36107]}, {"Fips"=36111, "FipsAdj"=[36021, 36025, 36027, 36039, 36071, 36105]}, {"Fips"=36113, "FipsAdj"=[36031, 36041, 36091, 36113]}, {"Fips"=36115, "FipsAdj"=[36031, 36083, 36091, 36113, 36115, 50001, 50003]}, {"Fips"=36117, "FipsAdj"=[36011, 36055, 36069, 36099]}, {"Fips"=36119, "FipsAdj"=[9001, 34003, 36005, 36059, 36079, 36087]}, {"Fips"=36121, "FipsAdj"=[36003, 36009, 36029, 36037, 36051]}, {"Fips"=36123, "FipsAdj"=[36069, 36097, 36099, 36101]}, {"Fips"=37001, "FipsAdj"=[37001, 37033, 37037, 37081, 37135, 37151]}, {"Fips"=37003, "FipsAdj"=[37003, 37027, 37035, 37097]}, {"Fips"=37005, "FipsAdj"=[37005, 37009, 37171, 37193]}, {"Fips"=37007, "FipsAdj"=[37007, 37123, 37153, 37167, 37179, 45025]}, {"Fips"=37009, "FipsAdj"=[37005, 37009, 37189, 37193, 47091]}, {"Fips"=37011, "FipsAdj"=[37011, 37023, 37027, 37111, 37121, 37189, 47019]}, {"Fips"=37013, "FipsAdj"=[37013, 37049, 37095, 37117, 37137, 37147]}, {"Fips"=37015, "FipsAdj"=[37015, 37041, 37083, 37091, 37117, 37131]}, {"Fips"=37017, "FipsAdj"=[37017, 37047, 37051, 37141, 37155]}, {"Fips"=37019, "FipsAdj"=[37019, 37047, 37129, 37141]}, {"Fips"=37021, "FipsAdj"=[37021, 37087, 37089, 37111, 37115, 37161]}, {"Fips"=37023, "FipsAdj"=[37011, 37023, 37027, 37035, 37045, 37109, 37111]}, {"Fips"=37025, "FipsAdj"=[37025, 37097, 37119, 37159, 37167]}, {"Fips"=37027, "FipsAdj"=[37003, 37011, 37023, 37027, 37035, 37189]}, {"Fips"=37029, "FipsAdj"=[37029, 37053, 37073, 37139, 37177, 51550]}, {"Fips"=37031, "FipsAdj"=[37031, 37049, 37095, 37103, 37133]}, {"Fips"=37033, "FipsAdj"=[37001, 37033, 37135, 37145, 37157, 51083, 51143]}, {"Fips"=37035, "FipsAdj"=[37003, 37023, 37027, 37035, 37097]}, {"Fips"=37037, "FipsAdj"=[37001, 37037, 37063, 37085, 37105, 37125, 37135, 37151]}, {"Fips"=37039, "FipsAdj"=[13111, 13291, 37039, 37043, 37075, 37113, 47123]}, {"Fips"=37041, "FipsAdj"=[37015, 37041, 37073, 37091, 37143]}, {"Fips"=37043, "FipsAdj"=[13241, 13281, 13291, 37039, 37043]}, {"Fips"=37045, "FipsAdj"=[37023, 37045, 37071, 37109, 37161, 45021]}, {"Fips"=37047, "FipsAdj"=[37017, 37019, 37047, 37141, 37155, 45033]}, {"Fips"=37049, "FipsAdj"=[37013, 37031, 37049, 37103, 37107, 37137]}, {"Fips"=37051, "FipsAdj"=[37017, 37051, 37085, 37093, 37125, 37155]}, {"Fips"=37053, "FipsAdj"=[37029, 37053, 37055, 37177, 51550]}, {"Fips"=37055, "FipsAdj"=[37053, 37055, 37095]}, {"Fips"=37057, "FipsAdj"=[37057, 37059, 37067, 37081, 37123, 37151, 37159]}, {"Fips"=37059, "FipsAdj"=[37057, 37059, 37067, 37097, 37159]}, {"Fips"=37061, "FipsAdj"=[37061, 37103, 37107, 37133, 37141, 37163]}, {"Fips"=37063, "FipsAdj"=[37037, 37063, 37077, 37135, 37145]}, {"Fips"=37065, "FipsAdj"=[37065, 37083, 37117, 37127, 37147]}, {"Fips"=37067, "FipsAdj"=[37057, 37059, 37067, 37081, 37157, 37169, 37171]}, {"Fips"=37069, "FipsAdj"=[37069, 37077, 37083, 37101, 37127, 37181, 37183]}, {"Fips"=37071, "FipsAdj"=[37045, 37071, 37109, 37119]}, {"Fips"=37073, "FipsAdj"=[37029, 37041, 37073, 37091, 37139, 37143, 51175]}, {"Fips"=37075, "FipsAdj"=[37039, 37075, 37113, 37173, 47009]}, {"Fips"=37077, "FipsAdj"=[37063, 37069, 37077, 37145, 37181, 37183, 51083]}, {"Fips"=37079, "FipsAdj"=[37079, 37107, 37147, 37191]}, {"Fips"=37081, "FipsAdj"=[37001, 37057, 37067, 37081, 37151, 37157]}, {"Fips"=37083, "FipsAdj"=[37015, 37065, 37069, 37083, 37117, 37127, 37131]}, {"Fips"=37085, "FipsAdj"=[37037, 37051, 37085, 37101, 37105, 37125, 37163]}, {"Fips"=37087, "FipsAdj"=[37021, 37087, 37089, 37099, 37115, 37173, 37175, 47029]}, {"Fips"=37089, "FipsAdj"=[37021, 37087, 37089, 37149, 37161, 37175]}, {"Fips"=37091, "FipsAdj"=[37015, 37041, 37073, 37091, 37131]}, {"Fips"=37093, "FipsAdj"=[37051, 37093, 37125, 37153, 37155]}, {"Fips"=37095, "FipsAdj"=[37013, 37031, 37055, 37095, 37137, 37177]}, {"Fips"=37097, "FipsAdj"=[37003, 37025, 37035, 37059, 37097, 37109, 37119, 37159, 37193]}, {"Fips"=37099, "FipsAdj"=[13241, 37087, 37099, 37113, 37173, 37175]}, {"Fips"=37101, "FipsAdj"=[37069, 37085, 37101, 37127, 37163, 37183, 37191]}, {"Fips"=37103, "FipsAdj"=[37031, 37049, 37061, 37103, 37107]}, {"Fips"=37105, "FipsAdj"=[37037, 37085, 37105]}, {"Fips"=37107, "FipsAdj"=[37049, 37061, 37079, 37103, 37107, 37147]}, {"Fips"=37109, "FipsAdj"=[37023, 37035, 37045, 37071, 37097, 37109]}, {"Fips"=37111, "FipsAdj"=[37011, 37021, 37023, 37111, 37121, 37161]}, {"Fips"=37113, "FipsAdj"=[13241, 37039, 37043, 37075, 37099, 37113, 37173]}, {"Fips"=37115, "FipsAdj"=[37021, 37087, 37115, 37199, 47029, 47059]}, {"Fips"=37117, "FipsAdj"=[37013, 37015, 37065, 37083, 37117, 37147]}, {"Fips"=37119, "FipsAdj"=[37025, 37071, 37097, 37109, 37119, 37179, 45057]}, {"Fips"=37121, "FipsAdj"=[37011, 37111, 37121, 37199, 47019]}, {"Fips"=37123, "FipsAdj"=[37007, 37057, 37123, 37125, 37151, 37153, 37159]}, {"Fips"=37125, "FipsAdj"=[37037, 37051, 37085, 37093, 37105, 37123, 37125, 37151, 37153]}, {"Fips"=37127, "FipsAdj"=[37065, 37069, 37083, 37101, 37127, 37183, 37185]}, {"Fips"=37129, "FipsAdj"=[37019, 37129]}, {"Fips"=37131, "FipsAdj"=[37015, 37083, 37091, 37131, 37185, 51025, 51081]}, {"Fips"=37133, "FipsAdj"=[37031, 37061, 37103, 37133]}, {"Fips"=37135, "FipsAdj"=[37001, 37033, 37037, 37063, 37135]}, {"Fips"=37137, "FipsAdj"=[37013, 37031, 37049, 37095]}, {"Fips"=37139, "FipsAdj"=[37029, 37073, 37139, 37143]}, {"Fips"=37141, "FipsAdj"=[37017, 37019, 37047, 37061, 37129, 37133, 37141]}, {"Fips"=37143, "FipsAdj"=[37041, 37073, 37139, 37143, 37177]}, {"Fips"=37145, "FipsAdj"=[37033, 37063, 37077, 37135, 37145]}, {"Fips"=37147, "FipsAdj"=[37013, 37049, 37065, 37079, 37107, 37117, 37147]}, {"Fips"=37149, "FipsAdj"=[37089, 37149, 37161, 45045]}, {"Fips"=37151, "FipsAdj"=[37001, 37037, 37057, 37081, 37123, 37125]}, {"Fips"=37153, "FipsAdj"=[37007, 37093, 37123, 37125, 37153, 37165, 37167, 45025]}, {"Fips"=37155, "FipsAdj"=[37017, 37047, 37051, 37093, 37155, 37165, 45033, 45051]}, {"Fips"=37157, "FipsAdj"=[37001, 37033, 37067, 37081, 37157, 37169, 51089]}, {"Fips"=37159, "FipsAdj"=[37025, 37057, 37059, 37097, 37123, 37159]}, {"Fips"=37161, "FipsAdj"=[37021, 37023, 37045, 37089, 37111, 37149, 37161, 45021]}, {"Fips"=37163, "FipsAdj"=[37017, 37051, 37061, 37085, 37101, 37141, 37163]}, {"Fips"=37165, "FipsAdj"=[37093, 37125, 37153, 37155, 37165]}, {"Fips"=37167, "FipsAdj"=[37007, 37025, 37057, 37123, 37153, 37159, 37167]}, {"Fips"=37169, "FipsAdj"=[37067, 37081, 37157, 37169, 37171, 51089]}, {"Fips"=37171, "FipsAdj"=[37005, 37067, 37169, 37171, 37193, 37197, 51035, 51077]}, {"Fips"=37173, "FipsAdj"=[37075, 37087, 37099, 37113, 37173, 47009]}, {"Fips"=37175, "FipsAdj"=[37087, 37089, 37099, 37175, 45045, 45073]}, {"Fips"=37177, "FipsAdj"=[37029, 37053, 37055, 37095, 37139, 37143, 37177]}, {"Fips"=37179, "FipsAdj"=[37007, 37025, 37119, 37167, 37179, 45025]}, {"Fips"=37181, "FipsAdj"=[37069, 37077, 37181, 37185]}, {"Fips"=37183, "FipsAdj"=[37037, 37063, 37069, 37077, 37085, 37101, 37127]}, {"Fips"=37185, "FipsAdj"=[37069, 37083, 37127, 37131, 37181, 37185, 51025]}, {"Fips"=37187, "FipsAdj"=[37013, 37015, 37041, 37095, 37117, 37143, 37177]}, {"Fips"=37189, "FipsAdj"=[37009, 37011, 37027, 37189, 37193]}, {"Fips"=37191, "FipsAdj"=[37061, 37079, 37101, 37107, 37163, 37191]}, {"Fips"=37193, "FipsAdj"=[37003, 37005, 37009, 37027, 37097, 37171, 37189, 37193]}, {"Fips"=37195, "FipsAdj"=[37065, 37079, 37101, 37127, 37147, 37191]}, {"Fips"=37197, "FipsAdj"=[37059, 37067, 37097, 37171, 37193]}, {"Fips"=37199, "FipsAdj"=[37021, 37111, 37115, 37121, 37199]}, {"Fips"=38001, "FipsAdj"=[38001, 38011, 38037, 38041, 38085, 38087, 46031, 46063]}, {"Fips"=38003, "FipsAdj"=[38003, 38017, 38039, 38045, 38073, 38091]}, {"Fips"=38005, "FipsAdj"=[38005, 38027, 38063, 38069, 38071, 38095]}, {"Fips"=38007, "FipsAdj"=[38007, 38025, 38033, 38053, 38087]}, {"Fips"=38009, "FipsAdj"=[38009, 38049, 38069, 38075]}, {"Fips"=38011, "FipsAdj"=[30025, 38001, 38011, 38087]}, {"Fips"=38013, "FipsAdj"=[38013, 38023, 38061, 38075, 38101]}, {"Fips"=38015, "FipsAdj"=[38015, 38029, 38043, 38055, 38059, 38065]}, {"Fips"=38017, "FipsAdj"=[27027, 27107, 38003, 38017, 38073, 38077, 38091]}, {"Fips"=38019, "FipsAdj"=[38019, 38067, 38071, 38095]}, {"Fips"=38021, "FipsAdj"=[38021, 38045, 38051, 38073, 38081, 46013]}, {"Fips"=38023, "FipsAdj"=[30091, 38013, 38023]}, {"Fips"=38025, "FipsAdj"=[38007, 38025, 38053, 38055, 38057, 38061]}, {"Fips"=38027, "FipsAdj"=[38005, 38027, 38031, 38039, 38063]}, {"Fips"=38029, "FipsAdj"=[38015, 38029, 38043, 38047, 38051, 38059, 38085, 46021]}, {"Fips"=38031, "FipsAdj"=[38027, 38031, 38039, 38093]}, {"Fips"=38033, "FipsAdj"=[30025, 30109, 38007, 38033, 38053]}, {"Fips"=38035, "FipsAdj"=[27089, 27119, 38035, 38063, 38091, 38097]}, {"Fips"=38037, "FipsAdj"=[38001, 38037, 38041, 38059, 38085]}, {"Fips"=38039, "FipsAdj"=[38003, 38027, 38031, 38039, 38063, 38091]}, {"Fips"=38041, "FipsAdj"=[38001, 38037, 38041, 38087]}, {"Fips"=38043, "FipsAdj"=[38015, 38029, 38043, 38047, 38083, 38093]}, {"Fips"=38045, "FipsAdj"=[38003, 38021, 38045, 38047, 38051, 38073]}, {"Fips"=38047, "FipsAdj"=[38029, 38043, 38045, 38047, 38051]}, {"Fips"=38049, "FipsAdj"=[38009, 38049, 38055, 38069, 38075, 38083]}, {"Fips"=38051, "FipsAdj"=[38021, 38029, 38045, 38047, 38051, 46021]}, {"Fips"=38053, "FipsAdj"=[30083, 30085, 30109, 38007, 38025, 38033, 38053, 38061]}, {"Fips"=38055, "FipsAdj"=[38015, 38025, 38049, 38055, 38057, 38061, 38065, 38083]}, {"Fips"=38057, "FipsAdj"=[38025, 38055, 38057, 38059, 38065]}, {"Fips"=38059, "FipsAdj"=[38015, 38029, 38037, 38057, 38059, 38065, 38085]}, {"Fips"=38061, "FipsAdj"=[38013, 38025, 38053, 38055, 38061, 38101]}, {"Fips"=38063, "FipsAdj"=[38005, 38027, 38035, 38039, 38063, 38071, 38091]}, {"Fips"=38065, "FipsAdj"=[38015, 38055, 38057, 38059]}, {"Fips"=38067, "FipsAdj"=[27069, 27089, 38019, 38067]}, {"Fips"=38069, "FipsAdj"=[38005, 38009, 38049, 38069, 38079, 38083, 38095]}, {"Fips"=38071, "FipsAdj"=[38005, 38019, 38063, 38071, 38095]}, {"Fips"=38073, "FipsAdj"=[38003, 38017, 38021, 38045, 38073, 38077]}, {"Fips"=38075, "FipsAdj"=[38009, 38013, 38049, 38075]}, {"Fips"=38077, "FipsAdj"=[27027, 27155, 27167, 38017, 38073, 38077, 38081, 46091]}, {"Fips"=38079, "FipsAdj"=[38009, 38069, 38079]}, {"Fips"=38081, "FipsAdj"=[38021, 38073, 38077, 38081, 46013, 46091]}, {"Fips"=38083, "FipsAdj"=[38015, 38043, 38049, 38055, 38069, 38083]}, {"Fips"=38085, "FipsAdj"=[38001, 38029, 38037, 38059, 38085]}, {"Fips"=38087, "FipsAdj"=[30025, 38001, 38007, 38011, 38033, 38041, 38087]}, {"Fips"=38089, "FipsAdj"=[38007, 38025, 38037, 38041, 38057, 38059, 38087]}, {"Fips"=38091, "FipsAdj"=[38003, 38017, 38035, 38039, 38063, 38091]}, {"Fips"=38093, "FipsAdj"=[38003, 38031, 38039, 38043, 38045, 38047, 38093]}, {"Fips"=38095, "FipsAdj"=[38005, 38019, 38069, 38071, 38079]}, {"Fips"=38097, "FipsAdj"=[27107, 27119, 38017, 38035, 38091]}, {"Fips"=38099, "FipsAdj"=[27089, 38019, 38035, 38063, 38067, 38071]}, {"Fips"=38101, "FipsAdj"=[38013, 38049, 38055, 38061, 38075]}, {"Fips"=38103, "FipsAdj"=[38005, 38027, 38031, 38043, 38069, 38083, 38093]}, {"Fips"=38105, "FipsAdj"=[30083, 30085, 30091, 38013, 38023, 38053, 38061]}, {"Fips"=39001, "FipsAdj"=[21135, 21161, 39001, 39015, 39071, 39131]}, {"Fips"=39003, "FipsAdj"=[39003, 39011, 39063, 39065, 39137]}, {"Fips"=39005, "FipsAdj"=[39005, 39075, 39077, 39083, 39093, 39103, 39139]}, {"Fips"=39007, "FipsAdj"=[39007, 39055, 39085, 39155, 42039]}, {"Fips"=39009, "FipsAdj"=[39009, 39073, 39105, 39115, 39127, 39163, 39167]}, {"Fips"=39011, "FipsAdj"=[39003, 39011, 39065, 39091, 39107, 39149]}, {"Fips"=39013, "FipsAdj"=[39013, 39059, 39067, 39081, 39111, 39121, 54051]}, {"Fips"=39015, "FipsAdj"=[21023, 21161, 39001, 39015, 39025, 39027]}, {"Fips"=39017, "FipsAdj"=[18029, 18047, 18161, 39017, 39061, 39113, 39135]}, {"Fips"=39019, "FipsAdj"=[39019, 39029, 39067, 39081, 39151]}, {"Fips"=39021, "FipsAdj"=[39021, 39023, 39091, 39097, 39109, 39149]}, {"Fips"=39023, "FipsAdj"=[39021, 39023, 39057, 39097, 39109]}, {"Fips"=39025, "FipsAdj"=[21023, 21037, 21191, 39015, 39025, 39027, 39061]}, {"Fips"=39027, "FipsAdj"=[39015, 39025, 39027, 39047, 39057, 39071]}, {"Fips"=39029, "FipsAdj"=[39019, 39029, 39081, 39099, 39151, 42007, 42073]}, {"Fips"=39031, "FipsAdj"=[39031, 39059, 39075, 39083, 39089, 39119]}, {"Fips"=39033, "FipsAdj"=[39033, 39077, 39101, 39117, 39139, 39147]}, {"Fips"=39035, "FipsAdj"=[39035, 39055, 39085, 39093, 39103, 39133]}, {"Fips"=39037, "FipsAdj"=[18075, 18135, 18177, 39037, 39107, 39109, 39113, 39135]}, {"Fips"=39039, "FipsAdj"=[18003, 18033, 39039, 39069, 39125, 39137]}, {"Fips"=39041, "FipsAdj"=[39041, 39049, 39083, 39089, 39101, 39117]}, {"Fips"=39043, "FipsAdj"=[39043, 39077, 39093, 39123]}, {"Fips"=39045, "FipsAdj"=[39045, 39049, 39073, 39089, 39127]}, {"Fips"=39047, "FipsAdj"=[39027, 39047, 39057, 39071, 39097, 39129]}, {"Fips"=39049, "FipsAdj"=[39041, 39045, 39049, 39089, 39097, 39129]}, {"Fips"=39051, "FipsAdj"=[26059, 26091, 39051, 39069, 39095]}, {"Fips"=39053, "FipsAdj"=[39053, 39079, 39087, 39105, 39163, 54011]}, {"Fips"=39055, "FipsAdj"=[39007, 39035, 39055, 39085, 39133, 39153]}, {"Fips"=39057, "FipsAdj"=[39023, 39027, 39047, 39057, 39097, 39113]}, {"Fips"=39059, "FipsAdj"=[39013, 39031, 39059, 39067, 39119, 39121]}, {"Fips"=39061, "FipsAdj"=[18029, 18047, 21015, 21037, 21117, 39017, 39025, 39061]}, {"Fips"=39063, "FipsAdj"=[39003, 39063, 39065, 39069, 39137, 39147, 39173]}, {"Fips"=39065, "FipsAdj"=[39003, 39011, 39063, 39065, 39091, 39101, 39159]}, {"Fips"=39067, "FipsAdj"=[39013, 39019, 39059, 39067, 39081]}, {"Fips"=39069, "FipsAdj"=[39039, 39051, 39063, 39069, 39095, 39137, 39171]}, {"Fips"=39071, "FipsAdj"=[39001, 39015, 39027, 39047, 39071, 39131]}, {"Fips"=39073, "FipsAdj"=[39009, 39045, 39073, 39127, 39129, 39141]}, {"Fips"=39075, "FipsAdj"=[39005, 39031, 39075, 39083, 39151, 39157]}, {"Fips"=39077, "FipsAdj"=[39005, 39033, 39043, 39077, 39093, 39139, 39143]}, {"Fips"=39079, "FipsAdj"=[39053, 39079, 39087, 39131, 39141, 39145]}, {"Fips"=39081, "FipsAdj"=[39013, 39019, 39029, 39067, 39081, 54009, 54029]}, {"Fips"=39083, "FipsAdj"=[39005, 39031, 39041, 39075, 39083, 39089, 39117]}, {"Fips"=39085, "FipsAdj"=[39007, 39035, 39055]}, {"Fips"=39087, "FipsAdj"=[21019, 21089, 39053, 39079, 39087, 39145, 54011]}, {"Fips"=39089, "FipsAdj"=[39031, 39041, 39045, 39049, 39083, 39089, 39119]}, {"Fips"=39091, "FipsAdj"=[39011, 39021, 39065, 39091, 39149]}, {"Fips"=39093, "FipsAdj"=[39005, 39035, 39043, 39077, 39093]}, {"Fips"=39095, "FipsAdj"=[26091, 26115, 39051, 39069, 39095, 39123]}, {"Fips"=39097, "FipsAdj"=[39021, 39023, 39047, 39049, 39057, 39097, 39129]}, {"Fips"=39099, "FipsAdj"=[39029, 39099, 39133, 39151, 39155, 42073]}, {"Fips"=39101, "FipsAdj"=[39033, 39041, 39065, 39101, 39117, 39159]}, {"Fips"=39103, "FipsAdj"=[39005, 39035, 39093, 39103, 39153]}, {"Fips"=39105, "FipsAdj"=[39009, 39053, 39105, 39163, 54035, 54053]}, {"Fips"=39107, "FipsAdj"=[18001, 18075, 39011, 39037, 39107, 39149]}, {"Fips"=39109, "FipsAdj"=[39021, 39023, 39037, 39109, 39113]}, {"Fips"=39111, "FipsAdj"=[39013, 39111, 39121, 39167, 54051, 54095]}, {"Fips"=39113, "FipsAdj"=[39017, 39023, 39037, 39057, 39109, 39113, 39135]}, {"Fips"=39115, "FipsAdj"=[39009, 39115, 39119, 39121, 39127]}, {"Fips"=39117, "FipsAdj"=[39033, 39041, 39083, 39101, 39117]}, {"Fips"=39119, "FipsAdj"=[39031, 39059, 39089, 39115, 39119, 39121]}, {"Fips"=39121, "FipsAdj"=[39013, 39059, 39111, 39115, 39119, 39121]}, {"Fips"=39123, "FipsAdj"=[39043, 39095, 39123, 39143]}, {"Fips"=39125, "FipsAdj"=[18003, 39039, 39125, 39137]}, {"Fips"=39127, "FipsAdj"=[39009, 39045, 39073, 39089, 39115, 39119]}, {"Fips"=39129, "FipsAdj"=[39045, 39047, 39049, 39073, 39097, 39129]}, {"Fips"=39131, "FipsAdj"=[39001, 39071, 39079, 39131, 39141]}, {"Fips"=39133, "FipsAdj"=[39035, 39055, 39099, 39133, 39151, 39153]}, {"Fips"=39135, "FipsAdj"=[18161, 18177, 39017, 39037, 39113]}, {"Fips"=39137, "FipsAdj"=[39003, 39039, 39063, 39069, 39125, 39137, 39161]}, {"Fips"=39139, "FipsAdj"=[39005, 39033, 39077, 39083, 39117]}, {"Fips"=39141, "FipsAdj"=[39047, 39071, 39073, 39079, 39129, 39131, 39141]}, {"Fips"=39143, "FipsAdj"=[39043, 39077, 39123, 39143, 39147]}, {"Fips"=39145, "FipsAdj"=[21089, 21135, 39001, 39079, 39087, 39131]}, {"Fips"=39147, "FipsAdj"=[39033, 39063, 39077, 39143, 39147, 39173]}, {"Fips"=39149, "FipsAdj"=[39011, 39021, 39037, 39091, 39107, 39109]}, {"Fips"=39151, "FipsAdj"=[39019, 39029, 39075, 39099, 39133, 39151, 39153, 39157]}, {"Fips"=39153, "FipsAdj"=[39035, 39055, 39103, 39133, 39151, 39153]}, {"Fips"=39155, "FipsAdj"=[39007, 39055, 39099, 39133, 39155, 42039]}, {"Fips"=39157, "FipsAdj"=[39019, 39031, 39059, 39067, 39075, 39151]}, {"Fips"=39159, "FipsAdj"=[39021, 39041, 39049, 39065, 39091, 39097, 39101]}, {"Fips"=39161, "FipsAdj"=[18001, 18003, 39003, 39011, 39107, 39125, 39137]}, {"Fips"=39163, "FipsAdj"=[39009, 39053, 39073, 39079, 39105, 39141]}, {"Fips"=39165, "FipsAdj"=[39017, 39025, 39027, 39057, 39061, 39113]}, {"Fips"=39167, "FipsAdj"=[39009, 39111, 39115, 39121, 39167, 54073, 54095]}, {"Fips"=39169, "FipsAdj"=[39005, 39075, 39103, 39151, 39153]}, {"Fips"=39171, "FipsAdj"=[18033, 18151, 26059, 39039, 39051, 39069]}, {"Fips"=39173, "FipsAdj"=[39063, 39069, 39095, 39123, 39137, 39143, 39147]}, {"Fips"=39175, "FipsAdj"=[39033, 39063, 39065, 39101, 39147]}, {"Fips"=40001, "FipsAdj"=[5007, 5033, 5143, 40001, 40021, 40041]}, {"Fips"=40003, "FipsAdj"=[20007, 20077, 40003, 40047, 40053, 40093]}, {"Fips"=40005, "FipsAdj"=[40005, 40013, 40023, 40029, 40069, 40121]}, {"Fips"=40007, "FipsAdj"=[20025, 20119, 20175, 40007, 40045, 40059, 40139, 48295]}, {"Fips"=40009, "FipsAdj"=[40009, 40039, 40055, 40057, 40075, 40129, 40149, 48087]}, {"Fips"=40011, "FipsAdj"=[40011, 40015, 40017, 40039, 40043, 40073]}, {"Fips"=40013, "FipsAdj"=[40005, 40013, 40023, 40069, 40095, 48147, 48181]}, {"Fips"=40015, "FipsAdj"=[40011, 40015, 40017, 40031, 40039, 40051, 40075]}, {"Fips"=40017, "FipsAdj"=[40011, 40015, 40017, 40027, 40051, 40073, 40083, 40087]}, {"Fips"=40019, "FipsAdj"=[40019, 40049, 40067, 40069, 40085, 40095, 40099]}, {"Fips"=40021, "FipsAdj"=[40001, 40021, 40041, 40097, 40101, 40135]}, {"Fips"=40023, "FipsAdj"=[40005, 40013, 40023, 40089, 40127, 48277]}, {"Fips"=40025, "FipsAdj"=[8009, 20129, 35059, 40025, 40139, 48111]}, {"Fips"=40027, "FipsAdj"=[40017, 40027, 40087, 40109]}, {"Fips"=40029, "FipsAdj"=[40005, 40029, 40063, 40069, 40121]}, {"Fips"=40031, "FipsAdj"=[40015, 40031, 40033, 40051, 40075, 40137]}, {"Fips"=40033, "FipsAdj"=[40031, 40033, 40067, 40137, 40141, 48077]}, {"Fips"=40035, "FipsAdj"=[20021, 20099, 40035, 40041, 40097, 40105, 40115]}, {"Fips"=40037, "FipsAdj"=[40037, 40081, 40107, 40111, 40117, 40119]}, {"Fips"=40039, "FipsAdj"=[40009, 40011, 40015, 40039, 40043, 40129]}, {"Fips"=40041, "FipsAdj"=[5007, 29119, 40001, 40021, 40035, 40041, 40097]}, {"Fips"=40043, "FipsAdj"=[40011, 40039, 40043, 40045, 40093, 40129]}, {"Fips"=40045, "FipsAdj"=[40007, 40043, 40045, 40059, 40129, 40153, 48211]}, {"Fips"=40047, "FipsAdj"=[40003, 40047, 40053, 40071, 40073, 40083, 40093]}, {"Fips"=40049, "FipsAdj"=[40019, 40049, 40051, 40087, 40099, 40123]}, {"Fips"=40051, "FipsAdj"=[40015, 40017, 40031, 40049, 40051, 40087]}, {"Fips"=40053, "FipsAdj"=[20077, 20191, 40003, 40047, 40053]}, {"Fips"=40055, "FipsAdj"=[40009, 40055, 40057, 40065]}, {"Fips"=40057, "FipsAdj"=[40009, 40055, 40057, 40065, 48075, 48087]}, {"Fips"=40059, "FipsAdj"=[20025, 20033, 40007, 40045, 40059, 40151]}, {"Fips"=40061, "FipsAdj"=[40061, 40077, 40079, 40091, 40101, 40121]}, {"Fips"=40063, "FipsAdj"=[40029, 40063, 40091, 40107, 40121, 40123]}, {"Fips"=40065, "FipsAdj"=[40055, 40057, 40065, 40075, 40141, 48197]}, {"Fips"=40067, "FipsAdj"=[40019, 40033, 40067, 40085, 40137, 48077]}, {"Fips"=40069, "FipsAdj"=[40005, 40013, 40019, 40029, 40069, 40095, 40099]}, {"Fips"=40071, "FipsAdj"=[20035, 20191, 40047, 40053, 40071, 40103]}, {"Fips"=40073, "FipsAdj"=[40011, 40017, 40047, 40073, 40083, 40093]}, {"Fips"=40075, "FipsAdj"=[40009, 40015, 40031, 40055, 40065, 40075, 40141]}, {"Fips"=40077, "FipsAdj"=[40061, 40077, 40079, 40121]}, {"Fips"=40079, "FipsAdj"=[5113, 5127, 5131, 40061, 40077, 40079, 40089, 40127]}, {"Fips"=40081, "FipsAdj"=[40037, 40081, 40083, 40107, 40109, 40119]}, {"Fips"=40083, "FipsAdj"=[40017, 40047, 40073, 40081, 40083, 40103, 40109]}, {"Fips"=40085, "FipsAdj"=[40019, 40067, 40085, 40095, 48097, 48181]}, {"Fips"=40087, "FipsAdj"=[40017, 40027, 40049, 40051, 40087, 40123]}, {"Fips"=40089, "FipsAdj"=[5081, 5113, 5133, 40023, 40079, 40089, 40127, 48037]}, {"Fips"=40091, "FipsAdj"=[40061, 40063, 40091, 40101, 40107, 40111]}, {"Fips"=40093, "FipsAdj"=[40003, 40011, 40043, 40047, 40073, 40093, 40151]}, {"Fips"=40095, "FipsAdj"=[40013, 40019, 40069, 40085, 40095]}, {"Fips"=40097, "FipsAdj"=[40021, 40035, 40041, 40097, 40131]}, {"Fips"=40099, "FipsAdj"=[40019, 40049, 40069, 40099]}, {"Fips"=40101, "FipsAdj"=[40021, 40061, 40091, 40101, 40111, 40135]}, {"Fips"=40103, "FipsAdj"=[40047, 40071, 40083, 40103, 40113, 40117]}, {"Fips"=40105, "FipsAdj"=[20099, 20125, 40035, 40105, 40131]}, {"Fips"=40107, "FipsAdj"=[40037, 40063, 40081, 40091, 40107, 40111, 40125]}, {"Fips"=40109, "FipsAdj"=[40017, 40027, 40073, 40081, 40083, 40109]}, {"Fips"=40111, "FipsAdj"=[40037, 40091, 40101, 40107, 40111, 40143]}, {"Fips"=40113, "FipsAdj"=[20019, 20035, 40071, 40103, 40113, 40117, 40143]}, {"Fips"=40115, "FipsAdj"=[20021, 29119, 29145, 40035, 40041]}, {"Fips"=40117, "FipsAdj"=[40037, 40103, 40113, 40117, 40119]}, {"Fips"=40119, "FipsAdj"=[40037, 40081, 40083, 40103, 40117]}, {"Fips"=40121, "FipsAdj"=[40005, 40029, 40061, 40063, 40077, 40091, 40121]}, {"Fips"=40123, "FipsAdj"=[40029, 40049, 40063, 40069, 40087, 40099, 40123, 40125]}, {"Fips"=40125, "FipsAdj"=[40027, 40081, 40087, 40107, 40109, 40123, 40125]}, {"Fips"=40127, "FipsAdj"=[40005, 40023, 40077, 40079, 40089, 40121]}, {"Fips"=40129, "FipsAdj"=[40009, 40039, 40043, 40045, 40129, 48211]}, {"Fips"=40131, "FipsAdj"=[40035, 40097, 40105, 40131, 40143, 40145]}, {"Fips"=40133, "FipsAdj"=[40063, 40107, 40123, 40125]}, {"Fips"=40135, "FipsAdj"=[5033, 5131, 40001, 40021, 40061, 40079, 40101]}, {"Fips"=40137, "FipsAdj"=[40019, 40031, 40033, 40049, 40051, 40067]}, {"Fips"=40139, "FipsAdj"=[20129, 20175, 20189, 40007, 40025, 40139, 48195, 48357]}, {"Fips"=40141, "FipsAdj"=[40031, 40033, 40065, 40075, 40141, 48485]}, {"Fips"=40143, "FipsAdj"=[40037, 40111, 40113, 40117, 40131, 40143, 40145]}, {"Fips"=40145, "FipsAdj"=[40021, 40097, 40101, 40111, 40131, 40143]}, {"Fips"=40147, "FipsAdj"=[20019, 20125, 40105, 40113, 40131, 40143]}, {"Fips"=40149, "FipsAdj"=[40009, 40015, 40039, 40075]}, {"Fips"=40151, "FipsAdj"=[20007, 20033, 40003, 40059, 40093, 40151]}, {"Fips"=40153, "FipsAdj"=[40043, 40045, 40059, 40093, 40151]}, {"Fips"=41001, "FipsAdj"=[16003, 16087, 41001, 41023, 41045, 41061]}, {"Fips"=41003, "FipsAdj"=[41003, 41039, 41041, 41043]}, {"Fips"=41005, "FipsAdj"=[41005, 41027, 41047, 41051, 41065, 41067]}, {"Fips"=41007, "FipsAdj"=[41007, 41009, 41057, 41067, 53049]}, {"Fips"=41009, "FipsAdj"=[41007, 41009, 41051, 41057, 41067, 53011, 53015]}, {"Fips"=41011, "FipsAdj"=[41011, 41015]}, {"Fips"=41013, "FipsAdj"=[41013, 41017, 41023, 41025, 41031]}, {"Fips"=41015, "FipsAdj"=[6015, 41011, 41015, 41019]}, {"Fips"=41017, "FipsAdj"=[41013, 41017, 41025, 41031, 41035, 41037, 41039]}, {"Fips"=41019, "FipsAdj"=[41011, 41015, 41019, 41029, 41033, 41035]}, {"Fips"=41021, "FipsAdj"=[41021, 41049, 41055, 41065, 41069]}, {"Fips"=41023, "FipsAdj"=[41001, 41013, 41023, 41025, 41045, 41049, 41059, 41061]}, {"Fips"=41025, "FipsAdj"=[32013, 32031, 41013, 41017, 41023, 41025, 41037]}, {"Fips"=41027, "FipsAdj"=[41005, 41027, 41051, 41065, 53039]}, {"Fips"=41029, "FipsAdj"=[6093, 41019, 41029, 41033]}, {"Fips"=41031, "FipsAdj"=[41013, 41017, 41031, 41043, 41047, 41065]}, {"Fips"=41033, "FipsAdj"=[6015, 6093, 41015, 41019, 41029]}, {"Fips"=41035, "FipsAdj"=[6049, 6093, 41017, 41019, 41029, 41035, 41037]}, {"Fips"=41037, "FipsAdj"=[6049, 32031, 41017, 41025, 41035]}, {"Fips"=41039, "FipsAdj"=[41003, 41017, 41019, 41035, 41039, 41041]}, {"Fips"=41041, "FipsAdj"=[41003, 41039, 41041, 41053]}, {"Fips"=41043, "FipsAdj"=[41003, 41017, 41031, 41039, 41043, 41047]}, {"Fips"=41045, "FipsAdj"=[16027, 16073, 16075, 16087, 32013, 41001, 41023, 41025]}, {"Fips"=41047, "FipsAdj"=[41005, 41031, 41043, 41047, 41053, 41065]}, {"Fips"=41049, "FipsAdj"=[41021, 41023, 41049, 41059, 41069, 53005]}, {"Fips"=41051, "FipsAdj"=[41005, 41009, 41027, 41051, 41067, 53011]}, {"Fips"=41053, "FipsAdj"=[41003, 41041, 41043, 41047, 41053, 41057]}, {"Fips"=41055, "FipsAdj"=[41021, 41055, 41065]}, {"Fips"=41057, "FipsAdj"=[41007, 41009, 41041, 41053, 41057, 41067]}, {"Fips"=41059, "FipsAdj"=[41023, 41049, 41059, 41061, 41063, 53005, 53013]}, {"Fips"=41061, "FipsAdj"=[41001, 41023, 41059, 41061]}, {"Fips"=41063, "FipsAdj"=[16003, 16049, 16069, 41001, 41059, 41061, 41063, 53003, 53013]}, {"Fips"=41065, "FipsAdj"=[41005, 41021, 41027, 41031, 41047, 41055, 41065, 41069]}, {"Fips"=41067, "FipsAdj"=[41005, 41007, 41009, 41051, 41057, 41067]}, {"Fips"=41069, "FipsAdj"=[41013, 41021, 41023, 41031, 41049, 41065]}, {"Fips"=41071, "FipsAdj"=[41005, 41047, 41053, 41057, 41067]}, {"Fips"=42001, "FipsAdj"=[24013, 24021, 42001, 42041, 42055]}, {"Fips"=42003, "FipsAdj"=[42003, 42005, 42007, 42019, 42125]}, {"Fips"=42005, "FipsAdj"=[42003, 42005, 42019, 42031, 42063, 42065]}, {"Fips"=42007, "FipsAdj"=[39029, 42003, 42007, 42019, 42073, 42125]}, {"Fips"=42009, "FipsAdj"=[24001, 42009, 42013, 42021, 42057, 42061]}, {"Fips"=42011, "FipsAdj"=[42011, 42029, 42071, 42075, 42077, 42091]}, {"Fips"=42013, "FipsAdj"=[42009, 42013, 42021, 42027, 42033]}, {"Fips"=42015, "FipsAdj"=[36015, 36107, 42015, 42081, 42113, 42115, 42117]}, {"Fips"=42017, "FipsAdj"=[34005, 34019, 34021, 34041, 42017, 42077, 42091, 42095]}, {"Fips"=42019, "FipsAdj"=[42003, 42005, 42007, 42019, 42031, 42073, 42085]}, {"Fips"=42021, "FipsAdj"=[42009, 42013, 42021, 42033, 42063, 42111]}, {"Fips"=42023, "FipsAdj"=[42023, 42033, 42035, 42047, 42083]}, {"Fips"=42025, "FipsAdj"=[42025, 42077, 42079, 42089, 42095]}, {"Fips"=42027, "FipsAdj"=[42013, 42027, 42033, 42035, 42061, 42087]}, {"Fips"=42029, "FipsAdj"=[10003, 24015, 42011, 42029, 42045, 42071]}, {"Fips"=42031, "FipsAdj"=[42005, 42019, 42031, 42053, 42065]}, {"Fips"=42033, "FipsAdj"=[42013, 42021, 42023, 42027, 42033, 42035, 42047, 42063]}, {"Fips"=42035, "FipsAdj"=[42023, 42027, 42033, 42035, 42081, 42105]}, {"Fips"=42037, "FipsAdj"=[42037, 42079, 42081, 42093, 42097, 42107]}, {"Fips"=42039, "FipsAdj"=[39007, 39155, 42039, 42049, 42085, 42121]}, {"Fips"=42041, "FipsAdj"=[42001, 42041, 42043, 42055, 42099]}, {"Fips"=42043, "FipsAdj"=[42041, 42043, 42067, 42071, 42075, 42097, 42099, 42107]}, {"Fips"=42045, "FipsAdj"=[10003, 34015, 42029, 42045, 42091]}, {"Fips"=42047, "FipsAdj"=[42023, 42033, 42047, 42053, 42065, 42083]}, {"Fips"=42049, "FipsAdj"=[36013, 39007, 42039, 42049]}, {"Fips"=42051, "FipsAdj"=[24023, 42051, 42059, 42111, 42125, 42129, 54061]}, {"Fips"=42053, "FipsAdj"=[42031, 42047, 42053, 42065, 42121]}, {"Fips"=42055, "FipsAdj"=[24021, 24043, 42001, 42041, 42055, 42057, 42061, 42067]}, {"Fips"=42057, "FipsAdj"=[24001, 24043, 42009, 42055, 42057]}, {"Fips"=42059, "FipsAdj"=[42051, 42059, 42125, 54051, 54061]}, {"Fips"=42061, "FipsAdj"=[42009, 42013, 42027, 42055, 42057, 42061, 42067]}, {"Fips"=42063, "FipsAdj"=[42005, 42021, 42033, 42063, 42065]}, {"Fips"=42065, "FipsAdj"=[42005, 42031, 42033, 42047, 42053, 42063]}, {"Fips"=42067, "FipsAdj"=[42043, 42055, 42061, 42067, 42087, 42097, 42099]}, {"Fips"=42069, "FipsAdj"=[42069, 42079, 42089, 42115, 42127]}, {"Fips"=42071, "FipsAdj"=[24015, 24025, 42011, 42029, 42043, 42071, 42075]}, {"Fips"=42073, "FipsAdj"=[39029, 39099, 42007, 42019, 42073]}, {"Fips"=42075, "FipsAdj"=[42011, 42043, 42071, 42075]}, {"Fips"=42077, "FipsAdj"=[42011, 42017, 42025, 42077, 42091, 42095]}, {"Fips"=42079, "FipsAdj"=[42025, 42037, 42069, 42079, 42089, 42107, 42113]}, {"Fips"=42081, "FipsAdj"=[42015, 42035, 42037, 42081, 42093, 42097, 42105, 42113, 42117]}, {"Fips"=42083, "FipsAdj"=[36003, 36009, 42023, 42047, 42083, 42105]}, {"Fips"=42085, "FipsAdj"=[39099, 39155, 42019, 42039, 42073, 42085]}, {"Fips"=42087, "FipsAdj"=[42027, 42061, 42067, 42087, 42109]}, {"Fips"=42089, "FipsAdj"=[34037, 34041, 42025, 42069, 42079, 42089, 42095, 42103]}, {"Fips"=42091, "FipsAdj"=[42011, 42017, 42029, 42045, 42077, 42091]}, {"Fips"=42093, "FipsAdj"=[42037, 42081, 42093]}, {"Fips"=42095, "FipsAdj"=[34041, 42017, 42025, 42077, 42089]}, {"Fips"=42097, "FipsAdj"=[42037, 42043, 42067, 42081, 42093, 42097, 42099, 42107, 42109]}, {"Fips"=42099, "FipsAdj"=[42041, 42043, 42055, 42067, 42097]}, {"Fips"=42101, "FipsAdj"=[34005, 34007, 34015, 42017, 42045, 42091]}, {"Fips"=42103, "FipsAdj"=[34037, 36071, 36105, 42089, 42103]}, {"Fips"=42105, "FipsAdj"=[36003, 36101, 42023, 42035, 42081, 42083, 42105]}, {"Fips"=42107, "FipsAdj"=[42011, 42025, 42037, 42043, 42075, 42077, 42079, 42097]}, {"Fips"=42109, "FipsAdj"=[42067, 42087, 42097, 42109]}, {"Fips"=42111, "FipsAdj"=[24001, 24023, 42009, 42021, 42051, 42111]}, {"Fips"=42113, "FipsAdj"=[42015, 42037, 42079, 42081, 42113]}, {"Fips"=42115, "FipsAdj"=[36007, 36107, 42015, 42069, 42115, 42127]}, {"Fips"=42117, "FipsAdj"=[36015, 36101, 42015, 42081, 42105]}, {"Fips"=42119, "FipsAdj"=[42027, 42035, 42081, 42087, 42097, 42109]}, {"Fips"=42121, "FipsAdj"=[42019, 42031, 42039, 42053, 42085, 42121]}, {"Fips"=42123, "FipsAdj"=[36009, 36013, 42039, 42047, 42049, 42053, 42083, 42121]}, {"Fips"=42125, "FipsAdj"=[42003, 42007, 42051, 42059, 42125, 42129, 54009, 54029, 54051]}, {"Fips"=42127, "FipsAdj"=[36007, 36025, 36105, 42069, 42089, 42103, 42115]}, {"Fips"=42129, "FipsAdj"=[42003, 42005, 42021, 42051, 42063, 42111, 42125]}, {"Fips"=42131, "FipsAdj"=[42015, 42069, 42079, 42113, 42115]}, {"Fips"=42133, "FipsAdj"=[24005, 24013, 24025, 42001, 42041, 42043, 42071]}, {"Fips"=44001, "FipsAdj"=[25005, 44001, 44003, 44005]}, {"Fips"=44003, "FipsAdj"=[9011, 9015, 44001, 44003, 44005, 44007]}, {"Fips"=44005, "FipsAdj"=[25005, 44001, 44003, 44005]}, {"Fips"=44007, "FipsAdj"=[9015, 25005, 25021, 25027, 44001, 44003]}, {"Fips"=44009, "FipsAdj"=[9011, 36103, 44003, 44005]}, {"Fips"=45001, "FipsAdj"=[13105, 45001, 45007, 45045, 45047, 45059]}, {"Fips"=45003, "FipsAdj"=[13033, 13245, 45003, 45011, 45037, 45063, 45075]}, {"Fips"=45005, "FipsAdj"=[13033, 13251, 45005, 45009, 45011, 45029]}, {"Fips"=45007, "FipsAdj"=[13105, 13147, 45001, 45007, 45045, 45059, 45073]}, {"Fips"=45009, "FipsAdj"=[45005, 45009, 45011, 45029, 45049]}, {"Fips"=45011, "FipsAdj"=[13033, 45003, 45005, 45009, 45011]}, {"Fips"=45013, "FipsAdj"=[45013, 45029, 45049]}, {"Fips"=45015, "FipsAdj"=[45015, 45019, 45027, 45035, 45043, 45075]}, {"Fips"=45017, "FipsAdj"=[45017, 45027, 45063, 45075, 45079]}, {"Fips"=45019, "FipsAdj"=[45015, 45019, 45029, 45035]}, {"Fips"=45021, "FipsAdj"=[37045, 37161, 45021, 45083, 45087]}, {"Fips"=45023, "FipsAdj"=[45023, 45039, 45057, 45087]}, {"Fips"=45025, "FipsAdj"=[37007, 37153, 37179, 45025, 45031, 45055, 45057]}, {"Fips"=45027, "FipsAdj"=[45015, 45017, 45027, 45041, 45075, 45085]}, {"Fips"=45029, "FipsAdj"=[45005, 45009, 45013, 45019, 45029, 45035, 45049]}, {"Fips"=45031, "FipsAdj"=[45025, 45031, 45041, 45055, 45061]}, {"Fips"=45033, "FipsAdj"=[37047, 37155, 45033, 45041, 45051, 45067]}, {"Fips"=45035, "FipsAdj"=[45015, 45019, 45029, 45035]}, {"Fips"=45037, "FipsAdj"=[13073, 13245, 45003, 45037, 45047, 45065]}, {"Fips"=45039, "FipsAdj"=[45023, 45039, 45055, 45057, 45071, 45079]}, {"Fips"=45041, "FipsAdj"=[45027, 45031, 45033, 45041, 45061, 45067, 45069, 45085]}, {"Fips"=45043, "FipsAdj"=[45015, 45019, 45043, 45051, 45067]}, {"Fips"=45045, "FipsAdj"=[37089, 37149, 37175, 45001, 45007, 45045, 45059, 45077]}, {"Fips"=45047, "FipsAdj"=[45001, 45037, 45047, 45059, 45065, 45071]}, {"Fips"=45049, "FipsAdj"=[13103, 13251, 45005, 45009, 45013, 45029, 45049]}, {"Fips"=45051, "FipsAdj"=[37019, 37047, 37155, 45033, 45043, 45051]}, {"Fips"=45053, "FipsAdj"=[13051, 13103, 45013, 45049]}, {"Fips"=45055, "FipsAdj"=[45025, 45031, 45039, 45055, 45057, 45061, 45079]}, {"Fips"=45057, "FipsAdj"=[37119, 37179, 45023, 45025, 45039, 45055, 45057]}, {"Fips"=45059, "FipsAdj"=[45001, 45007, 45045, 45047, 45059, 45071, 45083]}, {"Fips"=45061, "FipsAdj"=[45031, 45041, 45055, 45061]}, {"Fips"=45063, "FipsAdj"=[45003, 45017, 45063, 45071, 45075, 45079]}, {"Fips"=45065, "FipsAdj"=[13073, 13105, 13181, 45001, 45037, 45047]}, {"Fips"=45067, "FipsAdj"=[45033, 45041, 45043, 45051, 45067]}, {"Fips"=45069, "FipsAdj"=[37007, 37153, 37155, 37165, 45025, 45031, 45033, 45041]}, {"Fips"=45071, "FipsAdj"=[45039, 45047, 45059, 45063, 45071, 45079, 45081]}, {"Fips"=45073, "FipsAdj"=[13119, 13137, 13147, 13241, 13257, 37099, 37113, 37175, 45007, 45073]}, {"Fips"=45075, "FipsAdj"=[45003, 45009, 45011, 45015, 45017, 45027, 45029, 45035, 45063]}, {"Fips"=45077, "FipsAdj"=[37175, 45007, 45045, 45073]}, {"Fips"=45079, "FipsAdj"=[45017, 45039, 45055, 45063, 45071, 45079]}, {"Fips"=45081, "FipsAdj"=[45003, 45037, 45047, 45063, 45071]}, {"Fips"=45083, "FipsAdj"=[37149, 37161, 45021, 45045, 45059, 45083]}, {"Fips"=45085, "FipsAdj"=[45017, 45027, 45041, 45055, 45061, 45079]}, {"Fips"=45087, "FipsAdj"=[45021, 45023, 45039, 45059, 45071, 45083, 45087]}, {"Fips"=45089, "FipsAdj"=[45015, 45027, 45041, 45043, 45067]}, {"Fips"=45091, "FipsAdj"=[37045, 37071, 37119, 45021, 45023, 45057, 45087]}, {"Fips"=46003, "FipsAdj"=[46003, 46015, 46023, 46035, 46043, 46073]}, {"Fips"=46005, "FipsAdj"=[46005, 46025, 46059, 46073, 46077, 46111]}, {"Fips"=46007, "FipsAdj"=[31031, 46007, 46071, 46095, 46113]}, {"Fips"=46009, "FipsAdj"=[31107, 46009, 46023, 46067]}, {"Fips"=46011, "FipsAdj"=[27081, 27117, 46011, 46039, 46057, 46077, 46079]}, {"Fips"=46013, "FipsAdj"=[38021, 38081, 46013, 46037, 46045, 46049, 46089, 46091]}, {"Fips"=46015, "FipsAdj"=[46003, 46015, 46017, 46023, 46073]}, {"Fips"=46017, "FipsAdj"=[46015, 46017, 46059, 46069, 46073]}, {"Fips"=46019, "FipsAdj"=[30011, 46019, 46063, 46081, 46093, 46105]}, {"Fips"=46021, "FipsAdj"=[38029, 38051, 46021, 46031, 46089]}, {"Fips"=46023, "FipsAdj"=[31015, 31107, 46003, 46009, 46015, 46023, 46043, 46053, 46067]}, {"Fips"=46025, "FipsAdj"=[46005, 46025, 46029, 46037, 46057, 46077]}, {"Fips"=46027, "FipsAdj"=[31027, 31051, 46027, 46083, 46125, 46127]}, {"Fips"=46029, "FipsAdj"=[46025, 46029, 46037, 46039, 46051]}, {"Fips"=46031, "FipsAdj"=[38001, 38029, 38085, 46021, 46031, 46041, 46105, 46129]}, {"Fips"=46033, "FipsAdj"=[46033, 46047, 46103, 46113, 56027]}, {"Fips"=46035, "FipsAdj"=[46003, 46035, 46043, 46061, 46067]}, {"Fips"=46037, "FipsAdj"=[46013, 46025, 46029, 46037, 46051, 46091, 46109]}, {"Fips"=46039, "FipsAdj"=[27073, 27081, 27173, 46011, 46029, 46039, 46051]}, {"Fips"=46041, "FipsAdj"=[46031, 46041, 46055, 46107, 46117, 46119, 46129]}, {"Fips"=46043, "FipsAdj"=[46003, 46023, 46035, 46043]}, {"Fips"=46045, "FipsAdj"=[46013, 46045, 46049, 46089, 46107]}, {"Fips"=46047, "FipsAdj"=[31045, 31165, 46033, 46047, 46113]}, {"Fips"=46049, "FipsAdj"=[46013, 46045, 46049, 46059, 46069, 46107]}, {"Fips"=46051, "FipsAdj"=[27011, 27073, 46029, 46037, 46039, 46051]}, {"Fips"=46053, "FipsAdj"=[31015, 31103, 46023, 46053, 46085]}, {"Fips"=46055, "FipsAdj"=[46041, 46055, 46071, 46075, 46093, 46103, 46117]}, {"Fips"=46057, "FipsAdj"=[46011, 46025, 46029, 46039, 46057]}, {"Fips"=46059, "FipsAdj"=[46005, 46017, 46049, 46059, 46069, 46073]}, {"Fips"=46061, "FipsAdj"=[46035, 46061, 46067, 46087, 46097]}, {"Fips"=46063, "FipsAdj"=[30011, 30025, 38001, 38011, 46019, 46063]}, {"Fips"=46065, "FipsAdj"=[46065, 46069, 46085, 46117]}, {"Fips"=46067, "FipsAdj"=[46009, 46023, 46035, 46043, 46061, 46067, 46087, 46125]}, {"Fips"=46069, "FipsAdj"=[46017, 46049, 46059, 46065, 46069, 46085, 46107]}, {"Fips"=46071, "FipsAdj"=[46007, 46055, 46071, 46075, 46095, 46103, 46113]}, {"Fips"=46073, "FipsAdj"=[46003, 46005, 46015, 46017, 46059, 46073]}, {"Fips"=46075, "FipsAdj"=[46055, 46071, 46075, 46085, 46095]}, {"Fips"=46077, "FipsAdj"=[46005, 46011, 46025, 46057, 46077, 46079, 46097]}, {"Fips"=46079, "FipsAdj"=[46011, 46077, 46079, 46087, 46097, 46099]}, {"Fips"=46081, "FipsAdj"=[46019, 46081, 46093, 46103, 56011]}, {"Fips"=46083, "FipsAdj"=[19119, 19167, 46027, 46083, 46099, 46125]}, {"Fips"=46085, "FipsAdj"=[46015, 46017, 46023, 46053, 46065, 46069, 46075, 46085, 46095, 46117]}, {"Fips"=46087, "FipsAdj"=[46061, 46067, 46079, 46087, 46097, 46099]}, {"Fips"=46089, "FipsAdj"=[38021, 38051, 46013, 46021, 46045, 46089]}, {"Fips"=46091, "FipsAdj"=[38077, 38081, 46013, 46037, 46091]}, {"Fips"=46093, "FipsAdj"=[46019, 46055, 46081, 46093, 46103, 46105]}, {"Fips"=46095, "FipsAdj"=[46007, 46071, 46075, 46085, 46095, 46121]}, {"Fips"=46097, "FipsAdj"=[46061, 46077, 46079, 46087, 46097]}, {"Fips"=46099, "FipsAdj"=[19119, 27117, 27133, 46079, 46083, 46087, 46099, 46101]}, {"Fips"=46101, "FipsAdj"=[27081, 27117, 27133, 46011, 46079, 46099]}, {"Fips"=46103, "FipsAdj"=[46033, 46055, 46071, 46081, 46093, 46103, 46113]}, {"Fips"=46105, "FipsAdj"=[38001, 46019, 46031, 46063, 46093, 46105]}, {"Fips"=46107, "FipsAdj"=[46041, 46045, 46049, 46069, 46107, 46119]}, {"Fips"=46109, "FipsAdj"=[27011, 27155, 38077, 38081, 46037, 46051, 46091]}, {"Fips"=46111, "FipsAdj"=[46003, 46005, 46035, 46061, 46073, 46077, 46097]}, {"Fips"=46113, "FipsAdj"=[31031, 31045, 31161, 46007, 46033, 46047, 46071, 46103]}, {"Fips"=46115, "FipsAdj"=[46005, 46013, 46025, 46037, 46049, 46059]}, {"Fips"=46117, "FipsAdj"=[46041, 46055, 46065, 46075, 46085, 46117, 46119]}, {"Fips"=46119, "FipsAdj"=[46041, 46065, 46069, 46107, 46117]}, {"Fips"=46121, "FipsAdj"=[31031, 31103, 46007, 46071, 46095, 46121]}, {"Fips"=46123, "FipsAdj"=[31031, 31103, 46053, 46085, 46095, 46121]}, {"Fips"=46125, "FipsAdj"=[46027, 46067, 46083, 46087, 46099, 46125]}, {"Fips"=46127, "FipsAdj"=[19149, 19167, 19193, 31043, 31051, 46027, 46083]}, {"Fips"=46129, "FipsAdj"=[46021, 46031, 46041, 46045, 46089, 46107]}, {"Fips"=46135, "FipsAdj"=[31027, 31107, 46009, 46027, 46067, 46125]}, {"Fips"=46137, "FipsAdj"=[46031, 46041, 46055, 46093, 46105, 46117]}, {"Fips"=47001, "FipsAdj"=[47001, 47013, 47093, 47129, 47145, 47151]}, {"Fips"=47003, "FipsAdj"=[47003, 47031, 47103, 47117, 47127]}, {"Fips"=47005, "FipsAdj"=[47005, 47017, 47039, 47079, 47083, 47085, 47135]}, {"Fips"=47007, "FipsAdj"=[47007, 47035, 47065, 47143, 47153]}, {"Fips"=47009, "FipsAdj"=[37075, 37173, 47009, 47093, 47105, 47123]}, {"Fips"=47011, "FipsAdj"=[13213, 13313, 47011, 47065, 47107, 47121]}, {"Fips"=47013, "FipsAdj"=[21147, 21235, 47001, 47013, 47025, 47151]}, {"Fips"=47015, "FipsAdj"=[47015, 47031, 47041, 47149, 47177]}, {"Fips"=47017, "FipsAdj"=[47005, 47017, 47039, 47053, 47077, 47079, 47113]}, {"Fips"=47019, "FipsAdj"=[37011, 37121, 47019, 47091, 47163, 47171]}, {"Fips"=47021, "FipsAdj"=[47021, 47037, 47043, 47125, 47147]}, {"Fips"=47023, "FipsAdj"=[47023, 47069, 47071, 47077, 47109]}, {"Fips"=47025, "FipsAdj"=[21013, 21235, 47013, 47025, 47057, 47067, 47173]}, {"Fips"=47027, "FipsAdj"=[21053, 21057, 21171, 47027, 47087, 47111, 47133]}, {"Fips"=47029, "FipsAdj"=[37087, 37115, 47029, 47059, 47063, 47089]}, {"Fips"=47031, "FipsAdj"=[47003, 47015, 47031, 47051, 47061, 47127, 47149]}, {"Fips"=47033, "FipsAdj"=[47033, 47045, 47053, 47075, 47097]}, {"Fips"=47035, "FipsAdj"=[47007, 47035, 47049, 47129, 47141, 47143, 47145, 47175]}, {"Fips"=47037, "FipsAdj"=[47021, 47037, 47147, 47149, 47165, 47187]}, {"Fips"=47039, "FipsAdj"=[47005, 47017, 47039, 47071, 47077, 47135]}, {"Fips"=47041, "FipsAdj"=[47015, 47041, 47141, 47159, 47177, 47185]}, {"Fips"=47043, "FipsAdj"=[47021, 47043, 47081, 47083, 47085, 47125]}, {"Fips"=47045, "FipsAdj"=[5093, 29155, 47033, 47045, 47053, 47095, 47097]}, {"Fips"=47047, "FipsAdj"=[28009, 28093, 47047, 47069, 47075, 47157]}, {"Fips"=47049, "FipsAdj"=[47035, 47049, 47129, 47133, 47137, 47141]}, {"Fips"=47051, "FipsAdj"=[1071, 1089, 47031, 47051, 47061, 47103, 47115]}, {"Fips"=47053, "FipsAdj"=[47017, 47033, 47045, 47053, 47113, 47131]}, {"Fips"=47055, "FipsAdj"=[1077, 1083, 47055, 47099, 47103, 47117]}, {"Fips"=47057, "FipsAdj"=[47025, 47057, 47063, 47067, 47073, 47089, 47093]}, {"Fips"=47059, "FipsAdj"=[37115, 47029, 47059, 47063, 47073, 47171]}, {"Fips"=47061, "FipsAdj"=[47031, 47051, 47061, 47115, 47153]}, {"Fips"=47063, "FipsAdj"=[47029, 47057, 47059, 47063, 47073]}, {"Fips"=47065, "FipsAdj"=[13047, 13083, 13295, 13313, 47007, 47011, 47065, 47115, 47121, 47143]}, {"Fips"=47067, "FipsAdj"=[47025, 47057, 47067, 47073, 51105]}, {"Fips"=47069, "FipsAdj"=[28003, 28009, 28139, 47023, 47047, 47069, 47075, 47109]}, {"Fips"=47071, "FipsAdj"=[1077, 28003, 28141, 47023, 47039, 47071, 47077, 47109]}, {"Fips"=47073, "FipsAdj"=[47057, 47059, 47063, 47067, 47073, 47163, 47179]}, {"Fips"=47075, "FipsAdj"=[47033, 47047, 47069, 47075, 47097, 47113]}, {"Fips"=47077, "FipsAdj"=[47017, 47023, 47039, 47071, 47077]}, {"Fips"=47079, "FipsAdj"=[21035, 21083, 47005, 47017, 47079, 47161]}, {"Fips"=47081, "FipsAdj"=[47043, 47081, 47085, 47101, 47119, 47135]}, {"Fips"=47083, "FipsAdj"=[47005, 47043, 47083, 47085, 47125]}, {"Fips"=47085, "FipsAdj"=[47005, 47043, 47081, 47083, 47085]}, {"Fips"=47087, "FipsAdj"=[47027, 47087, 47111, 47133, 47141]}, {"Fips"=47089, "FipsAdj"=[47029, 47057, 47063, 47089, 47093]}, {"Fips"=47091, "FipsAdj"=[37009, 37011, 37189, 47019, 47091, 47163, 51077]}, {"Fips"=47093, "FipsAdj"=[47001, 47009, 47057, 47089, 47093, 47105, 47145, 47155]}, {"Fips"=47095, "FipsAdj"=[21075, 29143, 29155, 47045, 47095]}, {"Fips"=47097, "FipsAdj"=[5093, 47033, 47045, 47075, 47097]}, {"Fips"=47099, "FipsAdj"=[1077, 47055, 47099, 47101, 47119]}, {"Fips"=47101, "FipsAdj"=[47081, 47099, 47101, 47119, 47135]}, {"Fips"=47103, "FipsAdj"=[1083, 1089, 47003, 47051, 47055, 47103, 47117]}, {"Fips"=47105, "FipsAdj"=[47009, 47093, 47105, 47107, 47123]}, {"Fips"=47107, "FipsAdj"=[47011, 47105, 47107, 47121, 47123, 47139]}, {"Fips"=47109, "FipsAdj"=[28003, 47023, 47069, 47071]}, {"Fips"=47111, "FipsAdj"=[21003, 21171, 47027, 47087, 47111, 47159, 47165]}, {"Fips"=47113, "FipsAdj"=[47017, 47023, 47033, 47053, 47069, 47075, 47077]}, {"Fips"=47115, "FipsAdj"=[1071, 13083, 47051, 47061, 47065, 47115]}, {"Fips"=47117, "FipsAdj"=[47003, 47055, 47103, 47117, 47119, 47149]}, {"Fips"=47119, "FipsAdj"=[47055, 47081, 47099, 47101, 47117, 47119]}, {"Fips"=47121, "FipsAdj"=[47011, 47065, 47107, 47121, 47143]}, {"Fips"=47123, "FipsAdj"=[37039, 37075, 47009, 47105, 47107, 47123]}, {"Fips"=47125, "FipsAdj"=[21047, 21219, 47021, 47043, 47083, 47125, 47147]}, {"Fips"=47127, "FipsAdj"=[47003, 47031, 47051, 47103]}, {"Fips"=47129, "FipsAdj"=[47001, 47035, 47049, 47129, 47145]}, {"Fips"=47131, "FipsAdj"=[21075, 21105, 47045, 47053, 47095, 47131]}, {"Fips"=47133, "FipsAdj"=[47027, 47049, 47087, 47133, 47137]}, {"Fips"=47135, "FipsAdj"=[47005, 47039, 47081, 47085, 47101, 47135]}, {"Fips"=47137, "FipsAdj"=[21053, 21231, 47027, 47049, 47133, 47137]}, {"Fips"=47139, "FipsAdj"=[13111, 13213, 37039, 47011, 47107, 47123]}, {"Fips"=47141, "FipsAdj"=[47035, 47041, 47049, 47087, 47133, 47141, 47159]}, {"Fips"=47143, "FipsAdj"=[47007, 47035, 47065, 47121, 47143]}, {"Fips"=47145, "FipsAdj"=[47001, 47035, 47093, 47105, 47107, 47121, 47129, 47143]}, {"Fips"=47147, "FipsAdj"=[21141, 21213, 21219, 47021, 47037, 47125, 47147]}, {"Fips"=47149, "FipsAdj"=[47003, 47015, 47031, 47037, 47117, 47149, 47187]}, {"Fips"=47151, "FipsAdj"=[21147, 21231, 47001, 47013, 47049, 47129, 47137]}, {"Fips"=47153, "FipsAdj"=[47007, 47061, 47065, 47115, 47153, 47175]}, {"Fips"=47155, "FipsAdj"=[37087, 37173, 47009, 47029, 47089, 47093]}, {"Fips"=47157, "FipsAdj"=[5035, 5093, 28033, 28093, 47047, 47157]}, {"Fips"=47159, "FipsAdj"=[47041, 47087, 47111, 47141, 47159, 47169]}, {"Fips"=47161, "FipsAdj"=[21035, 21047, 21221, 47005, 47079, 47083, 47125]}, {"Fips"=47163, "FipsAdj"=[47019, 47073, 47091, 47163, 47179, 51169, 51191]}, {"Fips"=47165, "FipsAdj"=[21003, 21213, 47037, 47111, 47147, 47165, 47169]}, {"Fips"=47167, "FipsAdj"=[5035, 5093, 47047, 47075, 47097, 47157]}, {"Fips"=47169, "FipsAdj"=[47111, 47159, 47165, 47169]}, {"Fips"=47171, "FipsAdj"=[37115, 37121, 37199, 47019, 47059, 47171]}, {"Fips"=47173, "FipsAdj"=[47001, 47013, 47025, 47057, 47093]}, {"Fips"=47175, "FipsAdj"=[47007, 47035, 47153, 47175, 47177]}, {"Fips"=47177, "FipsAdj"=[47015, 47031, 47041, 47061, 47153, 47175, 47177]}, {"Fips"=47179, "FipsAdj"=[47019, 47059, 47073, 47163, 47171]}, {"Fips"=47181, "FipsAdj"=[1077, 47039, 47071, 47099, 47101, 47135]}, {"Fips"=47183, "FipsAdj"=[21083, 21105, 47017, 47053, 47079, 47131]}, {"Fips"=47185, "FipsAdj"=[47035, 47041, 47141, 47175, 47177]}, {"Fips"=47187, "FipsAdj"=[47021, 47037, 47043, 47081, 47117, 47119, 47149]}, {"Fips"=47189, "FipsAdj"=[47015, 47037, 47041, 47149, 47159, 47165, 47169]}, {"Fips"=48001, "FipsAdj"=[48001, 48073, 48161, 48213, 48225]}, {"Fips"=48003, "FipsAdj"=[35025, 48003, 48135, 48165, 48317, 48329]}, {"Fips"=48005, "FipsAdj"=[48005, 48073, 48225, 48241, 48347, 48373, 48405, 48455]}, {"Fips"=48007, "FipsAdj"=[48007, 48057, 48355, 48391]}, {"Fips"=48009, "FipsAdj"=[48009, 48023, 48077, 48237, 48447, 48485, 48487]}, {"Fips"=48011, "FipsAdj"=[48011, 48045, 48065, 48129, 48179, 48375, 48381]}, {"Fips"=48013, "FipsAdj"=[48013, 48029, 48163, 48255, 48283, 48297, 48311, 48325]}, {"Fips"=48015, "FipsAdj"=[48015, 48089, 48149, 48157, 48473, 48477]}, {"Fips"=48017, "FipsAdj"=[35009, 35041, 48017, 48079, 48219, 48279]}, {"Fips"=48019, "FipsAdj"=[48019, 48029, 48259, 48265, 48325, 48385]}, {"Fips"=48021, "FipsAdj"=[48021, 48055, 48149, 48287, 48453]}, {"Fips"=48023, "FipsAdj"=[48009, 48023, 48155, 48207, 48275, 48447, 48485, 48487]}, {"Fips"=48025, "FipsAdj"=[48025, 48175, 48255, 48297, 48391]}, {"Fips"=48027, "FipsAdj"=[48027, 48053, 48099, 48145, 48281, 48309, 48331]}, {"Fips"=48029, "FipsAdj"=[48013, 48019, 48029, 48091, 48187, 48259, 48325]}, {"Fips"=48031, "FipsAdj"=[48031, 48053, 48091, 48171, 48209, 48259, 48299]}, {"Fips"=48033, "FipsAdj"=[48033, 48115, 48169, 48227, 48305, 48317, 48335]}, {"Fips"=48035, "FipsAdj"=[48035, 48099, 48143, 48193, 48217, 48251, 48309]}, {"Fips"=48037, "FipsAdj"=[5081, 5091, 40089, 48037, 48067, 48343]}, {"Fips"=48039, "FipsAdj"=[48039, 48157, 48167, 48201, 48321]}, {"Fips"=48041, "FipsAdj"=[48041, 48051, 48185, 48289, 48313, 48395]}, {"Fips"=48043, "FipsAdj"=[48043, 48243, 48371, 48377]}, {"Fips"=48045, "FipsAdj"=[48011, 48045, 48129, 48153, 48191, 48345]}, {"Fips"=48047, "FipsAdj"=[48047, 48131, 48215, 48247, 48249, 48261, 48273]}, {"Fips"=48049, "FipsAdj"=[48049, 48059, 48083, 48093, 48133, 48307, 48333]}, {"Fips"=48051, "FipsAdj"=[48041, 48051, 48287, 48331, 48395]}, {"Fips"=48053, "FipsAdj"=[48027, 48031, 48053, 48281, 48299, 48411, 48453]}, {"Fips"=48055, "FipsAdj"=[48021, 48055, 48149, 48177, 48187, 48209]}, {"Fips"=48057, "FipsAdj"=[48007, 48057, 48239, 48321, 48391]}, {"Fips"=48059, "FipsAdj"=[48049, 48059, 48083, 48133, 48253, 48417]}, {"Fips"=48061, "FipsAdj"=[48061, 48215]}, {"Fips"=48063, "FipsAdj"=[48063, 48159, 48343, 48449, 48459]}, {"Fips"=48065, "FipsAdj"=[48011, 48065, 48129, 48179, 48233, 48341, 48375, 48381]}, {"Fips"=48067, "FipsAdj"=[5091, 22017, 48037, 48067, 48315]}, {"Fips"=48069, "FipsAdj"=[48069, 48117, 48189, 48279, 48369, 48381]}, {"Fips"=48071, "FipsAdj"=[48071, 48167, 48201, 48245]}, {"Fips"=48073, "FipsAdj"=[48001, 48005, 48073, 48213, 48225, 48347, 48401]}, {"Fips"=48075, "FipsAdj"=[40057, 48075, 48087, 48101, 48191]}, {"Fips"=48077, "FipsAdj"=[40033, 40067, 48009, 48077, 48237, 48337]}, {"Fips"=48079, "FipsAdj"=[35025, 35041, 48017, 48079, 48219, 48279, 48445]}, {"Fips"=48081, "FipsAdj"=[48081, 48335, 48353, 48399, 48431]}, {"Fips"=48083, "FipsAdj"=[48049, 48059, 48083, 48095, 48307, 48399]}, {"Fips"=48085, "FipsAdj"=[48085, 48113, 48121, 48147, 48181, 48231]}, {"Fips"=48087, "FipsAdj"=[40009, 40057, 48075, 48087, 48129, 48179, 48191]}, {"Fips"=48089, "FipsAdj"=[48015, 48089, 48149, 48239, 48285]}, {"Fips"=48091, "FipsAdj"=[48029, 48031, 48091, 48187, 48209]}, {"Fips"=48093, "FipsAdj"=[48049, 48093, 48133, 48143, 48193]}, {"Fips"=48095, "FipsAdj"=[48083, 48095, 48307, 48327, 48399, 48413]}, {"Fips"=48097, "FipsAdj"=[40085, 48097, 48121, 48181, 48337]}, {"Fips"=48099, "FipsAdj"=[48027, 48035, 48099, 48193, 48281]}, {"Fips"=48101, "FipsAdj"=[48075, 48101, 48125, 48155, 48191, 48197, 48269]}, {"Fips"=48103, "FipsAdj"=[48103, 48105, 48135, 48371, 48461]}, {"Fips"=48105, "FipsAdj"=[48103, 48105, 48235, 48371, 48383, 48413, 48435, 48443, 48461]}, {"Fips"=48107, "FipsAdj"=[48107, 48125, 48153, 48169, 48189, 48263, 48303, 48305]}, {"Fips"=48109, "FipsAdj"=[35015, 35035, 48109, 48229, 48243]}, {"Fips"=48111, "FipsAdj"=[35059, 40025, 48111, 48205, 48341]}, {"Fips"=48113, "FipsAdj"=[48085, 48113, 48121, 48139, 48257, 48397]}, {"Fips"=48115, "FipsAdj"=[48033, 48115, 48165, 48227, 48305, 48317]}, {"Fips"=48117, "FipsAdj"=[35009, 35037, 48069, 48117, 48359, 48369, 48375]}, {"Fips"=48119, "FipsAdj"=[48119, 48147, 48159, 48223, 48231, 48277]}, {"Fips"=48121, "FipsAdj"=[48085, 48097, 48113, 48121, 48181, 48439]}, {"Fips"=48123, "FipsAdj"=[48123, 48175, 48177, 48255, 48285]}, {"Fips"=48125, "FipsAdj"=[48101, 48107, 48125, 48153, 48169, 48263, 48269, 48345]}, {"Fips"=48127, "FipsAdj"=[48127, 48163, 48283, 48323, 48479]}, {"Fips"=48129, "FipsAdj"=[48011, 48045, 48065, 48087, 48129, 48179, 48191]}, {"Fips"=48131, "FipsAdj"=[48047, 48131, 48247, 48249, 48283, 48297, 48311]}, {"Fips"=48133, "FipsAdj"=[48049, 48059, 48093, 48133, 48143, 48363, 48417]}, {"Fips"=48135, "FipsAdj"=[48003, 48103, 48135, 48329, 48461, 48475]}, {"Fips"=48137, "FipsAdj"=[48137, 48265, 48267, 48271, 48385, 48435, 48463]}, {"Fips"=48139, "FipsAdj"=[48113, 48139, 48213, 48217, 48251, 48257, 48349]}, {"Fips"=48141, "FipsAdj"=[35013, 35035, 48141]}, {"Fips"=48143, "FipsAdj"=[48035, 48093, 48133, 48143, 48193, 48221, 48363]}, {"Fips"=48145, "FipsAdj"=[48027, 48145, 48293, 48309, 48331]}, {"Fips"=48147, "FipsAdj"=[40013, 48085, 48119, 48147, 48181, 48231]}, {"Fips"=48149, "FipsAdj"=[48015, 48021, 48055, 48089, 48149, 48177, 48285, 48287]}, {"Fips"=48151, "FipsAdj"=[48151, 48253, 48263, 48335, 48353, 48415, 48433]}, {"Fips"=48153, "FipsAdj"=[48045, 48107, 48125, 48153, 48189, 48303, 48345]}, {"Fips"=48155, "FipsAdj"=[48023, 48101, 48155, 48197, 48269, 48275]}, {"Fips"=48157, "FipsAdj"=[48015, 48039, 48157, 48201, 48473]}, {"Fips"=48159, "FipsAdj"=[48063, 48119, 48159, 48223, 48387, 48449]}, {"Fips"=48161, "FipsAdj"=[48001, 48161, 48213, 48289, 48293]}, {"Fips"=48163, "FipsAdj"=[48013, 48127, 48163, 48283, 48325, 48463]}, {"Fips"=48165, "FipsAdj"=[35025, 48003, 48115, 48165, 48317, 48445]}, {"Fips"=48167, "FipsAdj"=[48039, 48071, 48167]}, {"Fips"=48169, "FipsAdj"=[48033, 48107, 48125, 48169, 48263, 48303, 48305]}, {"Fips"=48171, "FipsAdj"=[48031, 48171, 48259, 48265, 48267, 48299]}, {"Fips"=48173, "FipsAdj"=[48173, 48227, 48317, 48329, 48383, 48431]}, {"Fips"=48175, "FipsAdj"=[48025, 48123, 48175, 48255, 48391]}, {"Fips"=48177, "FipsAdj"=[48055, 48123, 48149, 48177, 48187, 48255, 48285]}, {"Fips"=48179, "FipsAdj"=[48011, 48065, 48087, 48129, 48179, 48211, 48393]}, {"Fips"=48181, "FipsAdj"=[40013, 40085, 40095, 48085, 48097, 48121, 48147]}, {"Fips"=48183, "FipsAdj"=[48183, 48203, 48401, 48423]}, {"Fips"=48185, "FipsAdj"=[48041, 48185, 48313, 48339, 48471, 48473]}, {"Fips"=48187, "FipsAdj"=[48029, 48055, 48091, 48177, 48187, 48209]}, {"Fips"=48189, "FipsAdj"=[48069, 48107, 48153, 48189, 48219, 48279, 48303]}, {"Fips"=48191, "FipsAdj"=[48045, 48075, 48087, 48101, 48129, 48191]}, {"Fips"=48193, "FipsAdj"=[48035, 48093, 48099, 48143, 48193, 48281]}, {"Fips"=48195, "FipsAdj"=[40139, 48195, 48233, 48341, 48357, 48393]}, {"Fips"=48197, "FipsAdj"=[40057, 40065, 48075, 48101, 48155, 48197]}, {"Fips"=48199, "FipsAdj"=[48199, 48241, 48245, 48291, 48361, 48373]}, {"Fips"=48201, "FipsAdj"=[48039, 48071, 48157, 48167, 48201, 48291, 48339]}, {"Fips"=48203, "FipsAdj"=[22017, 48183, 48203, 48315, 48365, 48401]}, {"Fips"=48205, "FipsAdj"=[35037, 35059, 48111, 48205, 48341, 48359]}, {"Fips"=48207, "FipsAdj"=[48023, 48207, 48253, 48269, 48275, 48417, 48433]}, {"Fips"=48209, "FipsAdj"=[48031, 48055, 48091, 48187, 48209]}, {"Fips"=48211, "FipsAdj"=[40045, 40129, 48179, 48211, 48295, 48393]}, {"Fips"=48213, "FipsAdj"=[48001, 48073, 48139, 48161, 48213, 48257, 48349, 48423]}, {"Fips"=48215, "FipsAdj"=[48047, 48061, 48215, 48261, 48427]}, {"Fips"=48217, "FipsAdj"=[48035, 48139, 48217, 48251, 48293, 48309]}, {"Fips"=48219, "FipsAdj"=[48017, 48079, 48189, 48219, 48279, 48303, 48305, 48445]}, {"Fips"=48221, "FipsAdj"=[48143, 48221, 48251, 48363, 48367]}, {"Fips"=48223, "FipsAdj"=[48119, 48159, 48223, 48231, 48379]}, {"Fips"=48225, "FipsAdj"=[48001, 48005, 48073, 48225, 48289, 48313, 48455]}, {"Fips"=48227, "FipsAdj"=[48033, 48115, 48173, 48227, 48317, 48335]}, {"Fips"=48229, "FipsAdj"=[35035, 48109, 48141, 48229, 48243]}, {"Fips"=48231, "FipsAdj"=[48085, 48119, 48147, 48223, 48231, 48257, 48379, 48397]}, {"Fips"=48233, "FipsAdj"=[48065, 48195, 48233, 48341, 48393]}, {"Fips"=48235, "FipsAdj"=[48105, 48235, 48383, 48413]}, {"Fips"=48237, "FipsAdj"=[48009, 48077, 48237, 48337, 48363, 48367, 48497]}, {"Fips"=48239, "FipsAdj"=[48057, 48089, 48239, 48285, 48321, 48469]}, {"Fips"=48241, "FipsAdj"=[48005, 48199, 48241, 48351, 48361, 48403, 48405]}, {"Fips"=48243, "FipsAdj"=[48043, 48109, 48229, 48243, 48371, 48377]}, {"Fips"=48245, "FipsAdj"=[22023, 48071, 48199, 48245, 48291]}, {"Fips"=48247, "FipsAdj"=[48047, 48131, 48247, 48427, 48479]}, {"Fips"=48249, "FipsAdj"=[48047, 48131, 48249, 48273, 48297, 48355]}, {"Fips"=48251, "FipsAdj"=[48035, 48139, 48217, 48221, 48251, 48367, 48425]}, {"Fips"=48253, "FipsAdj"=[48059, 48151, 48207, 48253, 48353, 48417, 48433]}, {"Fips"=48255, "FipsAdj"=[48013, 48025, 48123, 48175, 48177, 48255, 48297]}, {"Fips"=48257, "FipsAdj"=[48113, 48139, 48213, 48231, 48257, 48397]}, {"Fips"=48259, "FipsAdj"=[48019, 48029, 48031, 48091, 48171, 48259]}, {"Fips"=48261, "FipsAdj"=[48047, 48215, 48261, 48273]}, {"Fips"=48263, "FipsAdj"=[48107, 48125, 48151, 48169, 48263, 48269, 48415]}, {"Fips"=48265, "FipsAdj"=[48019, 48137, 48171, 48259, 48265, 48267]}, {"Fips"=48267, "FipsAdj"=[48137, 48171, 48265, 48267, 48319, 48327, 48413]}, {"Fips"=48269, "FipsAdj"=[48101, 48125, 48155, 48207, 48263, 48269, 48275, 48345]}, {"Fips"=48271, "FipsAdj"=[48137, 48271, 48323, 48463, 48465]}, {"Fips"=48273, "FipsAdj"=[48047, 48249, 48261, 48273]}, {"Fips"=48275, "FipsAdj"=[48023, 48155, 48207, 48269, 48275, 48433]}, {"Fips"=48277, "FipsAdj"=[40013, 40023, 48119, 48147, 48277]}, {"Fips"=48279, "FipsAdj"=[48017, 48069, 48079, 48189, 48219, 48279, 48303]}, {"Fips"=48281, "FipsAdj"=[48027, 48053, 48099, 48193, 48281, 48333]}, {"Fips"=48283, "FipsAdj"=[48013, 48127, 48131, 48163, 48283, 48311]}, {"Fips"=48285, "FipsAdj"=[48089, 48123, 48149, 48177, 48239, 48285]}, {"Fips"=48287, "FipsAdj"=[48021, 48051, 48149, 48287, 48331, 48477]}, {"Fips"=48289, "FipsAdj"=[48001, 48041, 48161, 48225, 48289, 48293, 48313]}, {"Fips"=48291, "FipsAdj"=[48071, 48199, 48201, 48245, 48291, 48339, 48373]}, {"Fips"=48293, "FipsAdj"=[48145, 48161, 48217, 48289, 48293, 48309, 48349]}, {"Fips"=48295, "FipsAdj"=[40007, 40045, 48211, 48295, 48357]}, {"Fips"=48297, "FipsAdj"=[48013, 48025, 48131, 48249, 48255, 48297, 48311]}, {"Fips"=48299, "FipsAdj"=[48031, 48053, 48171, 48299, 48319]}, {"Fips"=48301, "FipsAdj"=[35015, 35025, 48301, 48389, 48475]}, {"Fips"=48303, "FipsAdj"=[48107, 48153, 48169, 48189, 48219, 48279, 48303, 48305]}, {"Fips"=48305, "FipsAdj"=[48033, 48107, 48115, 48169, 48219, 48303, 48305]}, {"Fips"=48307, "FipsAdj"=[48049, 48083, 48095, 48307, 48319, 48327]}, {"Fips"=48309, "FipsAdj"=[48027, 48035, 48099, 48145, 48217, 48293]}, {"Fips"=48311, "FipsAdj"=[48013, 48131, 48283, 48297, 48311]}, {"Fips"=48313, "FipsAdj"=[48041, 48185, 48225, 48289, 48313, 48395]}, {"Fips"=48315, "FipsAdj"=[22017, 48067, 48203, 48315, 48343]}, {"Fips"=48317, "FipsAdj"=[48003, 48033, 48115, 48165, 48173, 48227, 48317]}, {"Fips"=48319, "FipsAdj"=[48171, 48267, 48299, 48307, 48319, 48327]}, {"Fips"=48321, "FipsAdj"=[48039, 48057, 48239, 48321]}, {"Fips"=48323, "FipsAdj"=[48127, 48271, 48323, 48463, 48479]}, {"Fips"=48325, "FipsAdj"=[48013, 48019, 48029, 48163, 48325, 48463]}, {"Fips"=48327, "FipsAdj"=[48095, 48267, 48307, 48319, 48327, 48413, 48435]}, {"Fips"=48329, "FipsAdj"=[48003, 48135, 48173, 48317, 48329, 48383]}, {"Fips"=48331, "FipsAdj"=[48027, 48051, 48145, 48287, 48331, 48395]}, {"Fips"=48333, "FipsAdj"=[48049, 48093, 48193, 48281, 48333]}, {"Fips"=48335, "FipsAdj"=[48033, 48081, 48151, 48227, 48335, 48353, 48415]}, {"Fips"=48337, "FipsAdj"=[40067, 40085, 48077, 48097, 48237, 48337]}, {"Fips"=48339, "FipsAdj"=[48185, 48201, 48291, 48339, 48407, 48471]}, {"Fips"=48341, "FipsAdj"=[48065, 48111, 48195, 48205, 48233, 48341, 48359, 48375]}, {"Fips"=48343, "FipsAdj"=[48037, 48063, 48067, 48315, 48343, 48387, 48449]}, {"Fips"=48345, "FipsAdj"=[48045, 48101, 48107, 48125, 48153, 48191, 48269]}, {"Fips"=48347, "FipsAdj"=[48005, 48073, 48347, 48401, 48405]}, {"Fips"=48349, "FipsAdj"=[48139, 48161, 48213, 48217, 48293]}, {"Fips"=48351, "FipsAdj"=[22011, 22019, 22085, 22115, 48241, 48351, 48361]}, {"Fips"=48353, "FipsAdj"=[48081, 48151, 48253, 48335, 48353, 48399, 48415]}, {"Fips"=48355, "FipsAdj"=[48007, 48249, 48273, 48355]}, {"Fips"=48357, "FipsAdj"=[40007, 40139, 48195, 48295, 48357]}, {"Fips"=48359, "FipsAdj"=[35037, 48117, 48205, 48341, 48359, 48375]}, {"Fips"=48361, "FipsAdj"=[22019, 22023, 48199, 48241, 48245, 48351]}, {"Fips"=48363, "FipsAdj"=[48133, 48143, 48221, 48237, 48363, 48367, 48429]}, {"Fips"=48365, "FipsAdj"=[22017, 22031, 48203, 48365, 48401]}, {"Fips"=48367, "FipsAdj"=[48221, 48237, 48251, 48363, 48367, 48439]}, {"Fips"=48369, "FipsAdj"=[35009, 48017, 48069, 48117, 48279]}, {"Fips"=48371, "FipsAdj"=[48043, 48103, 48105, 48243, 48371, 48389, 48443]}, {"Fips"=48373, "FipsAdj"=[48005, 48199, 48291, 48373, 48407, 48455]}, {"Fips"=48375, "FipsAdj"=[48011, 48065, 48117, 48341, 48359, 48375]}, {"Fips"=48377, "FipsAdj"=[48043, 48229, 48243]}, {"Fips"=48379, "FipsAdj"=[48223, 48231, 48379, 48467]}, {"Fips"=48381, "FipsAdj"=[48011, 48065, 48069, 48117, 48359, 48375, 48381]}, {"Fips"=48383, "FipsAdj"=[48105, 48173, 48235, 48329, 48383, 48431, 48451]}, {"Fips"=48385, "FipsAdj"=[48019, 48137, 48265, 48385]}, {"Fips"=48387, "FipsAdj"=[40023, 40089, 48037, 48119, 48159, 48277, 48343, 48387]}, {"Fips"=48389, "FipsAdj"=[35015, 48109, 48243, 48301, 48371, 48389]}, {"Fips"=48391, "FipsAdj"=[48007, 48025, 48057, 48175, 48391, 48409]}, {"Fips"=48393, "FipsAdj"=[48065, 48179, 48195, 48211, 48233, 48295, 48357, 48393]}, {"Fips"=48395, "FipsAdj"=[48041, 48051, 48145, 48289, 48293, 48313, 48331]}, {"Fips"=48397, "FipsAdj"=[48085, 48113, 48231, 48257]}, {"Fips"=48399, "FipsAdj"=[48081, 48083, 48095, 48353, 48399, 48441]}, {"Fips"=48401, "FipsAdj"=[48073, 48183, 48203, 48347, 48365, 48401, 48419]}, {"Fips"=48403, "FipsAdj"=[22085, 48241, 48351, 48403, 48405]}, {"Fips"=48405, "FipsAdj"=[48005, 48241, 48347, 48403, 48405]}, {"Fips"=48407, "FipsAdj"=[48291, 48339, 48373, 48407, 48455]}, {"Fips"=48409, "FipsAdj"=[48007, 48025, 48249, 48297, 48355, 48391]}, {"Fips"=48411, "FipsAdj"=[48049, 48053, 48281, 48299, 48307, 48319, 48333]}, {"Fips"=48413, "FipsAdj"=[48095, 48105, 48235, 48267, 48327, 48413, 48435]}, {"Fips"=48415, "FipsAdj"=[48033, 48151, 48169, 48263, 48335, 48353]}, {"Fips"=48417, "FipsAdj"=[48059, 48133, 48207, 48253, 48417, 48429]}, {"Fips"=48419, "FipsAdj"=[22031, 22085, 48347, 48365, 48401, 48403, 48405]}, {"Fips"=48421, "FipsAdj"=[40025, 40139, 48111, 48195, 48205, 48233, 48341]}, {"Fips"=48423, "FipsAdj"=[48073, 48183, 48213, 48401, 48423, 48459, 48467]}, {"Fips"=48425, "FipsAdj"=[48035, 48143, 48221, 48251]}, {"Fips"=48427, "FipsAdj"=[48047, 48215, 48247, 48427]}, {"Fips"=48429, "FipsAdj"=[48133, 48363, 48417, 48429, 48447]}, {"Fips"=48431, "FipsAdj"=[48081, 48173, 48227, 48335, 48383, 48431]}, {"Fips"=48433, "FipsAdj"=[48125, 48151, 48207, 48253, 48263, 48269, 48275]}, {"Fips"=48435, "FipsAdj"=[48105, 48137, 48267, 48327, 48413, 48435]}, {"Fips"=48437, "FipsAdj"=[48011, 48045, 48069, 48153, 48189, 48381]}, {"Fips"=48439, "FipsAdj"=[48113, 48121, 48139, 48251, 48367, 48439]}, {"Fips"=48441, "FipsAdj"=[48059, 48083, 48151, 48253, 48353, 48399]}, {"Fips"=48443, "FipsAdj"=[48043, 48105, 48371, 48443]}, {"Fips"=48445, "FipsAdj"=[48079, 48115, 48165, 48219, 48303, 48305, 48445]}, {"Fips"=48447, "FipsAdj"=[48009, 48023, 48207, 48275, 48417, 48429, 48447]}, {"Fips"=48449, "FipsAdj"=[48063, 48159, 48343, 48387]}, {"Fips"=48451, "FipsAdj"=[48081, 48095, 48235, 48327, 48383, 48399, 48413, 48431]}, {"Fips"=48453, "FipsAdj"=[48021, 48031, 48053, 48055, 48209, 48453]}, {"Fips"=48455, "FipsAdj"=[48005, 48225, 48373, 48407, 48455]}, {"Fips"=48457, "FipsAdj"=[48005, 48199, 48241, 48373]}, {"Fips"=48459, "FipsAdj"=[48063, 48183, 48203, 48315, 48343, 48423, 48459]}, {"Fips"=48461, "FipsAdj"=[48103, 48105, 48135, 48173, 48329, 48383]}, {"Fips"=48463, "FipsAdj"=[48019, 48137, 48163, 48271, 48323, 48325, 48385, 48463]}, {"Fips"=48465, "FipsAdj"=[48105, 48137, 48271, 48435, 48443]}, {"Fips"=48467, "FipsAdj"=[48213, 48231, 48257, 48379, 48423, 48467]}, {"Fips"=48469, "FipsAdj"=[48057, 48123, 48175, 48239, 48285, 48391]}, {"Fips"=48471, "FipsAdj"=[48185, 48225, 48313, 48339, 48407, 48455]}, {"Fips"=48473, "FipsAdj"=[48015, 48157, 48185, 48201, 48339, 48473]}, {"Fips"=48475, "FipsAdj"=[48103, 48135, 48301, 48371, 48389, 48475]}, {"Fips"=48477, "FipsAdj"=[48015, 48041, 48051, 48149, 48185, 48287, 48473]}, {"Fips"=48479, "FipsAdj"=[48127, 48131, 48247, 48283, 48311, 48323, 48479]}, {"Fips"=48481, "FipsAdj"=[48015, 48039, 48089, 48157, 48239, 48321]}, {"Fips"=48483, "FipsAdj"=[40009, 40129, 48087, 48129, 48179, 48211, 48393]}, {"Fips"=48485, "FipsAdj"=[40033, 40141, 48009, 48023, 48077, 48485]}, {"Fips"=48487, "FipsAdj"=[40065, 40141, 48009, 48023, 48155, 48197, 48485]}, {"Fips"=48489, "FipsAdj"=[48061, 48215, 48261]}, {"Fips"=48491, "FipsAdj"=[48021, 48027, 48053, 48287, 48331, 48453]}, {"Fips"=48493, "FipsAdj"=[48013, 48029, 48177, 48187, 48255]}, {"Fips"=48495, "FipsAdj"=[35025, 48003, 48135, 48301, 48475]}, {"Fips"=48497, "FipsAdj"=[48097, 48121, 48237, 48337, 48367, 48439]}, {"Fips"=48499, "FipsAdj"=[48063, 48159, 48223, 48379, 48423, 48459, 48467]}, {"Fips"=48501, "FipsAdj"=[35025, 48079, 48165, 48219, 48445]}, {"Fips"=48503, "FipsAdj"=[48009, 48023, 48237, 48363, 48429, 48447]}, {"Fips"=48505, "FipsAdj"=[48247, 48427, 48479]}, {"Fips"=48507, "FipsAdj"=[48127, 48163, 48271, 48323, 48325, 48463]}, {"Fips"=49001, "FipsAdj"=[32017, 49001, 49017, 49021, 49027, 49031]}, {"Fips"=49003, "FipsAdj"=[16031, 16071, 32007, 49003, 49005, 49011, 49045]}, {"Fips"=49005, "FipsAdj"=[16007, 16041, 16071, 49003, 49005, 49033]}, {"Fips"=49007, "FipsAdj"=[49007, 49013, 49015, 49039, 49047]}, {"Fips"=49009, "FipsAdj"=[8081, 49009, 49013, 49043, 49047]}, {"Fips"=49011, "FipsAdj"=[49003, 49011, 49029, 49035, 49045]}, {"Fips"=49013, "FipsAdj"=[49007, 49009, 49013, 49043, 49047, 49049]}, {"Fips"=49015, "FipsAdj"=[49007, 49015, 49019, 49037, 49039, 49041, 49047]}, {"Fips"=49017, "FipsAdj"=[49001, 49017, 49021, 49025, 49031, 49037]}, {"Fips"=49019, "FipsAdj"=[8045, 8077, 8085, 49015, 49019, 49037, 49047]}, {"Fips"=49021, "FipsAdj"=[32017, 49001, 49017, 49021, 49025]}, {"Fips"=49023, "FipsAdj"=[32033, 49023, 49027, 49039, 49045]}, {"Fips"=49025, "FipsAdj"=[4005, 4015, 49017, 49021, 49025, 49037]}, {"Fips"=49027, "FipsAdj"=[32017, 32033, 49001, 49023, 49027, 49039]}, {"Fips"=49029, "FipsAdj"=[49011, 49029, 49033, 49035, 49043]}, {"Fips"=49031, "FipsAdj"=[49001, 49017, 49031, 49041]}, {"Fips"=49033, "FipsAdj"=[16007, 16041, 49005, 49029, 49033, 49043, 49057, 56023]}, {"Fips"=49035, "FipsAdj"=[49011, 49029, 49035, 49043, 49045, 49049]}, {"Fips"=49037, "FipsAdj"=[4001, 4005, 4017, 8033, 8077, 8083, 8085, 8113, 35045, 49015, 49017, 49019, 49025, 49037]}, {"Fips"=49039, "FipsAdj"=[49007, 49015, 49023, 49027, 49039, 49041]}, {"Fips"=49041, "FipsAdj"=[49001, 49015, 49027, 49031, 49039, 49041]}, {"Fips"=49043, "FipsAdj"=[49009, 49013, 49029, 49033, 49035, 49043, 49051, 56037]}, {"Fips"=49045, "FipsAdj"=[32007, 32033, 49003, 49011, 49023, 49035, 49045, 49049]}, {"Fips"=49047, "FipsAdj"=[8045, 8081, 8103, 49007, 49009, 49013, 49015, 49019]}, {"Fips"=49049, "FipsAdj"=[49007, 49013, 49023, 49035, 49039, 49045, 49049]}, {"Fips"=49051, "FipsAdj"=[49013, 49035, 49043, 49049]}, {"Fips"=49053, "FipsAdj"=[4015, 32017, 49021, 49025]}, {"Fips"=49055, "FipsAdj"=[49015, 49017, 49019, 49031, 49037, 49041]}, {"Fips"=49057, "FipsAdj"=[49003, 49005, 49011, 49029, 49033, 49045]}, {"Fips"=50001, "FipsAdj"=[36031, 36115, 50001, 50007, 50017, 50021, 50023]}, {"Fips"=50003, "FipsAdj"=[25003, 25011, 36083, 36115, 50003, 50021, 50025]}, {"Fips"=50005, "FipsAdj"=[33009, 50005, 50009, 50015, 50017, 50019]}, {"Fips"=50007, "FipsAdj"=[36019, 36031, 50001, 50007, 50011, 50013, 50015]}, {"Fips"=50009, "FipsAdj"=[33007, 33009, 50005, 50009]}, {"Fips"=50011, "FipsAdj"=[50007, 50011, 50013, 50015]}, {"Fips"=50013, "FipsAdj"=[36019, 50007, 50011]}, {"Fips"=50015, "FipsAdj"=[50005, 50007, 50011, 50015, 50019]}, {"Fips"=50017, "FipsAdj"=[33009, 50001, 50005, 50017, 50023]}, {"Fips"=50019, "FipsAdj"=[50005, 50009, 50011, 50015]}, {"Fips"=50021, "FipsAdj"=[36115, 50001, 50003, 50021]}, {"Fips"=50023, "FipsAdj"=[50001, 50005, 50007, 50015, 50017]}, {"Fips"=50025, "FipsAdj"=[25011, 33005, 33019, 50003, 50025]}, {"Fips"=50027, "FipsAdj"=[33009, 33019, 50001, 50003, 50017, 50021, 50025]}, {"Fips"=51001, "FipsAdj"=[24039, 24047, 51001, 51103, 51115, 51119, 51131]}, {"Fips"=51003, "FipsAdj"=[51003, 51015, 51029, 51065, 51079, 51109, 51125, 51137, 51165]}, {"Fips"=51005, "FipsAdj"=[51005, 51017, 51023, 51045, 51163, 51580, 54025]}, {"Fips"=51007, "FipsAdj"=[51007, 51041, 51049, 51053, 51135, 51145]}, {"Fips"=51009, "FipsAdj"=[51009, 51011, 51019, 51031, 51125, 51163]}, {"Fips"=51011, "FipsAdj"=[51009, 51011, 51029, 51031, 51037, 51125]}, {"Fips"=51013, "FipsAdj"=[11001, 24031, 51013, 51059, 51510]}, {"Fips"=51015, "FipsAdj"=[51003, 51015, 51017, 51091, 51125, 51163, 51165, 51790, 51820]}, {"Fips"=51017, "FipsAdj"=[51005, 51015, 51017, 51091, 51163, 54025]}, {"Fips"=51019, "FipsAdj"=[51009, 51019, 51023, 51031, 51067, 51143, 51161, 51163, 51515]}, {"Fips"=51021, "FipsAdj"=[51021, 51071, 51155, 51173, 51185, 51197]}, {"Fips"=51023, "FipsAdj"=[51005, 51019, 51023, 51045, 51161]}, {"Fips"=51025, "FipsAdj"=[37131, 37185, 51025, 51053, 51081, 51111, 51117]}, {"Fips"=51027, "FipsAdj"=[21195, 51027, 51051, 51167, 51185, 54047]}, {"Fips"=51029, "FipsAdj"=[51003, 51011, 51029, 51049, 51065, 51125]}, {"Fips"=51031, "FipsAdj"=[51009, 51011, 51019, 51031, 51037, 51083, 51143]}, {"Fips"=51033, "FipsAdj"=[51033, 51057, 51085, 51097, 51099, 51101, 51177]}, {"Fips"=51035, "FipsAdj"=[37171, 51035, 51063, 51077, 51141, 51155, 51197]}, {"Fips"=51036, "FipsAdj"=[51036, 51041, 51087, 51095, 51127, 51149]}, {"Fips"=51037, "FipsAdj"=[51011, 51031, 51037, 51083, 51111, 51117]}, {"Fips"=51041, "FipsAdj"=[51007, 51036, 51041, 51053, 51075, 51087, 51145, 51149, 51570, 51670, 51730]}, {"Fips"=51043, "FipsAdj"=[51043, 51061, 51069, 51107, 51187, 54003]}, {"Fips"=51045, "FipsAdj"=[51005, 51023, 51045, 51071, 51121, 51161]}, {"Fips"=51047, "FipsAdj"=[51047, 51061, 51113, 51137, 51157, 51177]}, {"Fips"=51049, "FipsAdj"=[51007, 51029, 51049, 51065, 51075, 51145]}, {"Fips"=51051, "FipsAdj"=[21195, 51027, 51051, 51167]}, {"Fips"=51053, "FipsAdj"=[51007, 51025, 51041, 51053, 51081, 51135, 51149, 51183]}, {"Fips"=51057, "FipsAdj"=[51033, 51057, 51097, 51099, 51103, 51119, 51159]}, {"Fips"=51059, "FipsAdj"=[11001, 24017, 24031, 24033, 51013, 51059, 51107, 51153, 51510, 51600]}, {"Fips"=51061, "FipsAdj"=[51043, 51047, 51061, 51107, 51153, 51157, 51179]}, {"Fips"=51063, "FipsAdj"=[51035, 51063, 51067, 51121, 51141, 51155]}, {"Fips"=51065, "FipsAdj"=[51003, 51029, 51049, 51065, 51075]}, {"Fips"=51067, "FipsAdj"=[51019, 51063, 51067, 51089, 51141, 51143]}, {"Fips"=51069, "FipsAdj"=[51043, 51069, 51171, 51187, 51840, 54003, 54027, 54031, 54037]}, {"Fips"=51071, "FipsAdj"=[51021, 51045, 51071, 51121, 51155, 54055, 54063]}, {"Fips"=51073, "FipsAdj"=[51073, 51095, 51097, 51115, 51119]}, {"Fips"=51075, "FipsAdj"=[51041, 51049, 51065, 51075, 51085, 51087, 51109]}, {"Fips"=51077, "FipsAdj"=[37005, 37009, 37171, 47091, 51035, 51077, 51173, 51191, 51197]}, {"Fips"=51079, "FipsAdj"=[51003, 51079, 51113, 51137, 51139]}, {"Fips"=51081, "FipsAdj"=[37131, 51025, 51053, 51081, 51175, 51183]}, {"Fips"=51083, "FipsAdj"=[37033, 37077, 37145, 51031, 51037, 51083, 51117]}, {"Fips"=51085, "FipsAdj"=[51033, 51075, 51085, 51087, 51101, 51109, 51127]}, {"Fips"=51087, "FipsAdj"=[51036, 51041, 51075, 51085, 51087, 51127, 51145]}, {"Fips"=51089, "FipsAdj"=[37157, 37169, 51067, 51089, 51141, 51143]}, {"Fips"=51091, "FipsAdj"=[51015, 51017, 51091, 54071]}, {"Fips"=51093, "FipsAdj"=[51093, 51095, 51175, 51181, 51620, 51700]}, {"Fips"=51095, "FipsAdj"=[51036, 51073, 51093, 51095, 51097, 51127, 51181, 51199, 51700]}, {"Fips"=51097, "FipsAdj"=[51033, 51057, 51073, 51095, 51097, 51101, 51119]}, {"Fips"=51099, "FipsAdj"=[24017, 51033, 51057, 51099, 51179]}, {"Fips"=51101, "FipsAdj"=[51033, 51085, 51097, 51101]}, {"Fips"=51103, "FipsAdj"=[51001, 51057, 51103, 51119, 51133]}, {"Fips"=51105, "FipsAdj"=[21013, 21095, 47025, 47067, 51105, 51169]}, {"Fips"=51107, "FipsAdj"=[24021, 24031, 24043, 51043, 51059, 51061, 51107, 51153]}, {"Fips"=51109, "FipsAdj"=[51003, 51065, 51075, 51085, 51109, 51137]}, {"Fips"=51111, "FipsAdj"=[51025, 51037, 51111, 51117, 51135]}, {"Fips"=51113, "FipsAdj"=[51047, 51079, 51113, 51137, 51139]}, {"Fips"=51115, "FipsAdj"=[51001, 51073, 51115, 51119, 51131]}, {"Fips"=51117, "FipsAdj"=[37077, 37181, 37185, 51025, 51037, 51083, 51111]}, {"Fips"=51119, "FipsAdj"=[51001, 51057, 51073, 51097, 51103, 51115, 51119, 51131]}, {"Fips"=51121, "FipsAdj"=[51045, 51063, 51071, 51121, 51155, 51161]}, {"Fips"=51125, "FipsAdj"=[51003, 51009, 51011, 51015, 51029, 51125]}, {"Fips"=51127, "FipsAdj"=[51036, 51085, 51087, 51095, 51097, 51101]}, {"Fips"=51131, "FipsAdj"=[51001, 51115, 51119, 51131, 51199, 51650, 51710, 51735]}, {"Fips"=51133, "FipsAdj"=[24037, 24039, 51001, 51103, 51133, 51159]}, {"Fips"=51135, "FipsAdj"=[51007, 51025, 51053, 51111, 51135]}, {"Fips"=51137, "FipsAdj"=[51003, 51047, 51079, 51109, 51113, 51137]}, {"Fips"=51139, "FipsAdj"=[51079, 51113, 51139, 51157, 51165, 51171]}, {"Fips"=51141, "FipsAdj"=[37169, 37171, 51035, 51063, 51067, 51089]}, {"Fips"=51143, "FipsAdj"=[37033, 37157, 51019, 51031, 51067, 51083, 51089, 51143]}, {"Fips"=51145, "FipsAdj"=[51007, 51041, 51049, 51075, 51087]}, {"Fips"=51147, "FipsAdj"=[51007, 51011, 51029, 51037, 51049, 51111, 51135]}, {"Fips"=51149, "FipsAdj"=[51036, 51041, 51053, 51149, 51181, 51183, 51670]}, {"Fips"=51153, "FipsAdj"=[24017, 51059, 51061, 51107, 51153, 51179, 51683]}, {"Fips"=51155, "FipsAdj"=[51021, 51035, 51063, 51071, 51121, 51155, 51197]}, {"Fips"=51157, "FipsAdj"=[51047, 51061, 51113, 51139, 51157]}, {"Fips"=51159, "FipsAdj"=[51057, 51103, 51119, 51133, 51159]}, {"Fips"=51161, "FipsAdj"=[51019, 51023, 51045, 51063, 51067, 51121, 51161, 51770]}, {"Fips"=51163, "FipsAdj"=[51005, 51009, 51015, 51017, 51019, 51023, 51125, 51163, 51530]}, {"Fips"=51165, "FipsAdj"=[51003, 51015, 51079, 51139, 51165, 51171, 51660, 54031]}, {"Fips"=51167, "FipsAdj"=[51027, 51051, 51167, 51169, 51173, 51185, 51191]}, {"Fips"=51169, "FipsAdj"=[47067, 47073, 47163, 51105, 51167, 51169, 51191]}, {"Fips"=51171, "FipsAdj"=[51069, 51139, 51165, 51171, 51187]}, {"Fips"=51173, "FipsAdj"=[51021, 51077, 51167, 51173, 51185, 51191]}, {"Fips"=51175, "FipsAdj"=[37073, 37091, 37131, 51081, 51093, 51175, 51181, 51183, 51620]}, {"Fips"=51177, "FipsAdj"=[51033, 51047, 51085, 51109, 51137, 51177, 51179]}, {"Fips"=51179, "FipsAdj"=[24017, 51033, 51047, 51061, 51099, 51153, 51177, 51179]}, {"Fips"=51181, "FipsAdj"=[51036, 51093, 51095, 51149, 51175, 51181, 51183]}, {"Fips"=51183, "FipsAdj"=[51053, 51081, 51149, 51175, 51181]}, {"Fips"=51185, "FipsAdj"=[51021, 51027, 51167, 51173, 51185, 54047]}, {"Fips"=51187, "FipsAdj"=[51043, 51061, 51069, 51139, 51157, 51171]}, {"Fips"=51191, "FipsAdj"=[47091, 47163, 51077, 51167, 51169, 51173, 51191]}, {"Fips"=51193, "FipsAdj"=[24017, 24037, 51057, 51099, 51133, 51159]}, {"Fips"=51195, "FipsAdj"=[21095, 21133, 21195, 51051, 51105, 51167, 51169, 51195]}, {"Fips"=51197, "FipsAdj"=[51021, 51035, 51077, 51155, 51173]}, {"Fips"=51199, "FipsAdj"=[51073, 51095, 51115, 51131, 51199, 51650, 51700, 51735]}, {"Fips"=51510, "FipsAdj"=[11001, 24033, 51013, 51059]}, {"Fips"=51515, "FipsAdj"=[51019]}, {"Fips"=51520, "FipsAdj"=[47163, 51191]}, {"Fips"=51530, "FipsAdj"=[51163]}, {"Fips"=51540, "FipsAdj"=[51003]}, {"Fips"=51550, "FipsAdj"=[37029, 37053, 51550, 51710, 51740, 51800]}, {"Fips"=51570, "FipsAdj"=[51041, 51570]}, {"Fips"=51580, "FipsAdj"=[51005]}, {"Fips"=51590, "FipsAdj"=[37033, 51143]}, {"Fips"=51595, "FipsAdj"=[51081]}, {"Fips"=51600, "FipsAdj"=[51059]}, {"Fips"=51610, "FipsAdj"=[51013, 51059]}, {"Fips"=51620, "FipsAdj"=[51093, 51175]}, {"Fips"=51630, "FipsAdj"=[51177, 51179]}, {"Fips"=51640, "FipsAdj"=[51035, 51077]}, {"Fips"=51650, "FipsAdj"=[51131, 51199, 51650, 51700, 51710, 51735, 51740]}, {"Fips"=51660, "FipsAdj"=[51165]}, {"Fips"=51670, "FipsAdj"=[51041, 51149]}, {"Fips"=51678, "FipsAdj"=[51163]}, {"Fips"=51680, "FipsAdj"=[51009, 51019, 51031]}, {"Fips"=51683, "FipsAdj"=[51153, 51683]}, {"Fips"=51685, "FipsAdj"=[51153, 51683]}, {"Fips"=51690, "FipsAdj"=[51089]}, {"Fips"=51700, "FipsAdj"=[51093, 51095, 51181, 51199, 51650, 51700, 51740]}, {"Fips"=51710, "FipsAdj"=[51131, 51550, 51650, 51710, 51740]}, {"Fips"=51720, "FipsAdj"=[51195]}, {"Fips"=51730, "FipsAdj"=[51041, 51053, 51149, 51570]}, {"Fips"=51735, "FipsAdj"=[51131, 51199, 51650]}, {"Fips"=51740, "FipsAdj"=[51550, 51650, 51700, 51710, 51740]}, {"Fips"=51750, "FipsAdj"=[51121, 51155]}, {"Fips"=51760, "FipsAdj"=[51041, 51087]}, {"Fips"=51770, "FipsAdj"=[51161, 51770]}, {"Fips"=51775, "FipsAdj"=[51161, 51770]}, {"Fips"=51790, "FipsAdj"=[51015]}, {"Fips"=51800, "FipsAdj"=[37029, 37073, 51093, 51175, 51550, 51700, 51740]}, {"Fips"=51810, "FipsAdj"=[37053, 51131, 51550, 51650, 51710]}, {"Fips"=51820, "FipsAdj"=[51015]}, {"Fips"=51830, "FipsAdj"=[51095, 51199]}, {"Fips"=51840, "FipsAdj"=[51069]}, {"Fips"=53001, "FipsAdj"=[53001, 53021, 53025, 53043]}, {"Fips"=53003, "FipsAdj"=[16069, 41063, 53003, 53023]}, {"Fips"=53005, "FipsAdj"=[41049, 41059, 53005, 53021, 53025, 53039, 53071]}, {"Fips"=53007, "FipsAdj"=[53007, 53017, 53033, 53037, 53047, 53057]}, {"Fips"=53009, "FipsAdj"=[53009, 53031]}, {"Fips"=53011, "FipsAdj"=[41009, 41051, 53011, 53015]}, {"Fips"=53013, "FipsAdj"=[41059, 41063, 53013, 53021, 53023, 53071]}, {"Fips"=53015, "FipsAdj"=[41009, 53011, 53015, 53041, 53059]}, {"Fips"=53017, "FipsAdj"=[53007, 53017, 53025, 53037]}, {"Fips"=53019, "FipsAdj"=[53019, 53043, 53047]}, {"Fips"=53021, "FipsAdj"=[53001, 53005, 53013, 53021, 53025, 53071]}, {"Fips"=53023, "FipsAdj"=[41063, 53003, 53013, 53023]}, {"Fips"=53025, "FipsAdj"=[53001, 53005, 53017, 53021, 53025, 53037, 53043, 53047]}, {"Fips"=53027, "FipsAdj"=[53027, 53031, 53041, 53045, 53049]}, {"Fips"=53029, "FipsAdj"=[53029, 53031, 53035, 53055, 53057]}, {"Fips"=53031, "FipsAdj"=[53009, 53027, 53029, 53031, 53035, 53045]}, {"Fips"=53033, "FipsAdj"=[53007, 53033, 53035, 53037, 53053, 53061]}, {"Fips"=53035, "FipsAdj"=[53029, 53031, 53033, 53035, 53045, 53053]}, {"Fips"=53037, "FipsAdj"=[53007, 53017, 53025, 53033, 53037, 53053]}, {"Fips"=53039, "FipsAdj"=[41021, 41027, 41049, 41055, 41065, 53005, 53039, 53059]}, {"Fips"=53041, "FipsAdj"=[53015, 53027, 53041, 53049, 53053, 53059, 53067, 53069]}, {"Fips"=53043, "FipsAdj"=[53001, 53019, 53025, 53043, 53047, 53063, 53065]}, {"Fips"=53045, "FipsAdj"=[53027, 53031, 53035, 53045, 53053]}, {"Fips"=53047, "FipsAdj"=[53007, 53017, 53019, 53025, 53043, 53047, 53057]}, {"Fips"=53049, "FipsAdj"=[41007, 53027, 53041, 53049]}, {"Fips"=53051, "FipsAdj"=[16017, 16021, 53051, 53063]}, {"Fips"=53053, "FipsAdj"=[53033, 53035, 53037, 53041, 53045, 53053, 53067]}, {"Fips"=53055, "FipsAdj"=[53009, 53029, 53031, 53055, 53057]}, {"Fips"=53057, "FipsAdj"=[53007, 53029, 53047, 53055, 53057, 53061]}, {"Fips"=53059, "FipsAdj"=[41027, 41051, 53011, 53015, 53039, 53041, 53059]}, {"Fips"=53061, "FipsAdj"=[53007, 53029, 53033, 53035, 53057]}, {"Fips"=53063, "FipsAdj"=[16009, 16017, 16055, 53043, 53051, 53063, 53065]}, {"Fips"=53065, "FipsAdj"=[53019, 53043, 53051, 53063]}, {"Fips"=53067, "FipsAdj"=[53027, 53041, 53045, 53053]}, {"Fips"=53069, "FipsAdj"=[41007, 41009, 53015, 53041, 53049]}, {"Fips"=53071, "FipsAdj"=[41059, 53005, 53013, 53021]}, {"Fips"=53073, "FipsAdj"=[53047, 53055, 53057]}, {"Fips"=53075, "FipsAdj"=[16009, 16057, 16069, 53001, 53003, 53013, 53021, 53023, 53043, 53063]}, {"Fips"=53077, "FipsAdj"=[53005, 53025, 53033, 53037, 53039, 53041, 53053, 53059]}, {"Fips"=54001, "FipsAdj"=[54001, 54033, 54077, 54083, 54091, 54093]}, {"Fips"=54003, "FipsAdj"=[24043, 51043, 51069, 54003, 54037]}, {"Fips"=54005, "FipsAdj"=[54005, 54039, 54043, 54045, 54081]}, {"Fips"=54007, "FipsAdj"=[54007, 54013, 54015, 54021, 54041, 54067]}, {"Fips"=54009, "FipsAdj"=[39081, 42125, 54009, 54029]}, {"Fips"=54011, "FipsAdj"=[39053, 39087, 54011, 54043, 54053, 54079]}, {"Fips"=54013, "FipsAdj"=[54007, 54013, 54015, 54021, 54085, 54087]}, {"Fips"=54015, "FipsAdj"=[54007, 54013, 54015, 54039, 54067]}, {"Fips"=54017, "FipsAdj"=[54017, 54021, 54033, 54041, 54085, 54095]}, {"Fips"=54019, "FipsAdj"=[54019, 54025, 54039, 54067, 54081]}, {"Fips"=54021, "FipsAdj"=[54007, 54013, 54017, 54021, 54041]}, {"Fips"=54023, "FipsAdj"=[24023, 54023, 54027, 54031, 54057, 54071, 54077, 54083]}, {"Fips"=54025, "FipsAdj"=[51005, 51017, 54019, 54025, 54063, 54067, 54075, 54089]}, {"Fips"=54027, "FipsAdj"=[24001, 51069, 54023, 54027, 54031, 54057]}, {"Fips"=54029, "FipsAdj"=[39029, 39081, 42007, 42125, 54009]}, {"Fips"=54031, "FipsAdj"=[51069, 51165, 51171, 54023, 54027, 54031, 54057]}, {"Fips"=54033, "FipsAdj"=[54001, 54017, 54033, 54041, 54049, 54091, 54097]}, {"Fips"=54035, "FipsAdj"=[39105, 54035, 54039, 54053, 54079, 54087, 54105]}, {"Fips"=54037, "FipsAdj"=[24043, 51043, 51069, 51107, 54003]}, {"Fips"=54039, "FipsAdj"=[54005, 54015, 54019, 54035, 54039, 54043, 54067, 54079, 54081]}, {"Fips"=54041, "FipsAdj"=[54007, 54017, 54021, 54033, 54041, 54097]}, {"Fips"=54043, "FipsAdj"=[54005, 54011, 54039, 54043, 54045, 54059, 54079]}, {"Fips"=54045, "FipsAdj"=[54005, 54043, 54045, 54059]}, {"Fips"=54047, "FipsAdj"=[51027, 51185, 54047, 54055, 54059]}, {"Fips"=54049, "FipsAdj"=[54033, 54049, 54061, 54091]}, {"Fips"=54051, "FipsAdj"=[39013, 39111, 42059, 42125, 54051, 54069]}, {"Fips"=54053, "FipsAdj"=[39053, 39105, 54011, 54035, 54053]}, {"Fips"=54055, "FipsAdj"=[51021, 51071, 51185, 54047, 54055, 54081, 54089]}, {"Fips"=54057, "FipsAdj"=[24001, 24023, 54023, 54027, 54031]}, {"Fips"=54059, "FipsAdj"=[21159, 21195, 51027, 54043, 54045, 54047, 54059, 54099]}, {"Fips"=54061, "FipsAdj"=[42051, 42059, 54049, 54061, 54077, 54091]}, {"Fips"=54063, "FipsAdj"=[51005, 51045, 51071, 54025, 54063]}, {"Fips"=54065, "FipsAdj"=[24001, 24043, 51069, 54003, 54027]}, {"Fips"=54067, "FipsAdj"=[54007, 54015, 54019, 54025, 54039, 54067]}, {"Fips"=54069, "FipsAdj"=[39013, 39081, 42125, 54009, 54051]}, {"Fips"=54071, "FipsAdj"=[51015, 51091, 51165, 54023, 54031, 54071, 54075]}, {"Fips"=54073, "FipsAdj"=[39167, 54073, 54085, 54095]}, {"Fips"=54075, "FipsAdj"=[51017, 51091, 54025, 54071, 54075, 54083]}, {"Fips"=54077, "FipsAdj"=[24023, 42051, 54001, 54023, 54061, 54077, 54091]}, {"Fips"=54079, "FipsAdj"=[54011, 54035, 54039, 54043, 54053]}, {"Fips"=54081, "FipsAdj"=[54005, 54019, 54039, 54055, 54081, 54089]}, {"Fips"=54083, "FipsAdj"=[54001, 54023, 54071, 54075, 54083, 54093, 54097]}, {"Fips"=54085, "FipsAdj"=[54013, 54017, 54021, 54073, 54085, 54095, 54105]}, {"Fips"=54087, "FipsAdj"=[54013, 54015, 54035, 54039, 54087]}, {"Fips"=54089, "FipsAdj"=[51071, 54019, 54025, 54055, 54063, 54081]}, {"Fips"=54091, "FipsAdj"=[54001, 54033, 54049, 54061, 54077]}, {"Fips"=54093, "FipsAdj"=[54001, 54023, 54077, 54083]}, {"Fips"=54095, "FipsAdj"=[39111, 39167, 54017, 54073, 54085, 54095]}, {"Fips"=54097, "FipsAdj"=[54001, 54033, 54041, 54083, 54097]}, {"Fips"=54099, "FipsAdj"=[21019, 21127, 21159, 39087, 54011, 54043, 54059]}, {"Fips"=54101, "FipsAdj"=[54007, 54025, 54041, 54067, 54075, 54083, 54097]}, {"Fips"=54103, "FipsAdj"=[39111, 42059, 54017, 54033, 54049, 54051, 54061, 54095]}, {"Fips"=54105, "FipsAdj"=[54013, 54035, 54085, 54087, 54105]}, {"Fips"=54107, "FipsAdj"=[39009, 39105, 39167, 54035, 54073, 54085, 54105]}, {"Fips"=54109, "FipsAdj"=[54005, 54045, 54047, 54055, 54059, 54081]}, {"Fips"=55001, "FipsAdj"=[55001, 55021, 55057, 55077, 55097, 55111, 55137]}, {"Fips"=55003, "FipsAdj"=[26053, 26131, 27031, 27075, 55003, 55007, 55051, 55099]}, {"Fips"=55005, "FipsAdj"=[55005, 55013, 55017, 55033, 55095, 55107, 55109, 55113]}, {"Fips"=55007, "FipsAdj"=[27075, 55003, 55007, 55031, 55113]}, {"Fips"=55009, "FipsAdj"=[55009, 55015, 55029, 55061, 55071, 55083, 55087]}, {"Fips"=55011, "FipsAdj"=[27157, 27169, 55011, 55035, 55091]}, {"Fips"=55013, "FipsAdj"=[27025, 27115, 55005, 55013, 55031, 55095]}, {"Fips"=55015, "FipsAdj"=[55009, 55015, 55039, 55071, 55087, 55117]}, {"Fips"=55017, "FipsAdj"=[55005, 55017, 55019, 55033, 55035, 55107]}, {"Fips"=55019, "FipsAdj"=[55017, 55019, 55035, 55053, 55073, 55119]}, {"Fips"=55021, "FipsAdj"=[55001, 55021, 55025, 55027, 55047, 55057, 55077]}, {"Fips"=55023, "FipsAdj"=[19005, 19043, 55023, 55043, 55103]}, {"Fips"=55025, "FipsAdj"=[55021, 55025, 55027, 55045, 55049, 55055, 55105]}, {"Fips"=55027, "FipsAdj"=[55021, 55025, 55027, 55039, 55047, 55055, 55131]}, {"Fips"=55029, "FipsAdj"=[26019, 26041, 26089, 26109, 55009, 55029, 55061, 55075]}, {"Fips"=55031, "FipsAdj"=[27017, 27075, 27115, 27137, 55007, 55013, 55031, 55113]}, {"Fips"=55033, "FipsAdj"=[55005, 55017, 55033, 55035, 55091, 55093, 55095]}, {"Fips"=55035, "FipsAdj"=[55011, 55017, 55019, 55033, 55035, 55053, 55091]}, {"Fips"=55037, "FipsAdj"=[26043, 26071, 55037, 55041]}, {"Fips"=55039, "FipsAdj"=[55015, 55027, 55039, 55047, 55117, 55131]}, {"Fips"=55041, "FipsAdj"=[26071, 55037, 55041, 55067, 55075, 55083, 55085]}, {"Fips"=55043, "FipsAdj"=[17085, 19043, 19061, 55023, 55043, 55049, 55065]}, {"Fips"=55045, "FipsAdj"=[17177, 17201, 55025, 55045, 55049, 55065]}, {"Fips"=55047, "FipsAdj"=[55021, 55027, 55039, 55047, 55077, 55137]}, {"Fips"=55049, "FipsAdj"=[55025, 55043, 55045, 55049, 55065, 55103]}, {"Fips"=55051, "FipsAdj"=[26053, 55003, 55051, 55099]}, {"Fips"=55053, "FipsAdj"=[55019, 55035, 55053, 55057, 55063, 55081, 55121]}, {"Fips"=55055, "FipsAdj"=[55025, 55027, 55055, 55105, 55127]}, {"Fips"=55057, "FipsAdj"=[55001, 55021, 55053, 55057, 55081, 55111, 55123]}, {"Fips"=55059, "FipsAdj"=[17097, 17111, 26005, 55059, 55101]}, {"Fips"=55061, "FipsAdj"=[26019, 26101, 55009, 55029, 55061]}, {"Fips"=55063, "FipsAdj"=[27055, 27169, 55053, 55063, 55081, 55121]}, {"Fips"=55065, "FipsAdj"=[17085, 17177, 55043, 55045, 55049]}, {"Fips"=55067, "FipsAdj"=[55041, 55067, 55069, 55073, 55078, 55083, 55085]}, {"Fips"=55069, "FipsAdj"=[55067, 55069, 55073, 55085, 55099]}, {"Fips"=55071, "FipsAdj"=[26101, 26105, 55009, 55015, 55061, 55071]}, {"Fips"=55073, "FipsAdj"=[55019, 55067, 55069, 55073, 55097, 55115, 55119, 55135]}, {"Fips"=55075, "FipsAdj"=[26043, 26109, 55029, 55037, 55041, 55075]}, {"Fips"=55077, "FipsAdj"=[55001, 55021, 55047, 55077]}, {"Fips"=55078, "FipsAdj"=[55067, 55078, 55083]}, {"Fips"=55079, "FipsAdj"=[26121, 26139, 55079, 55089, 55101, 55131]}, {"Fips"=55081, "FipsAdj"=[55053, 55057, 55063, 55081]}, {"Fips"=55083, "FipsAdj"=[55009, 55029, 55041, 55067, 55075, 55078, 55083]}, {"Fips"=55085, "FipsAdj"=[55041, 55067, 55069, 55085, 55099]}, {"Fips"=55087, "FipsAdj"=[55009, 55015, 55087, 55115, 55135]}, {"Fips"=55089, "FipsAdj"=[26121, 26127, 55079, 55089, 55117, 55131]}, {"Fips"=55091, "FipsAdj"=[27049, 27157, 55011, 55033, 55035, 55091]}, {"Fips"=55093, "FipsAdj"=[27037, 27049, 27163, 55033, 55091, 55093]}, {"Fips"=55095, "FipsAdj"=[27025, 27163, 55005, 55013, 55033, 55095]}, {"Fips"=55097, "FipsAdj"=[55001, 55073, 55097, 55115, 55135, 55137]}, {"Fips"=55099, "FipsAdj"=[55003, 55051, 55069, 55085, 55099, 55107, 55113, 55119]}, {"Fips"=55101, "FipsAdj"=[26005, 26139, 55059, 55079, 55101, 55127]}, {"Fips"=55103, "FipsAdj"=[55023, 55043, 55049, 55103, 55111]}, {"Fips"=55105, "FipsAdj"=[17007, 17201, 55025, 55045, 55055, 55105]}, {"Fips"=55107, "FipsAdj"=[55005, 55017, 55099, 55107, 55113, 55119]}, {"Fips"=55109, "FipsAdj"=[27163, 55005, 55033, 55093, 55095]}, {"Fips"=55111, "FipsAdj"=[55001, 55021, 55025, 55049, 55057, 55103, 55111]}, {"Fips"=55113, "FipsAdj"=[55003, 55005, 55007, 55031, 55099, 55107, 55113]}, {"Fips"=55115, "FipsAdj"=[55009, 55067, 55073, 55078, 55083, 55087, 55097, 55115]}, {"Fips"=55117, "FipsAdj"=[26105, 26127, 55015, 55039, 55071, 55089, 55117]}, {"Fips"=55119, "FipsAdj"=[55017, 55019, 55069, 55073, 55099, 55107]}, {"Fips"=55121, "FipsAdj"=[27169, 55011, 55035, 55053, 55063]}, {"Fips"=55123, "FipsAdj"=[19005, 27055, 55023, 55057, 55063, 55081, 55103, 55111]}, {"Fips"=55125, "FipsAdj"=[26053, 26071, 55041, 55051, 55085, 55099]}, {"Fips"=55127, "FipsAdj"=[17007, 17111, 55055, 55059, 55101, 55105, 55127]}, {"Fips"=55129, "FipsAdj"=[55005, 55007, 55013, 55031, 55107, 55113]}, {"Fips"=55131, "FipsAdj"=[55027, 55039, 55079, 55089, 55117, 55131]}, {"Fips"=55133, "FipsAdj"=[55027, 55055, 55079, 55089, 55101, 55127, 55131]}, {"Fips"=55135, "FipsAdj"=[55073, 55087, 55097, 55115, 55135, 55137]}, {"Fips"=55137, "FipsAdj"=[55001, 55047, 55077, 55097, 55135, 55137]}, {"Fips"=55139, "FipsAdj"=[55015, 55039, 55047, 55087, 55135, 55137]}, {"Fips"=55141, "FipsAdj"=[55001, 55019, 55053, 55057, 55073, 55097]}, {"Fips"=56001, "FipsAdj"=[8057, 8069, 56001, 56007, 56009, 56021]}, {"Fips"=56003, "FipsAdj"=[30003, 30009, 56003, 56019, 56029, 56033]}, {"Fips"=56005, "FipsAdj"=[30075, 56005, 56009, 56011, 56019, 56033]}, {"Fips"=56007, "FipsAdj"=[8057, 8081, 8107, 56001, 56007, 56009, 56013, 56025]}, {"Fips"=56009, "FipsAdj"=[56001, 56005, 56007, 56009, 56019, 56025, 56027, 56031]}, {"Fips"=56011, "FipsAdj"=[30011, 30075, 46019, 46081, 56005, 56011]}, {"Fips"=56013, "FipsAdj"=[56007, 56013, 56017, 56025, 56029, 56035, 56037, 56039]}, {"Fips"=56015, "FipsAdj"=[31007, 31157, 31165, 56015, 56021, 56027]}, {"Fips"=56017, "FipsAdj"=[56013, 56017, 56029]}, {"Fips"=56019, "FipsAdj"=[56003, 56005, 56009, 56019, 56025, 56033]}, {"Fips"=56021, "FipsAdj"=[8069, 8123, 31007, 31105, 56001, 56015, 56021]}, {"Fips"=56023, "FipsAdj"=[16007, 16019, 16029, 49033, 56023, 56035, 56037, 56039]}, {"Fips"=56025, "FipsAdj"=[56007, 56009, 56013, 56019, 56025]}, {"Fips"=56027, "FipsAdj"=[31165, 46033, 46047, 56009, 56015, 56027, 56031]}, {"Fips"=56029, "FipsAdj"=[30009, 30031, 30067, 56003, 56013, 56017, 56029, 56039]}, {"Fips"=56031, "FipsAdj"=[56001, 56009, 56015, 56021, 56027]}, {"Fips"=56033, "FipsAdj"=[30003, 30075, 56003, 56005, 56019]}, {"Fips"=56035, "FipsAdj"=[56013, 56023, 56035, 56037]}, {"Fips"=56037, "FipsAdj"=[8081, 49009, 49043, 56007, 56013, 56023, 56035, 56037]}, {"Fips"=56039, "FipsAdj"=[16019, 16043, 16081, 30031, 56013, 56023, 56029, 56035]}, {"Fips"=56041, "FipsAdj"=[49033, 49043, 56023, 56037]}, {"Fips"=56043, "FipsAdj"=[56003, 56013, 56017, 56019, 56025, 56029]}, {"Fips"=56045, "FipsAdj"=[46033, 46081, 46103, 56005, 56009, 56011, 56027]}, {"Fips"=72001, "FipsAdj"=[72001, 72059, 72081, 72111, 72113, 72141]}, {"Fips"=72003, "FipsAdj"=[72003, 72005, 72011, 72099]}, {"Fips"=72005, "FipsAdj"=[72003, 72005, 72071]}, {"Fips"=72007, "FipsAdj"=[72007, 72021, 72025, 72041, 72045, 72061]}, {"Fips"=72009, "FipsAdj"=[72009, 72019, 72035, 72041, 72043]}, {"Fips"=72011, "FipsAdj"=[72003, 72011, 72083, 72097, 72099, 72117]}, {"Fips"=72013, "FipsAdj"=[72013, 72017, 72039, 72054, 72065]}, {"Fips"=72015, "FipsAdj"=[72015, 72057]}, {"Fips"=72017, "FipsAdj"=[72013, 72017, 72054]}, {"Fips"=72019, "FipsAdj"=[72009, 72019, 72041, 72043, 72045, 72047, 72105]}, {"Fips"=72021, "FipsAdj"=[72007, 72021, 72033, 72045, 72061, 72105, 72135]}, {"Fips"=72023, "FipsAdj"=[72023, 72067, 72079, 72097]}, {"Fips"=72025, "FipsAdj"=[72007, 72025, 72035, 72041, 72063, 72127, 72129]}, {"Fips"=72027, "FipsAdj"=[72027, 72065, 72081, 72115]}, {"Fips"=72029, "FipsAdj"=[72029, 72031, 72063, 72077, 72085, 72087]}, {"Fips"=72031, "FipsAdj"=[72029, 72031, 72063, 72077, 72087, 72127]}, {"Fips"=72033, "FipsAdj"=[72021, 72033, 72061, 72127]}, {"Fips"=72035, "FipsAdj"=[72009, 72025, 72035, 72041, 72057, 72109, 72123]}, {"Fips"=72037, "FipsAdj"=[72037, 72049, 72053, 72089, 72103, 72119]}, {"Fips"=72039, "FipsAdj"=[72013, 72039, 72054, 72073, 72091, 72101, 72107]}, {"Fips"=72041, "FipsAdj"=[72007, 72009, 72019, 72025, 72035, 72041]}, {"Fips"=72043, "FipsAdj"=[72009, 72019, 72043, 72075, 72107, 72123, 72133]}, {"Fips"=72045, "FipsAdj"=[72007, 72019, 72021, 72041, 72045]}, {"Fips"=72047, "FipsAdj"=[72019, 72047, 72101, 72105, 72107, 72135]}, {"Fips"=72049, "FipsAdj"=[72037]}, {"Fips"=72051, "FipsAdj"=[72051, 72135, 72137]}, {"Fips"=72053, "FipsAdj"=[72037, 72053]}, {"Fips"=72054, "FipsAdj"=[72013, 72017, 72039, 72054]}, {"Fips"=72055, "FipsAdj"=[72055, 72059, 72079, 72121]}, {"Fips"=72057, "FipsAdj"=[72015, 72035, 72057, 72109]}, {"Fips"=72059, "FipsAdj"=[72001, 72055, 72059, 72111]}, {"Fips"=72061, "FipsAdj"=[72007, 72021, 72033, 72061]}, {"Fips"=72063, "FipsAdj"=[72025, 72029, 72031, 72063, 72077, 72129]}, {"Fips"=72065, "FipsAdj"=[72013, 72027, 72065, 72081]}, {"Fips"=72067, "FipsAdj"=[72023, 72067, 72097]}, {"Fips"=72069, "FipsAdj"=[72069, 72085, 72103]}, {"Fips"=72071, "FipsAdj"=[72005, 72071, 72099, 72115]}, {"Fips"=72073, "FipsAdj"=[72039, 72073, 72075, 72107, 72113]}, {"Fips"=72075, "FipsAdj"=[72043, 72073, 72075, 72107, 72113, 72133]}, {"Fips"=72077, "FipsAdj"=[72029, 72031, 72063, 72077, 72085]}, {"Fips"=72079, "FipsAdj"=[72023, 72055, 72079, 72121]}, {"Fips"=72081, "FipsAdj"=[72001, 72027, 72065, 72081, 72083, 72093, 72131, 72141]}, {"Fips"=72083, "FipsAdj"=[72011, 72081, 72083, 72093, 72097]}, {"Fips"=72085, "FipsAdj"=[72029, 72069, 72077, 72085, 72103, 72119, 72129]}, {"Fips"=72087, "FipsAdj"=[72029, 72031, 72087]}, {"Fips"=72089, "FipsAdj"=[72037, 72053, 72089]}, {"Fips"=72091, "FipsAdj"=[72017, 72039, 72054, 72091, 72101, 72143]}, {"Fips"=72093, "FipsAdj"=[72081, 72083, 72093, 72097, 72121, 72125]}, {"Fips"=72095, "FipsAdj"=[72095, 72109]}, {"Fips"=72097, "FipsAdj"=[72011, 72023, 72067, 72083, 72093, 72097, 72117]}, {"Fips"=72099, "FipsAdj"=[72003, 72005, 72011, 72071, 72099]}, {"Fips"=72101, "FipsAdj"=[72039, 72047, 72091, 72101, 72107, 72143]}, {"Fips"=72103, "FipsAdj"=[72037, 72069, 72085, 72103]}, {"Fips"=72105, "FipsAdj"=[72019, 72021, 72045, 72047, 72105]}, {"Fips"=72107, "FipsAdj"=[72019, 72039, 72043, 72047, 72073, 72075, 72101, 72107]}, {"Fips"=72109, "FipsAdj"=[72015, 72035, 72057, 72095, 72109, 72129]}, {"Fips"=72111, "FipsAdj"=[72001, 72059, 72111]}, {"Fips"=72113, "FipsAdj"=[72001, 72073, 72075, 72111, 72113]}, {"Fips"=72115, "FipsAdj"=[72027, 72071, 72115]}, {"Fips"=72117, "FipsAdj"=[72003, 72011, 72097]}, {"Fips"=72119, "FipsAdj"=[72029, 72037, 72085, 72087, 72089, 72103]}, {"Fips"=72121, "FipsAdj"=[72055, 72079, 72093, 72121, 72125]}, {"Fips"=72123, "FipsAdj"=[72009, 72035, 72043, 72057, 72123]}, {"Fips"=72125, "FipsAdj"=[72023, 72067, 72079, 72093, 72097, 72121]}, {"Fips"=72127, "FipsAdj"=[72007, 72025, 72031, 72033, 72061, 72127, 72137]}, {"Fips"=72129, "FipsAdj"=[72025, 72035, 72063, 72077, 72085, 72109, 72129]}, {"Fips"=72131, "FipsAdj"=[72011, 72027, 72071, 72081, 72083, 72099, 72115]}, {"Fips"=72133, "FipsAdj"=[72043, 72075, 72123]}, {"Fips"=72135, "FipsAdj"=[72021, 72047, 72051, 72105, 72135, 72137]}, {"Fips"=72137, "FipsAdj"=[72021, 72033, 72051, 72127, 72135]}, {"Fips"=72139, "FipsAdj"=[72025, 72031, 72063, 72127]}, {"Fips"=72141, "FipsAdj"=[72001, 72013, 72039, 72065, 72073, 72081, 72113]}, {"Fips"=72143, "FipsAdj"=[72047, 72051, 72091, 72101, 72135, 72143]}, {"Fips"=72145, "FipsAdj"=[72091, 72101, 72143]}, {"Fips"=72147, "FipsAdj"=[72037]}, {"Fips"=72149, "FipsAdj"=[72043, 72075, 72107]}, {"Fips"=72151, "FipsAdj"=[72069, 72085, 72095, 72109, 72129]}, {"Fips"=72153, "FipsAdj"=[72001, 72055, 72059, 72081, 72093, 72121]}, {"Fips"=60010, "FipsAdj"=[60010]}, {"Fips"=60020, "FipsAdj"=[]}, {"Fips"=60030, "FipsAdj"=[]}, {"Fips"=60040, "FipsAdj"=[]}, {"Fips"=60050, "FipsAdj"=[60010]}, {"Fips"=66010, "FipsAdj"=[]}, {"Fips"=69085, "FipsAdj"=[]}, {"Fips"=69100, "FipsAdj"=[]}, {"Fips"=69110, "FipsAdj"=[69110]}, {"Fips"=69120, "FipsAdj"=[69110]}, {"Fips"=78010, "FipsAdj"=[]}, {"Fips"=78020, "FipsAdj"=[78020]}] ("Adjaceny") -> [w8]
    tunnel: "FipsIn" -> [w7] mode=indexing
    tunnel: [w6] -> w3 mode=concatenating
    n2 = for {
      tunnel: w8 -> [w13] mode=indexing
      tunnel: w7 -> [w11]
      tunnel: [w9] -> w6
      stop <- w10 stop-if-true
      n3 = Unbundle By Name(w13) -> ("Fips"=w12:i32, "FipsAdj"=w9:i32[])
      n4 = Equal?(x=w11, y=w12) -> (x = y?=w10:bool)
    }
  }
  n5 = Build Array (concatenate)("FipsIn", w3) -> (w1:i32[])
  n6 = call "DeleteDup.vi"("Array in"=w1) -> ("Array out"=→"FipsOut":i32[])  [unwired: 10 in]
